vi "LabVIEW_Ansys.vi"() -> ()   [LabVIEW 2017]
uses:
  <vilib>/imath/engines/lvmath/Plug In/_Char/NIMS_CH_character datatype.ctl
  <vilib>/Utility/file.llb/Read Delimited Spreadsheet (string).vi
  <vilib>/imath/engines/lvmath2/RunTimeEngine/Managers/WorkSpace/UID Generator.vi
  <vilib>/imath/engines/lvmath2/RunTimeEngine/ArithmeticOperatorToken/NIMS_ArithmeticOperator_times.vi
  <instcachedir>/0/NIMS_ArithmeticOperator_times_9BECD6C28351466A83A029AF2762CD58.lvgen/NIMS_ArithmeticOperator_times_9BECD6C28351466A83A029AF2762CD58_000.vi
  <vilib>/imath/engines/lvmath2/RunTimeEngine/ArithmeticOperatorToken/NIMS_ArithmeticOperator_plus.vi
  <instcachedir>/0/NIMS_ArithmeticOperator_plus_9255C7DA94A9479C92F91DC2DA9A664F.lvgen/NIMS_ArithmeticOperator_plus_9255C7DA94A9479C92F91DC2DA9A664F_004.vi
  <vilib>/imath/engines/lvmath2/RunTimeEngine/RunTimeType/NIMS_RunTimeType_From StrictType (excl LVString).vi
  <instcachedir>/0/NIMS_RunTimeType_From StrictType (excl LVString)_1019F277F0A747EDBCA0F6C52CA54500.lvgen/NIMS_RunTimeType_From StrictType (excl LVString)_1019F277F0A747EDBCA0F6C52CA54500_000.vi
  <vilib>/imath/engines/lvmath2/RunTimeEngine/ErrorHandling/NIMS_Create Error From Enums.vi
  <vilib>/imath/engines/lvmath2/RunTimeEngine/LocalVariableDefStatement/MC_LocalVariableDefStatement_Display.vi
  <vilib>/imath/engines/lvmath2/RunTimeEngine/BuiltInFunctions/plot/NIMS_plot(RM, RM, Str).vi
  <vilib>/imathl/engines/lvmath/Functions/Error Handling/Create Error.vi
  <vilib>/imath/engines/lvmath/Plug In/_Char/NIMS_CH_Character RV to String.vi
  <vilib>/imath/engines/lvmath2/RunTimeEngine/BuiltInFunctions/title/NIMS_title.vi
  <vilib>/imath/engines/lvmath2/RunTimeEngine/BuiltInFunctions/xlabel/NIMS_xlabel.vi
  <vilib>/imath/engines/lvmath2/RunTimeEngine/BuiltInFunctions/ylabel/NIMS_ylabel.vi
  <vilib>/imath/engines/lvmath2/RunTimeEngine/Managers/SymbolTable/Clear UID.vi
  <vilib>/imath/engines/lvmath2/RunTimeEngine/ErrorHandling/NIMS_Finalize Error.vi
  <vilib>/imath/engines/lvmath2/RunTimeEngine/Managers/SymbolTable/NIMS_WorkSpace.lvlib
panel:
  in  "定子瞬态":bool
  out "new picture":picture caption="图片展示"
  in  "?":bool
  in  "表面幅仿真-Z方向":bool
  in  "表面幅仿真-Y方向":bool
  in  "关闭图片":bool
  in  "阻抗特性曲线":bool
  in  "计算步数":u32(slide) scale=0.0..100.0
  in  "表面幅仿真-X方向":bool
  in  "16":bool
  in  "波数":dbl
  in  "15":bool
  in  "台阶高":dbl
  in  "14":bool
  in  "压电片外圈直径":dbl
  in  "13":bool
  in  "压电片内圈直径":dbl
  in  "12":bool
  in  "压电片厚":dbl
  in  "11":bool
  in  "轴厚度":dbl
  in  "10":bool
  in  "轴外圈直径":dbl
  in  "9":bool
  in  "轴内圈直径":dbl
  in  "8":bool
  in  "定子齿外圈直径":dbl
  in  "7":bool
  in  "定子齿内圈直径":dbl
  in  "6":bool
  in  "齿槽宽":dbl
  in  "5":bool
  in  "齿厚":dbl
  in  "4":bool
  in  "内侧斜齿高":dbl
  in  "3":bool
  in  "外侧斜齿高":dbl
  in  "2":bool
  in  "平均齿高":dbl
  in  "1":bool
  in  "齿数":dbl
  in  "数值":dbl
  in  "加载图片":bool
  in  "一键删除":bool
  in  "开始ANSYS计算":bool
  in  "存":bool
  in  "前一张":bool
  in  "后一张":bool
  # "电机仿真参数"
  # "计算"
  # "结果"
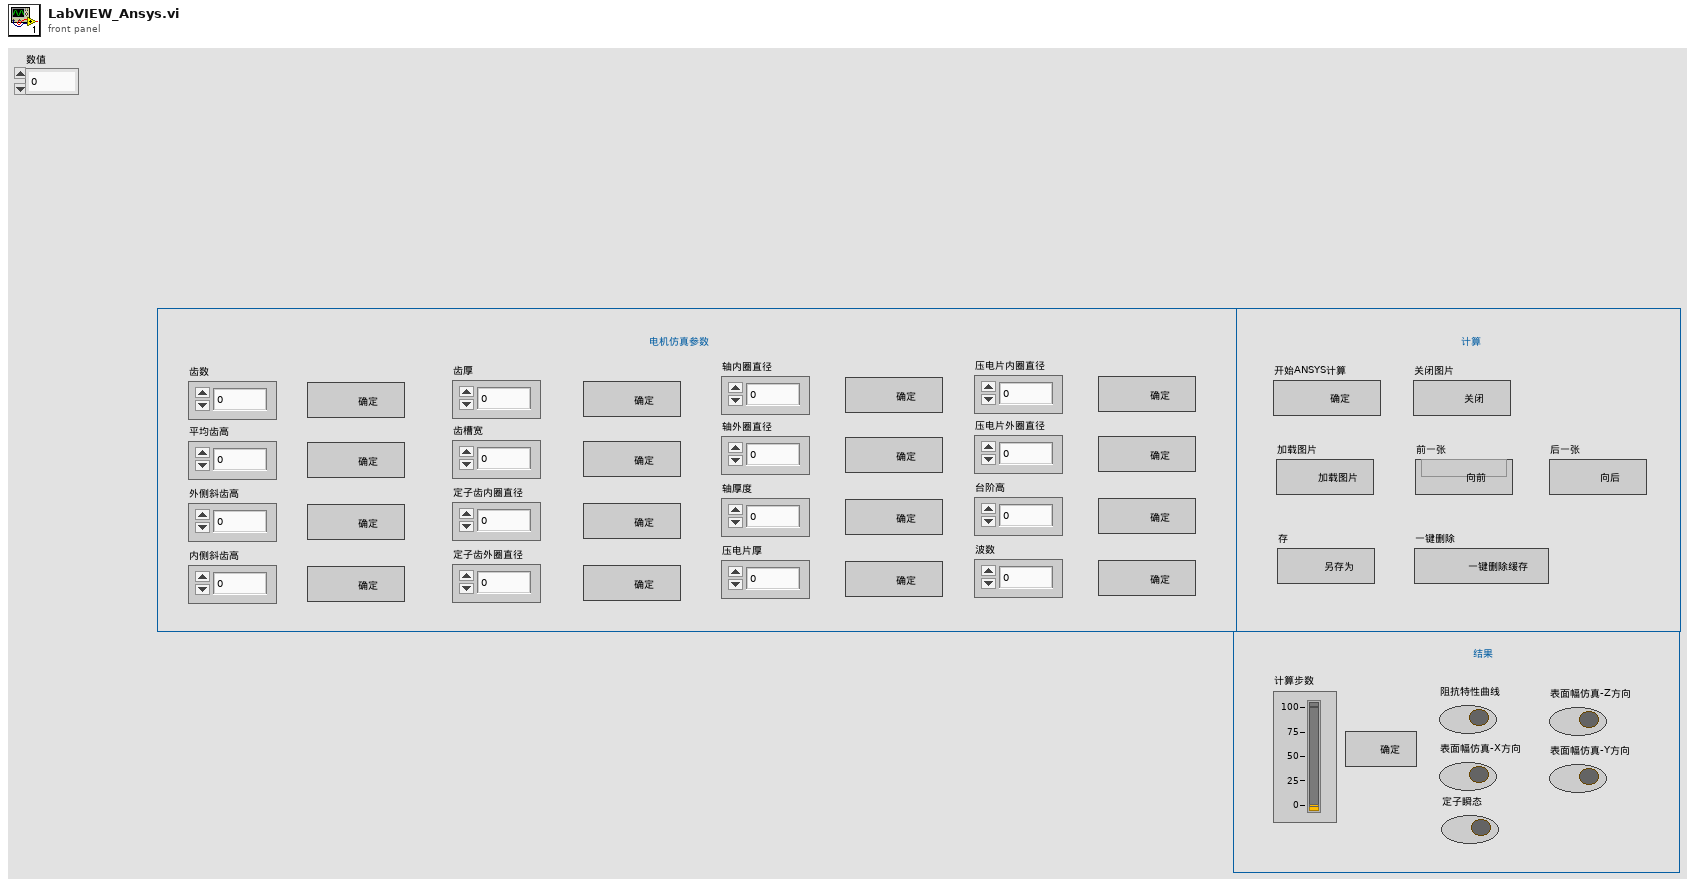
[diagram p1: front panel]
types:
  T1 = enum16{"open", "replace", "create", "open or create", "replace or create", "replace or create with confirmation"}
  T2 = typedef "NIMS_CH_character datatype.ctl" = cluster{"Numeric":u8}
  T3 = typedef "imagedata.ctl" = cluster{"image type":i32, "image depth":i32, "image":u8[], "mask":u8[], "colors":u32[], "Rectangle":cluster{"left":i16, "top":i16, "right":i16, "bottom":i16}}
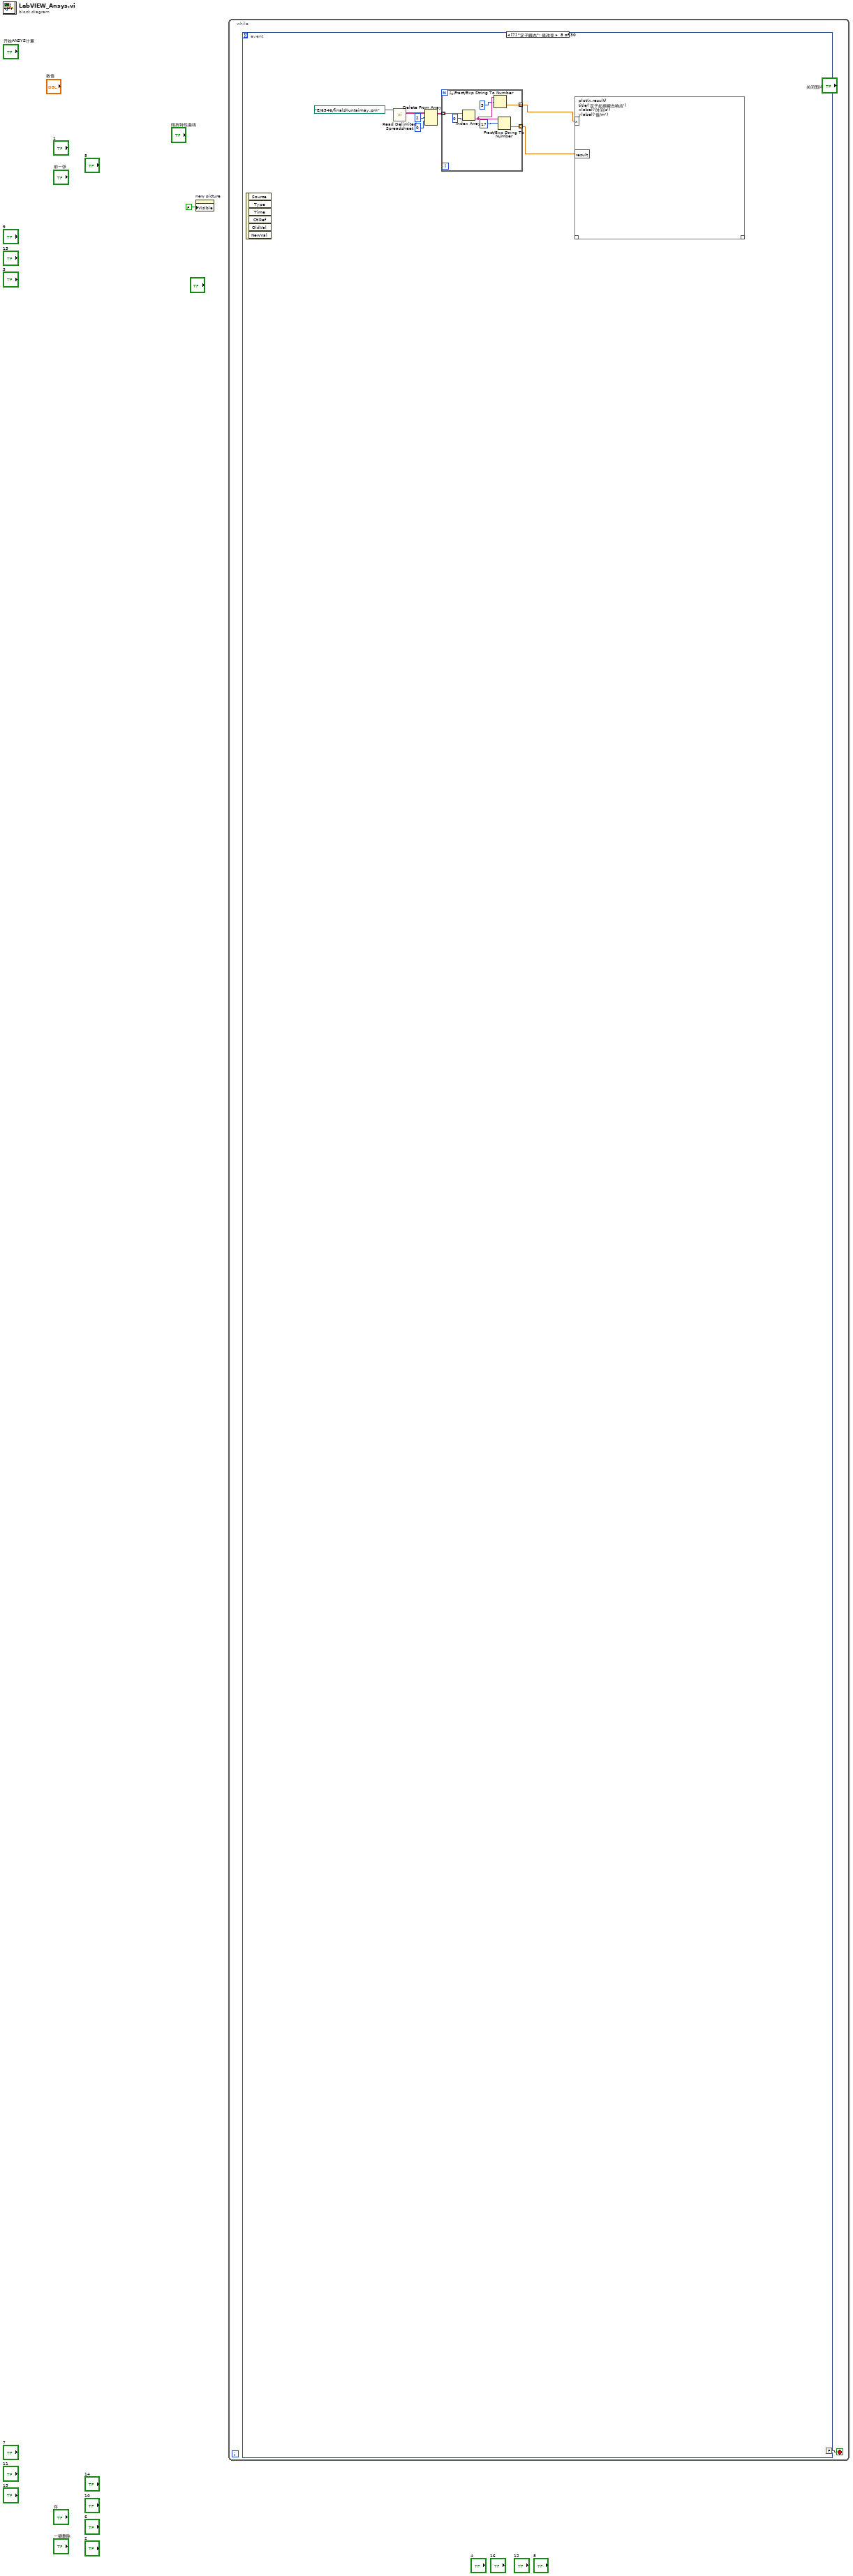
[diagram p0: block diagram]
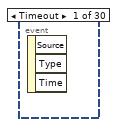
[diagram p2: hidden frame]
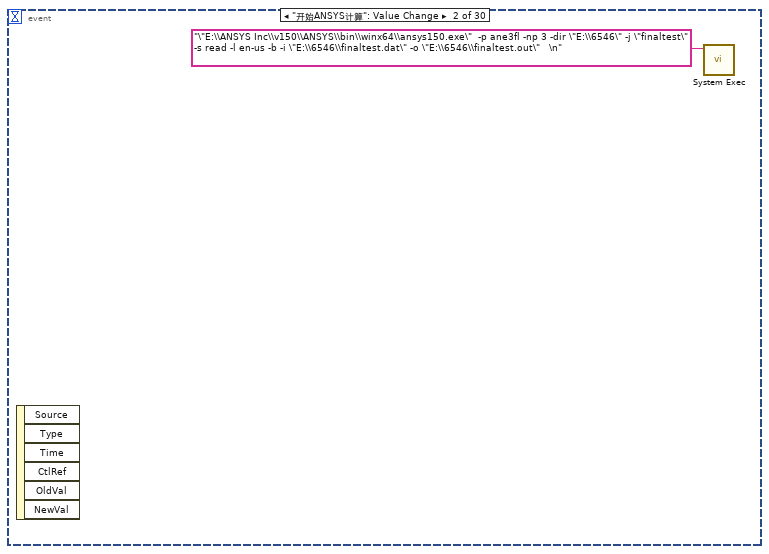
[diagram p3: hidden frame]
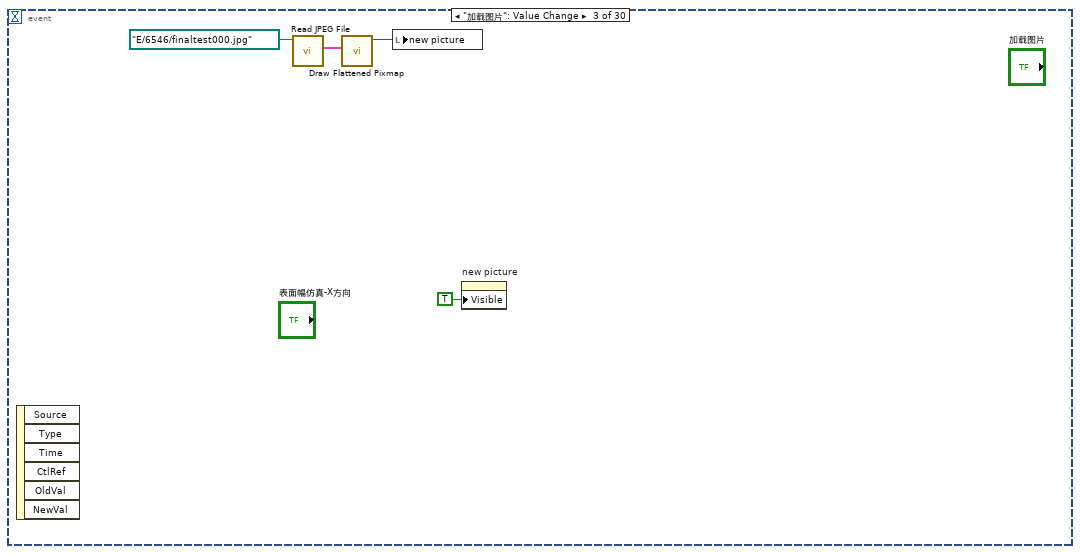
[diagram p4: hidden frame]
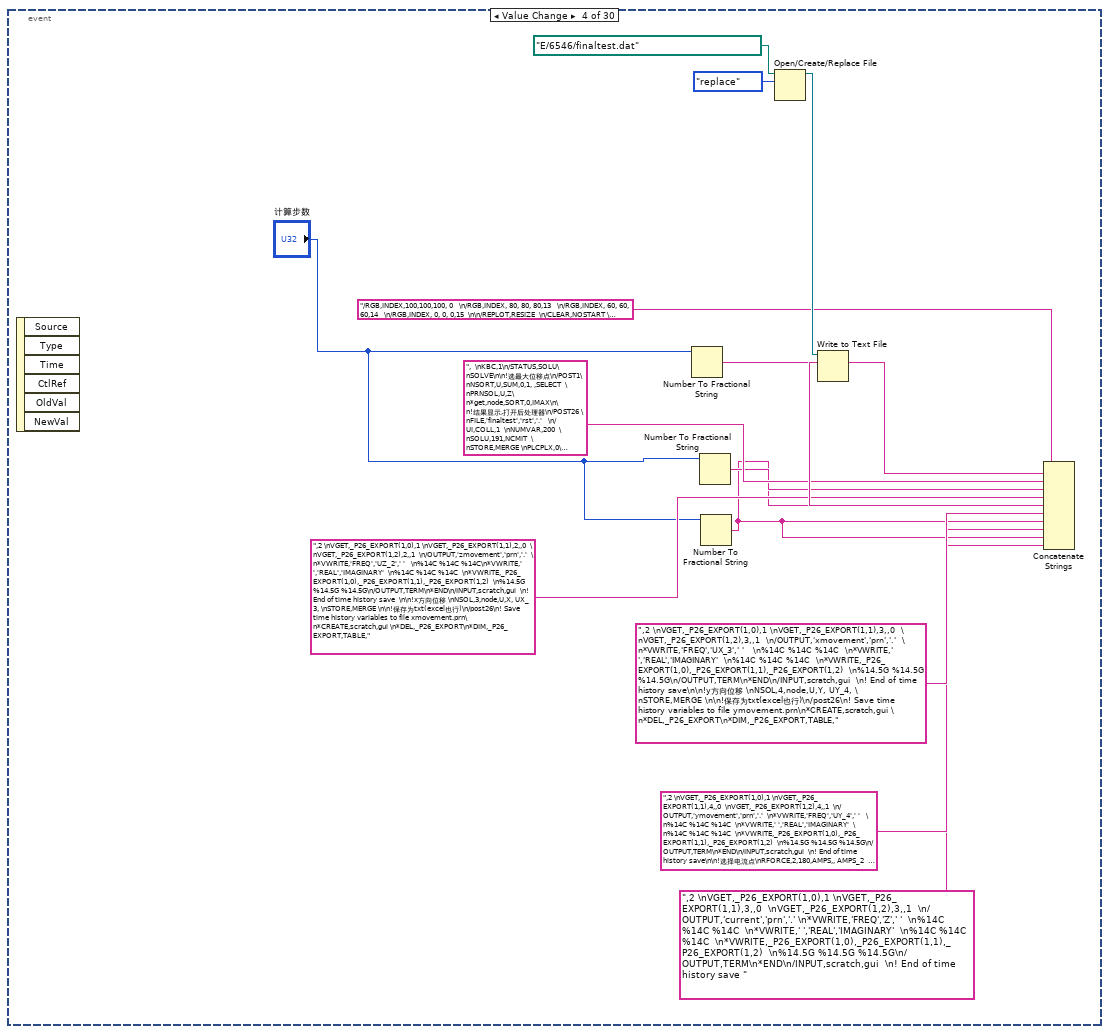
[diagram p5: hidden frame]
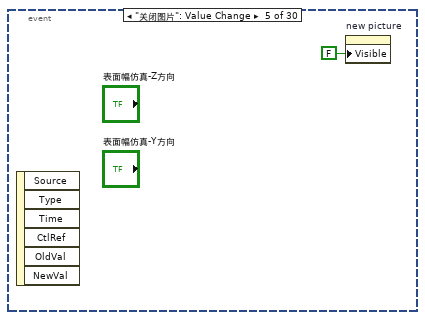
[diagram p6: hidden frame]
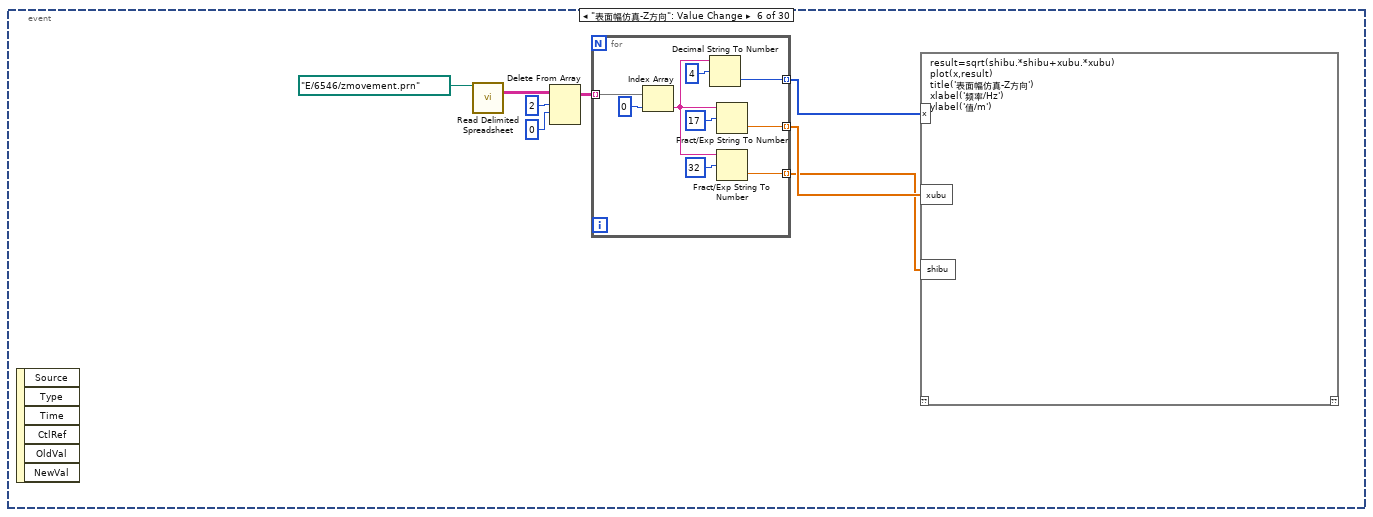
[diagram p7: hidden frame]
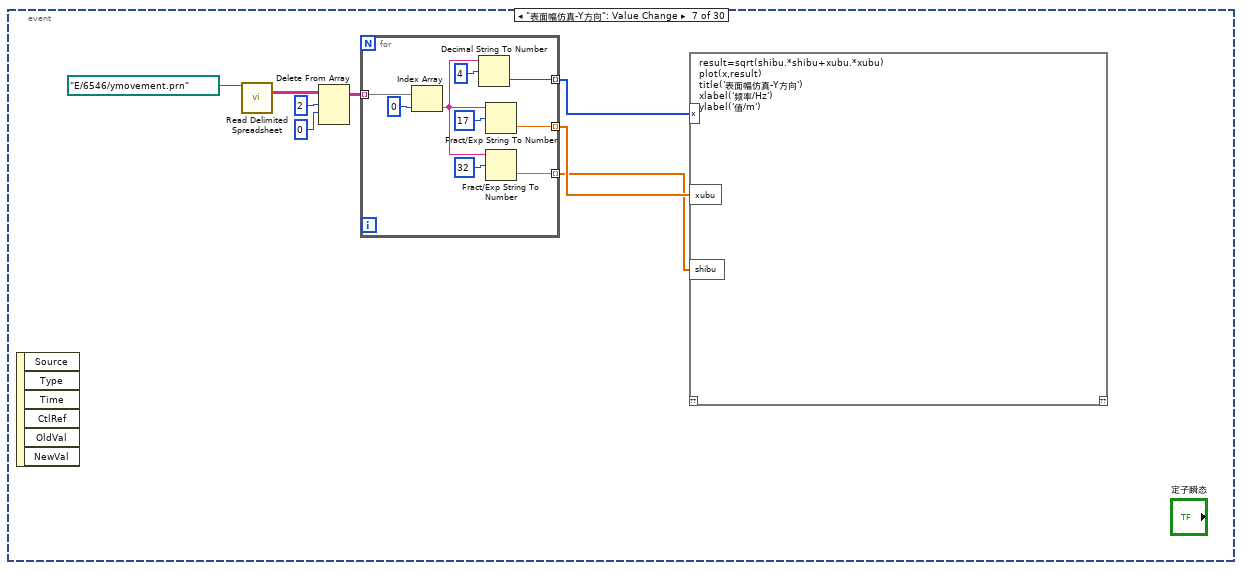
[diagram p8: hidden frame]
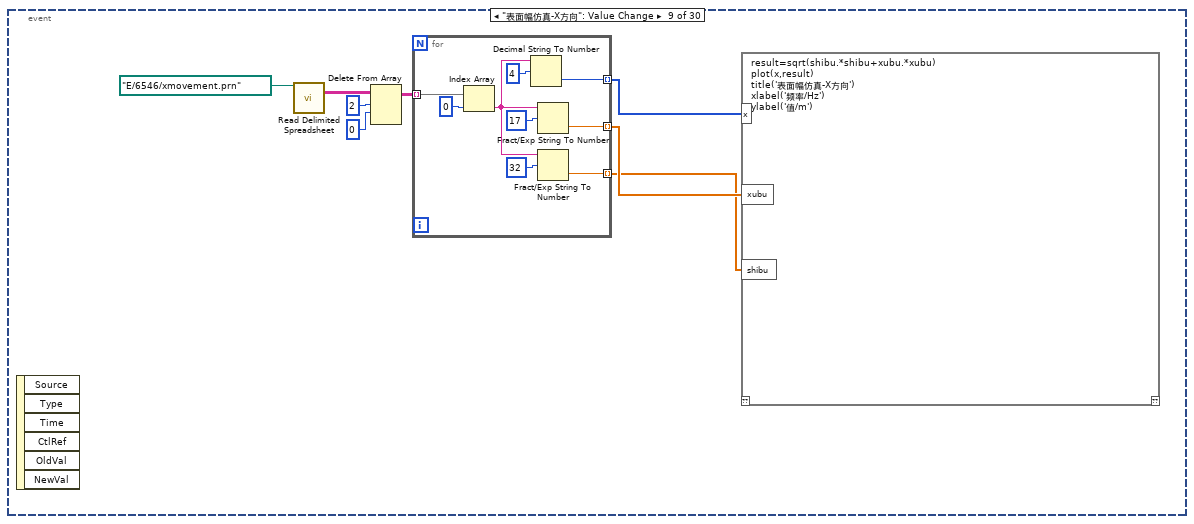
[diagram p9: hidden frame]
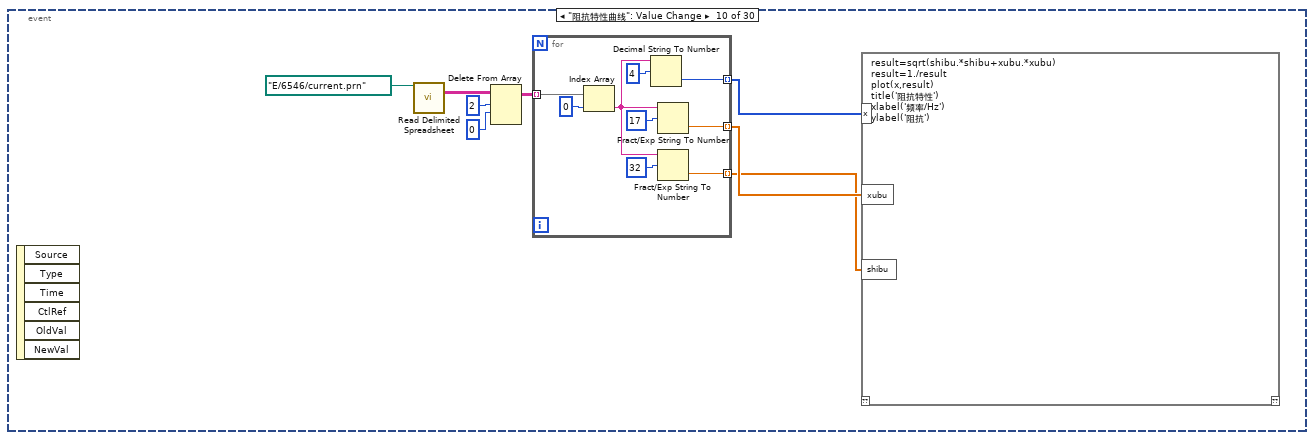
[diagram p10: hidden frame]
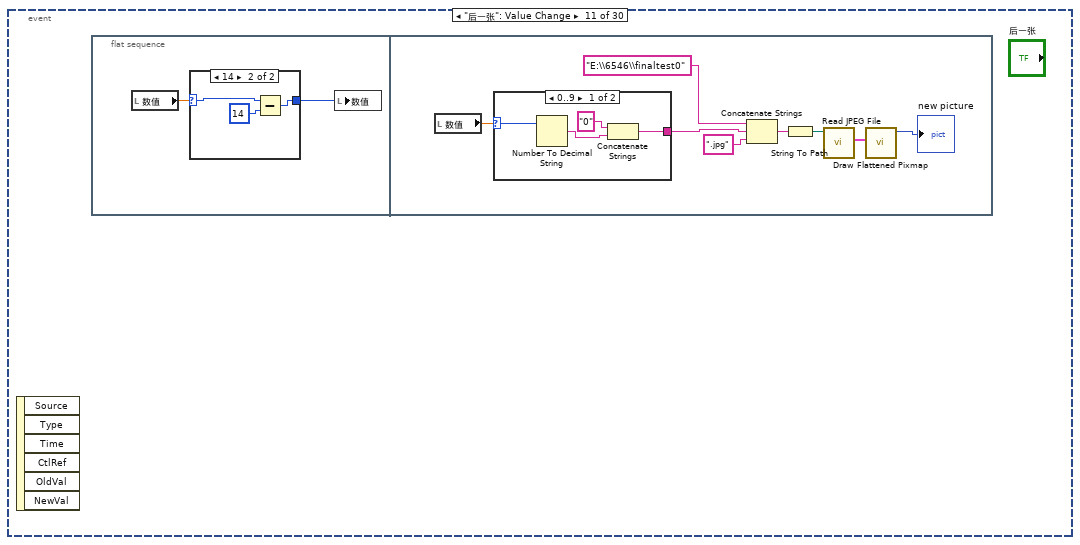
[diagram p11: hidden frame]
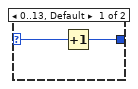
[diagram p12: hidden frame]
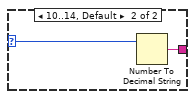
[diagram p13: hidden frame]
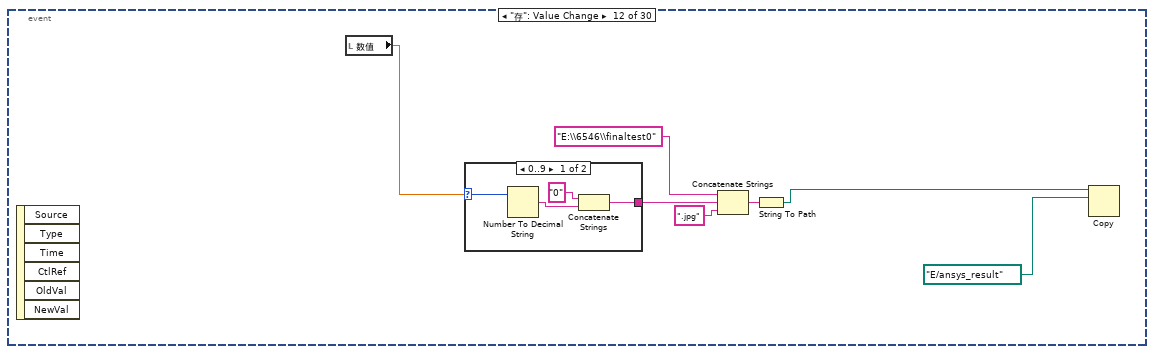
[diagram p14: hidden frame]
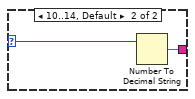
[diagram p15: hidden frame]
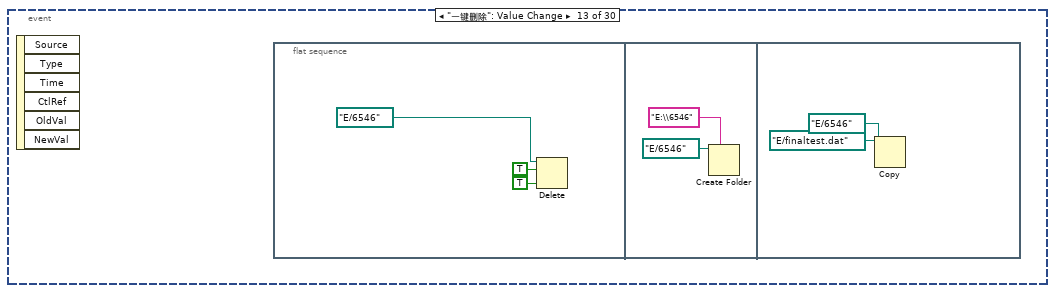
[diagram p16: hidden frame]
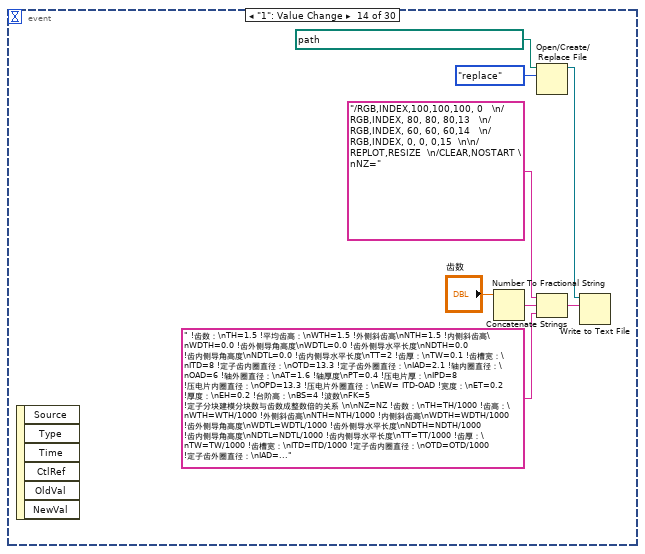
[diagram p17: hidden frame]
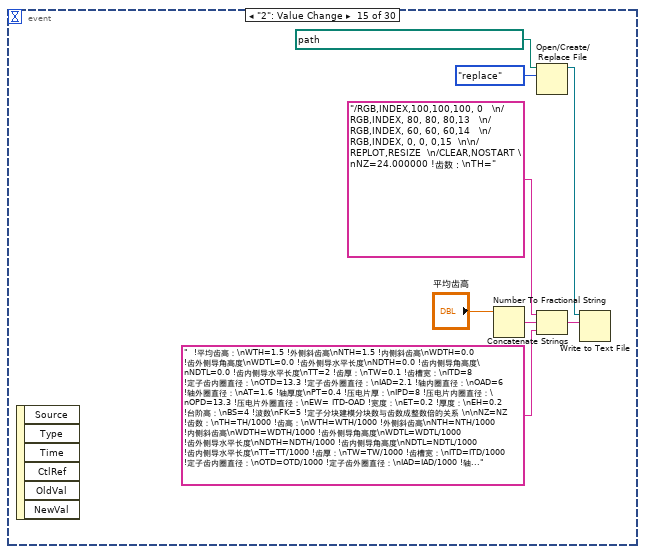
[diagram p18: hidden frame]
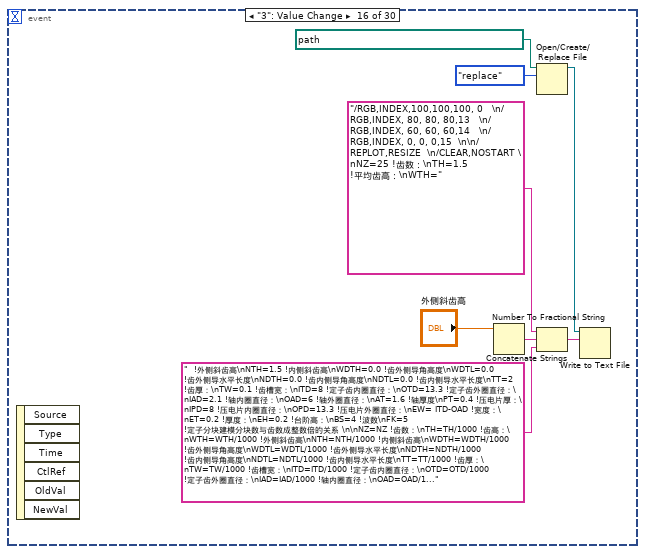
[diagram p19: hidden frame]
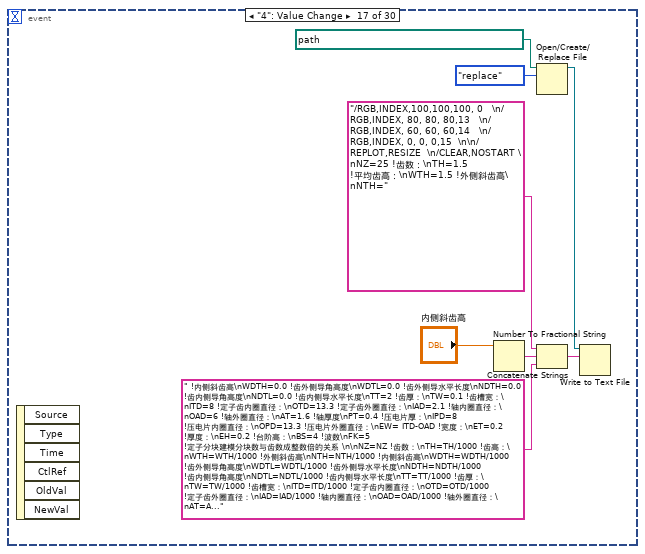
[diagram p20: hidden frame]
diagram:
  n1 = property on="new picture" class="Pict"("Visible"=FALSE ("可见")) -> ()  [unwired: 2 in, 2 out]
  n2 = while {
    stop <- FALSE stop-if-true
    n3 = event shown="[7] \"定子瞬态\": 值改变" {
      selector: _ -> [_ _ _ _ _ _ _ _ _ _ _ _ _ _ _ _ _ _ _ _ _ _ _ _ _ _ _ _ _ _]
      dyn-events: _ -> [_ _ _ _ _ _ _ _ _ _ _ _ _ _ _ _ _ _ _ _ _ _ _ _ _ _ _ _ _ _]
      timeout: _ -> [_ _ _ _ _ _ _ _ _ _ _ _ _ _ _ _ _ _ _ _ _ _ _ _ _ _ _ _ _ _]
      event Timeout {
        n4 = event-data() -> ()  [unwired: 1 in, 3 out]
      }
      event "开始ANSYS计算": Value Change {
        n5 = event-data() -> ()  [unwired: 1 in, 6 out]
        n6 = call <vilib>:"System Exec.vi"("command line"="\"E:\\ANSYS Inc\\v150\\ANSYS\\bin\\winx64\\ansys150.exe\"  -p ane3fl -np 3 -dir \"E:\\6546\" -j \"finaltest\" -s read -l en-us -b -i \"E:\\6546\\finaltest.dat\" -o \"E:\\6546\\finaltest.out\"   \n") -> ()  [unwired: 7 in, 4 out]
      }
      event "加载图片": Value Change {
        n7 = event-data() -> ()  [unwired: 1 in, 6 out]
        n8 = call <vilib>:"Read JPEG File.vi"("path to JPEG file"=path "E:/6546/finaltest000.jpg") -> ("image data"=w7:T3)  [unwired: 8 in, 2 out]
        n9 = call <vilib>:"Draw Flattened Pixmap.vi"("image data"=w7) -> ("new picture"=w5:picture)  [unwired: 8 in]
        n10 = local write "new picture"(w5) -> ()
        n11 = property on="new picture" class="Pict"("Visible"=TRUE ("可见")) -> ()  [unwired: 2 in, 2 out]
      }
      event Value Change {
        n12 = event-data() -> ()  [unwired: 1 in, 6 out]
        n13 = Number To Fractional String(number="计算步数") -> (F-format string=w17:string)  [unwired: 3 in]
        n14 = Number To Fractional String(number="计算步数") -> (F-format string=w14:string)  [unwired: 3 in]
        n15 = Number To Fractional String(number="计算步数") -> (F-format string=w9:string)  [unwired: 3 in]
        n16 = Open/Create/Replace File(file path (use dialog)=path "E:/6546/finaltest.dat" ("文件路径（使用对话框）"), operation (0:open)=T1."replace" ("操作(0:open)")) -> (refnum out=w21:refnum<file>)  [unwired: 4 in, 2 out]
        n17 = Concatenate Strings("/RGB,INDEX,100,100,100, 0   \n/RGB,INDEX, 80, 80, 80,13   \n/RGB,INDEX, 60, 60, 60,14   \n/RGB,INDEX, 0, 0, 0,15  \n\n/REPLOT,RESIZE  \n/CLEAR,NOSTART \nNZ=25 !齿数：\nTH=1.5 !平均齿高：\nWTH=1.5 !外侧斜齿高\nNTH=1.5 !内侧斜齿高\nWDTH=0.0 !齿外侧导角高度\nWDTL=0.0 !齿外侧导水平长度\nNDTH=0.0 !齿内侧导角高度\nNDTL=0.0 !齿内侧导水平长度\nTT=2 !齿厚：\nTW=0.1 !齿槽宽：\nITD=8 !定子齿内圈直径：\nOTD=13.3 !定子齿外圈直径：\nIAD=2.1 !轴内圈直径：\nOAD=6 !轴外圈直径：\nAT=1.6 !轴厚度\nPT=0.4 !压电片厚：\nIPD=8 !压电片内圈直径：\nOPD=13.3 !压电片外圈直径：\nEW= ITD-OAD !宽度：\nET=0.2 !厚度：\nEH=0.2 !台阶高：\nBS=4 !波数\nFK=5 !定子分块建模分块数与齿数成整数倍的关系 \n\nNZ=NZ !齿数：\nTH=TH/1000 !齿高：\nWTH=WTH/1000 !外侧斜齿高\nNTH=NTH/1000 !内侧斜齿高\nWDTH=WDTH/1000 !齿外侧导角高度\nWDTL=WDTL/1000 !齿外侧导水平长度\nNDTH=NDTH/1000 !齿内侧导角高度\nNDTL=NDTL/1000 !齿内侧导水平长度\nTT=TT/1000 !齿厚：\nTW=TW/1000 !齿槽宽：\nITD=ITD/1000 !定子齿内圈直径：\nOTD=OTD/1000 !定子齿外圈直径：\nIAD=IAD/1000 !轴内圈直径：\nOAD=OAD/1000 !轴外圈直径：\nAT=AT/1000 !轴厚度\nPT=PT/1000 !压电片厚：\nIPD=IPD/1000 !压电片内圈直径：\nOPD=OPD/1000 !压电片外圈直径：\nEW= EW/1000 !宽度：\nET=ET/1000 !厚度：\nEH=EH/1000 !台阶高：\n\n/PREP7 \n!定义单元和材料属性\nET,1,SOLID185   \nMPTEMP,,,,,,,,  \nMPTEMP,1,0  \nMPDATA,DENS,1,,8290\nMPTEMP,,,,,,,,  \nMPTEMP,1,0  \nMPDATA,EX,1,,1.06E+011   \nMPDATA,PRXY,1,,0.35 \n\nET,2,SOLID5 \nMPTEMP,,,,,,,,  \nMPTEMP,1,0     \nMPDATA,DENS,2,,7750   \nMPTEMP,,,,,,,,  \nMPTEMP,1,0  \nMPDATA,PERX,2,,919E-009\nMPDATA,PERY,2,,919E-009   \nMPDATA,PERZ,2,,826E-009\nTB,PIEZ,2,,,0   \nTBMODIF,1,1,0   \nTBMODIF,1,2,0   \nTBMODIF,1,3,-5.35   \nTBMODIF,2,1,0   \nTBMODIF,2,2,0   \nTBMODIF,2,3,-5.35   \nTBMODIF,3,1,0   \nTBMODIF,3,2,0   \nTBMODIF,3,3,15.78   \nTBMODIF,4,1,0   \nTBMODIF,4,2,0   \nTBMODIF,4,3,0   \nTBMODIF,5,1,0   \nTBMODIF,5,2,12.3\nTBMODIF,5,3,0   \nTBMODIF,6,1,12.3\nTBMODIF,6,2,0   \nTBMODIF,6,3,0   \nTB,ANEL,2,1,21,0\nTBTEMP,0\nTBDATA,,1.2035E+011,7.52E+010,7.51E+010,0,0,0   \nTBDATA,,1.204E+011,7.51E+010,0,0,0,1.109E+011   \nTBDATA,,0,0,0,2.26E+010,0,0 \nTBDATA,,2.12E+010,0,2.11E+010,,,\n\n!超声波电机模型建立\nK,1,OAD/2,,,\nK,2,ITD/2,,,\nK,3,ITD/2,-EH,,!最上面\nK,4,OTD/2,-EH,,\nK,5,OTD/2,-EH+TT-TH,,\nK,6,ITD/2,-EH+TT-TH,,\nK,7,ITD/2,ET,,\nK,8,OAD/2,ET,,\nK,11,ITD/2,-EH-PT,,!最下面\nK,12,OTD/2,-EH-PT,,\nK,13,OTD/2,-EH+TT,,\nK,14,ITD/2,-EH+TT,,\nK,15,IAD/2,ET,,\nK,16,IAD/2,0,,\nK,17,IAD/2,-AT+ET,,\nK,18,OAD/2,-AT+ET,,\n\nK,100,0,0,0,\nK,101,0,0.003,0,\n\nLSTR,1,2\nLSTR,2,3\nLSTR,3,4\nLSTR,4,5\nLSTR,5,6\nLSTR,6,7\nLSTR,7,8\nLSTR,8,1\nLSTR,3,11\nLSTR,11,12\nLSTR,12,4\nLSTR,5,13\nLSTR,13,14\nLSTR,14,6\nLSTR,2,7\nLSTR,8,15\nLSTR,15,16\nLSTR,1,16\nLSTR,16,17\nLSTR,17,18\nLSTR,1,18\n\nAL,1,15,7,8\nAL,15,2,3,4,5,6,\nAL,9,10,11,3\nAL,5,12,13,14\nAL,8,16,17,18\nAL,18,19,20,21\n\nVROTAT,1,2,3,4, , ,100,101 ,360/FK, , !!!!!\nVROTAT,5,6, , , , ,100,101 ,360/FK, , !!!!!\nBLC4,0,TT-EH,OTD,-TH,TW !建立长方体\nVGEN, ,7, , , , ,-TW/2, , ,1!复制创建体  \nVOVLAP,4,7 !布尔操作\nVDELE,10, , ,1!删除体\nVSYMM,Z,8, , , ,0,0 !体镜像 \n\n!建立齿槽\nCSYS,5  \nWPSTYLE,,,,,,,,0\nVGEN,NZ/FK+1,4, , , ,360/NZ, , ,0  \nVGEN,NZ/FK+1,8, , , ,360/NZ, , ,0  \nVOVLAP,ALL\n*DO,I,1,NZ/FK+1\nCSYS,0\nVSEL,S,LOC,Y,TT-EH-TH/1.5,1\nCSYS,5\nVSEL,R,LOC,Y,(I-1)*360/NZ-TW/2/3.1415/ITD*360,TW/2/3.1415/ITD*360+(I-1)*360/NZ!选择体\nVDELE,ALL, , ,1\nALLSEL,ALL \n*ENDDO\n\n!旋转成体\nEPLOT \nCSYS,5 \nVGEN,FK,ALL, , , ,360/FK, , ,0 \n\n!Glue体\nVGLUE,ALL\n\n!添加材料属性\nALLSEL,ALL\nCSYS,0\nVSEL,S,LOC,Y,0,TT-EH\nVATT,       1, ,   1,       0   \nCSYS,5\nVSEL,S,LOC,X,0,OAD/2\nVATT,       1, ,   1,       0 \n\nALLSEL,ALL\nCSYS,0\nVSEL,R,LOC,Y,-EH-PT,-EH\nVATT,       2, ,  2,       0  \nALLSEL,ALL\n\n!网格体\nCSYS,0\nVSEL,R,LOC,Y,-EH-PT,-EH\nVSWEEP,ALL\n\nCSYS,0\nALLSEL,ALL \nVSEL,S,MAT,,1\nSMRT,6  \nSMRT,5  \nSMRT,4  \nMSHAPE,1,3d\nMSHKEY,0\nVMESH,ALL\n\nALLSEL,ALL\n\n!模态分析 \n/SOL  \nANTYPE,2\nMODOPT,LANB,22  \nEQSLV,SPAR  \nMXPAND,0, , ,0  \nLUMPM,0 \nPSTRES,0\nMODOPT,LANB,22,0,80000, ,OFF\n\nCSYS,5\nASEL,S,LOC,X,-IAD/2,IAD/2   \nDA,ALL,ALL,\nALLSEL,ALL\n\n!OUTPR,BASIC,ALL,  \n!OUTRES,ALL,ALL,\n \n/STATUS,SOLU\nSOLVE   \nFINISH\nCSYS,0\nALLSEL,ALL\n\n/POST1  \nSET,FIRST   \n/EFACET,1   \nPLNSOL, U,SUM, 2,1.0 !无轮廓2变0\n/post1\n*do,i,8,22\nset,1,i\n/VIEW,1,1,2,3   \n/ANG,1  \n/REP,FAST  \n/show,jpeg,,\nplnsol,u,sum,0,1.0\n/show,close\n*enddo\nFINISH\n\n!振幅仿真\n/SOL\nANTYPE,3\nHROPT,FULL  \nHROUT,ON\nLUMPM,0 \nEQSLV, ,0,  \nPSTRES,0\n\n!阻尼特性\nALPHAD,0,   \nBETAD,0,\nDMPSTR,0.005,   \n\n!压电耦合\n*do,i,1,(BS-1)\nALLSEL,ALL\ncsys,5\nnsel,S,LOC,X,ITD/2,OTD/2\ncsys,0\nnsel,R,loc,y,-eh-eq-pt\ncsys,5\nangle=360/BS\nnsel,r,loc,y,(i-1)*angle/2,i*angle/2\nb=1/2*(1-(-1)**i)*1\nc=1/2*(1-(-1)**(i+1))*1\nD,All,VOLT,b,c\n*enddo\n\nALLSEL,ALL\ncsys,5\nnsel,S,LOC,X,ITD/2,OTD/2\ncsys,0\nnsel,R,loc,y,-eh-eq-pt\ncsys,5\nangle=360/BS\nnsel,r,loc,y,(BS-1)*angle/2,((BS-1)*angle/2+3*angle/8)\nD,All,VOLT,(1/2*(1-(-1)**BS)*1),(1/2*(1-(-1)**(BS+1))*1)\n\nALLSEL,ALL\ncsys,5\nnsel,S,LOC,X,ITD/2,OTD/2\ncsys,0\nnsel,R,loc,y,-eh-eq-pt\ncsys,5\nangle=360/BS\nnsel,r,loc,y,((BS-1)*angle/2+3*angle/8),((BS-1)*angle/2+3*angle/4)\nD,All,VOLT,(1/2*(1-(-1)**(BS+1))*1),(1/2*(1-(-1)**(BS+2))*1)\n\n*do,i,1,(BS-1)\nALLSEL,ALL\ncsys,5\nnsel,S,LOC,X,ITD/2,OTD/2\ncsys,0\nnsel,R,loc,y,-eh-eq-pt\ncsys,5\nangle=360/BS\nnsel,r,loc,y,((BS-1)*angle/2+3*angle/4+(i-1)*angle/2),((BS-1)*angle/2+3*angle/4+(i)*angle/2)\ne=1/2*(1-(-1)**(BS+1+i))*1\nf=1/2*(1-(-1)**(BS+2+i))*1\nD,All,VOLT,e,f\n*enddo\n\nALLSEL,ALL\ncsys,5\nnsel,S,LOC,X,ITD/2,OTD/2\ncsys,0\nnsel,r,loc,y,-eh-eq\nD,All,VOLT,0,0\nALLSEL,ALL \n\nHARFRQ,26000,76000, \nNSUBST," ("字符串"), w17, ",  \nKBC,1\n/STATUS,SOLU\nSOLVE\n\n!选最大位移点\n/POST1\nNSORT,U,SUM,0,1, ,SELECT  \nPRNSOL,U,Z\n*get,node,SORT,0,IMAX\n\n!结果显示,打开后处理器\n/POST26 \nFILE,'finaltest','rst','.'   \n/UI,COLL,1  \nNUMVAR,200  \nSOLU,191,NCMIT  \nSTORE,MERGE \nPLCPLX,0\nPRCPLX,1\nFILLDATA,191,,,,1,1 \nREALVAR,191,191 \n\n!z方向位移 \nNSOL,2,node,U,Z, UZ_2, \nSTORE,MERGE \n\n!保存为txt(excel也行)\n/post26\n! Save time history variables to file zmovement.prn\n*CREATE,scratch,gui \n*DEL,_P26_EXPORT\n*DIM,_P26_EXPORT,TABLE," ("字符串"), w14, ",2 \nVGET,_P26_EXPORT(1,0),1 \nVGET,_P26_EXPORT(1,1),2,,0  \nVGET,_P26_EXPORT(1,2),2,,1  \n/OUTPUT,'zmovement','prn','.'  \n*VWRITE,'FREQ','UZ_2',' '   \n%14C %14C %14C\n*VWRITE,' ','REAL','IMAGINARY'  \n%14C %14C %14C  \n*VWRITE,_P26_EXPORT(1,0),_P26_EXPORT(1,1),_P26_EXPORT(1,2)  \n%14.5G %14.5G %14.5G\n/OUTPUT,TERM\n*END\n/INPUT,scratch,gui  \n! End of time history save  \n\n!x方向位移 \nNSOL,3,node,U,X, UX_3, \nSTORE,MERGE \n\n!保存为txt(excel也行)\n/post26\n! Save time history variables to file xmovement.prn\n*CREATE,scratch,gui \n*DEL,_P26_EXPORT\n*DIM,_P26_EXPORT,TABLE," ("字符串"), w9, ",2 \nVGET,_P26_EXPORT(1,0),1 \nVGET,_P26_EXPORT(1,1),3,,0  \nVGET,_P26_EXPORT(1,2),3,,1  \n/OUTPUT,'xmovement','prn','.'  \n*VWRITE,'FREQ','UX_3',' '   \n%14C %14C %14C  \n*VWRITE,' ','REAL','IMAGINARY'  \n%14C %14C %14C  \n*VWRITE,_P26_EXPORT(1,0),_P26_EXPORT(1,1),_P26_EXPORT(1,2)  \n%14.5G %14.5G %14.5G\n/OUTPUT,TERM\n*END\n/INPUT,scratch,gui  \n! End of time history save\n\n!y方向位移 \nNSOL,4,node,U,Y, UY_4, \nSTORE,MERGE \n\n!保存为txt(excel也行)\n/post26\n! Save time history variables to file ymovement.prn\n*CREATE,scratch,gui \n*DEL,_P26_EXPORT\n*DIM,_P26_EXPORT,TABLE," ("字符串"), w9, ",2 \nVGET,_P26_EXPORT(1,0),1 \nVGET,_P26_EXPORT(1,1),4,,0  \nVGET,_P26_EXPORT(1,2),4,,1  \n/OUTPUT,'ymovement','prn','.'  \n*VWRITE,'FREQ','UY_4',' '   \n%14C %14C %14C  \n*VWRITE,' ','REAL','IMAGINARY'  \n%14C %14C %14C  \n*VWRITE,_P26_EXPORT(1,0),_P26_EXPORT(1,1),_P26_EXPORT(1,2)  \n%14.5G %14.5G %14.5G\n/OUTPUT,TERM\n*END\n/INPUT,scratch,gui  \n! End of time history save\n\n!选择电流点\nRFORCE,2,180,AMPS,, AMPS_2  \nSTORE,MERGE \nFILLDATA,192,,,,0,0 \nFILLDATA,193,,,,1,0 \nFILLDATA,194,,,,-1,0\nFILLDATA,195,,,,1,1 \nVARNAME,195,NSET\n! Name: Z   \n! ID:  3\n! Function: 1/{AMPS_2}  \nFILLDATA,199,,,,1,0 \nREALVAR,199,199 \nQUOT,3,199,2,,Z \nSTORE,MERGE \n\n!保存为txt(excel也行)\n/post26\n! Save time history variables to file current.prn   \n*CREATE,scratch,gui \n*DEL,_P26_EXPORT\n*DIM,_P26_EXPORT,TABLE," ("字符串"), w9, ",2 \nVGET,_P26_EXPORT(1,0),1 \nVGET,_P26_EXPORT(1,1),3,,0  \nVGET,_P26_EXPORT(1,2),3,,1  \n/OUTPUT,'current','prn','.' \n*VWRITE,'FREQ','Z',' '  \n%14C %14C %14C  \n*VWRITE,' ','REAL','IMAGINARY'  \n%14C %14C %14C  \n*VWRITE,_P26_EXPORT(1,0),_P26_EXPORT(1,1),_P26_EXPORT(1,2)  \n%14.5G %14.5G %14.5G\n/OUTPUT,TERM\n*END\n/INPUT,scratch,gui  \n! End of time history save " ("字符串")) -> (w20:string)
        n18 = Write to Text File(file (use dialog)=w21, text=w20) -> ()  [unwired: 2 in, 3 out]
      }
      event "关闭图片": Value Change {
        n19 = event-data() -> ()  [unwired: 1 in, 6 out]
        n20 = property on="new picture" class="Pict"("Visible"=FALSE ("可见")) -> ()  [unwired: 2 in, 2 out]
      }
      event "表面幅仿真-Z方向": Value Change {
        n21 = event-data() -> ()  [unwired: 1 in, 6 out]
        n22 = call-poly <vilib>:"Read Delimited Spreadsheet.vi"("file path (dialog if empty)"=path "E:/6546/zmovement.prn") -> ("all rows"=w27:string[][])  [unwired: 9 in, 5 out]
        n23 = Delete From Array(array=w27, length=2 ("长度"), index (row)=0 ("索引 (行)")) -> (array with subset deleted=w26:string[][])  [unwired: 1 in, 1 out]
        n24 = for {
          tunnel: w26 -> [w175] mode=indexing
          tunnel: [w178] -> w24 mode=indexing
          tunnel: [w177] -> w23 mode=indexing
          tunnel: [w176] -> w25 mode=indexing
          n25 = Index Array(array=w175, index=0 ("索引")) -> (element=w173:string)
          n26 = Decimal String To Number(string=w173, offset=4 ("偏移量")) -> (number=w176:i32)  [unwired: 1 in, 1 out]
          n27 = Fract/Exp String To Number(string=w173, offset=17 ("偏移量")) -> (number=w178:dbl)  [unwired: 2 in, 1 out]
          n28 = Fract/Exp String To Number(string=w173, offset=32 ("偏移量")) -> (number=w177:dbl)  [unwired: 2 in, 1 out]
        }
        n29 = mathscript code="result=sqrt(shibu.*shibu+xubu.*xubu)\nplot(x,result)\ntitle('表面幅仿真-Z方向')\nxlabel('频率/Hz')\nylabel('值/m')"("x"=w25, "xubu"=w24, "shibu"=w23) -> ()  [unwired: 1 in, 1 out]
      }
      event "表面幅仿真-Y方向": Value Change {
        n30 = event-data() -> ()  [unwired: 1 in, 6 out]
        n31 = call-poly <vilib>:"Read Delimited Spreadsheet.vi"("file path (dialog if empty)"=path "E:/6546/ymovement.prn") -> ("all rows"=w186:string[][])  [unwired: 9 in, 5 out]
        n32 = Delete From Array(array=w186, length=2 ("长度"), index (row)=0 ("索引 (行)")) -> (array with subset deleted=w185:string[][])  [unwired: 1 in, 1 out]
        n33 = for {
          tunnel: w185 -> [w334] mode=indexing
          tunnel: [w337] -> w183 mode=indexing
          tunnel: [w336] -> w182 mode=indexing
          tunnel: [w335] -> w184 mode=indexing
          n34 = Index Array(array=w334, index=0 ("索引")) -> (element=w332:string)
          n35 = Decimal String To Number(string=w332, offset=4 ("偏移量")) -> (number=w335:i32)  [unwired: 1 in, 1 out]
          n36 = Fract/Exp String To Number(string=w332, offset=17 ("偏移量")) -> (number=w337:dbl)  [unwired: 2 in, 1 out]
          n37 = Fract/Exp String To Number(string=w332, offset=32 ("偏移量")) -> (number=w336:dbl)  [unwired: 2 in, 1 out]
        }
        n38 = mathscript code="result=sqrt(shibu.*shibu+xubu.*xubu)\nplot(x,result)\ntitle('表面幅仿真-Y方向')\nxlabel('频率/Hz')\nylabel('值/m')"("x"=w184, "xubu"=w183, "shibu"=w182) -> ()  [unwired: 1 in, 1 out]
      }
      event "定子瞬态": Value Change {
        n39 = event-data() -> ()  [unwired: 1 in, 6 out]
        n40 = call-poly <vilib>:"Read Delimited Spreadsheet.vi"("file path (dialog if empty)"=path "E:/6546/finalshuntaimay.prn") -> ("all rows"=w344:string[][])  [unwired: 9 in, 5 out]
        n41 = Delete From Array(array=w344, length=2 ("长度"), index (row)=0 ("索引 (行)")) -> (array with subset deleted=w343:string[][])  [unwired: 1 in, 1 out]
        n42 = for {
          tunnel: w343 -> [w453] mode=indexing
          tunnel: [w454] -> w342 mode=indexing
          tunnel: [w449] -> w341 mode=indexing
          n43 = Index Array(array=w453, index=0 ("索引")) -> (element=w451:string)
          n44 = Fract/Exp String To Number(string=w451, offset=3 ("偏移量")) -> (number=w449:dbl)  [unwired: 2 in, 1 out]
          n45 = Fract/Exp String To Number(string=w451, offset=17 ("偏移量")) -> (number=w454:dbl)  [unwired: 2 in, 1 out]
        }
        n46 = mathscript code="plot(x,result)\ntitle('定子起振瞬态响应')\nxlabel('时间/s')\nylabel('值/m')"("x"=w341, "result"=w342) -> ()  [unwired: 1 in, 1 out]
      }
      event "表面幅仿真-X方向": Value Change {
        n47 = event-data() -> ()  [unwired: 1 in, 6 out]
        n48 = call-poly <vilib>:"Read Delimited Spreadsheet.vi"("file path (dialog if empty)"=path "E:/6546/xmovement.prn") -> ("all rows"=w460:string[][])  [unwired: 9 in, 5 out]
        n49 = Delete From Array(array=w460, length=2 ("长度"), index (row)=0 ("索引 (行)")) -> (array with subset deleted=w459:string[][])  [unwired: 1 in, 1 out]
        n50 = for {
          tunnel: w459 -> [w608] mode=indexing
          tunnel: [w611] -> w457 mode=indexing
          tunnel: [w610] -> w456 mode=indexing
          tunnel: [w609] -> w458 mode=indexing
          n51 = Index Array(array=w608, index=0 ("索引")) -> (element=w606:string)
          n52 = Decimal String To Number(string=w606, offset=4 ("偏移量")) -> (number=w609:i32)  [unwired: 1 in, 1 out]
          n53 = Fract/Exp String To Number(string=w606, offset=17 ("偏移量")) -> (number=w611:dbl)  [unwired: 2 in, 1 out]
          n54 = Fract/Exp String To Number(string=w606, offset=32 ("偏移量")) -> (number=w610:dbl)  [unwired: 2 in, 1 out]
        }
        n55 = mathscript code="result=sqrt(shibu.*shibu+xubu.*xubu)\nplot(x,result)\ntitle('表面幅仿真-X方向')\nxlabel('频率/Hz')\nylabel('值/m')"("x"=w458, "xubu"=w457, "shibu"=w456) -> ()  [unwired: 1 in, 1 out]
      }
      event "阻抗特性曲线": Value Change {
        n56 = event-data() -> ()  [unwired: 1 in, 6 out]
        n57 = call-poly <vilib>:"Read Delimited Spreadsheet.vi"("file path (dialog if empty)"=path "E:/6546/current.prn") -> ("all rows"=w619:string[][])  [unwired: 9 in, 5 out]
        n58 = Delete From Array(array=w619, length=2 ("长度"), index (row)=0 ("索引 (行)")) -> (array with subset deleted=w618:string[][])  [unwired: 1 in, 1 out]
        n59 = for {
          tunnel: w618 -> [w781] mode=indexing
          tunnel: [w784] -> w616 mode=indexing
          tunnel: [w783] -> w615 mode=indexing
          tunnel: [w782] -> w617 mode=indexing
          n60 = Index Array(array=w781, index=0 ("索引")) -> (element=w779:string)
          n61 = Decimal String To Number(string=w779, offset=4 ("偏移量")) -> (number=w782:i32)  [unwired: 1 in, 1 out]
          n62 = Fract/Exp String To Number(string=w779, offset=17 ("偏移量")) -> (number=w784:dbl)  [unwired: 2 in, 1 out]
          n63 = Fract/Exp String To Number(string=w779, offset=32 ("偏移量")) -> (number=w783:dbl)  [unwired: 2 in, 1 out]
        }
        n64 = mathscript code="result=sqrt(shibu.*shibu+xubu.*xubu)\nresult=1./result\nplot(x,result)\ntitle('阻抗特性')\nxlabel('频率/Hz')\nylabel('阻抗')"("x"=w617, "xubu"=w616, "shibu"=w615) -> ()  [unwired: 1 in, 1 out]
      }
      event "后一张": Value Change {
        n65 = event-data() -> ()  [unwired: 1 in, 6 out]
        n66 = flat-sequence {
          frame #0 {
            n67 = local read "数值"() -> (w789:dbl)
            n68 = case shown="14" w789 {
              selector: w789 -> [w791 w794]
              tunnel: [w790 w792] -> w788
              frame 0..13, Default {
                n69 = Increment(x=w791) -> (x+1=w790:i32)
              }
              frame 14 {
                n70 = Subtract(x=w794, y=14) -> (x-y=w792:i32)
              }
            }
            n71 = local write "数值"(w788) -> ()
          }
          frame #1 {
            n72 = local read "数值"() -> (w800:dbl)
            n73 = case shown="0..9" w800 {
              selector: w800 -> [w804 w808]
              tunnel: [w805 w807] -> w802
              frame 0..9 {
                n74 = Number To Decimal String(number=w804) -> (decimal integer string=w803:string)  [unwired: 1 in]
                n75 = Concatenate Strings("0" ("字符串"), w803) -> (w805:string)
              }
              frame 10..14, Default {
                n76 = Number To Decimal String(number=w808) -> (decimal integer string=w807:string)  [unwired: 1 in]
              }
            }
            n77 = Concatenate Strings("E:\\6546\\finaltest0", w802, ".jpg" ("字符串")) -> (w797:string)
            n78 = String To Path(string=w797) -> (path=w796:path)
            n79 = call <vilib>:"Read JPEG File.vi"("path to JPEG file"=w796) -> ("image data"=w798:T3)  [unwired: 8 in, 2 out]
            n80 = call <vilib>:"Draw Flattened Pixmap.vi"("image data"=w798) -> ("new picture"=→"new picture":picture)  [unwired: 8 in]
          }
        }
      }
      event "存": Value Change {
        n81 = event-data() -> ()  [unwired: 1 in, 6 out]
        n82 = local read "数值"() -> (w811:dbl)
        n83 = case shown="0..9" w811 {
          selector: w811 -> [w817 w821]
          tunnel: [w818 w820] -> w815
          frame 0..9 {
            n84 = Number To Decimal String(number=w817) -> (decimal integer string=w816:string)  [unwired: 1 in]
            n85 = Concatenate Strings("0" ("字符串"), w816) -> (w818:string)
          }
          frame 10..14, Default {
            n86 = Number To Decimal String(number=w821) -> (decimal integer string=w820:string)  [unwired: 1 in]
          }
        }
        n87 = Concatenate Strings("E:\\6546\\finaltest0", w815, ".jpg" ("字符串")) -> (w813:string)
        n88 = String To Path(string=w813) -> (path=w810:path)
        n89 = Copy(10:path "E:/ansys_result" ("目标路径（使用对话框）"), 11:w810) -> ()  [unwired: 3 in, 3 out]
      }
      event "一键删除": Value Change {
        n90 = event-data() -> ()  [unwired: 1 in, 6 out]
        n91 = flat-sequence {
          frame #0 {
            n92 = Delete(path (use dialog)=path "E:/6546" ("路径（使用对话框）"), entire hierarchy (F)=TRUE ("整个层次结构(F)"), confirm (F)=TRUE ("确认(F)")) -> ()  [unwired: 2 in, 3 out]
          }
          frame #1 {
            n93 = Create Folder(prompt (Create Folder)="E:\\6546" ("对话框窗口（创建文件夹）"), path (use dialog)=path "E:/6546" ("路径（使用对话框）")) -> ()  [unwired: 1 in, 3 out]
          }
          frame #2 {
            n94 = Copy(10:path "E:/6546" ("目标路径（使用对话框）"), 11:path "E:/finaltest.dat" ("源路径")) -> ()  [unwired: 3 in, 3 out]
          }
        }
      }
      event "1": Value Change {
        n95 = event-data() -> ()  [unwired: 1 in, 6 out]
        n96 = Number To Fractional String(number="齿数") -> (F-format string=w830:string)  [unwired: 3 in]
        n97 = Open/Create/Replace File(file path (use dialog)=path "H:/新/finaltest.dat" ("文件路径（使用对话框）"), operation (0:open)=T1."replace" ("操作(0:open)")) -> (refnum out=w836:refnum<file>)  [unwired: 4 in, 2 out]
        n98 = Concatenate Strings("/RGB,INDEX,100,100,100, 0   \n/RGB,INDEX, 80, 80, 80,13   \n/RGB,INDEX, 60, 60, 60,14   \n/RGB,INDEX, 0, 0, 0,15  \n\n/REPLOT,RESIZE  \n/CLEAR,NOSTART \nNZ=" ("字符串"), w830, " !齿数：\nTH=1.5 !平均齿高：\nWTH=1.5 !外侧斜齿高\nNTH=1.5 !内侧斜齿高\nWDTH=0.0 !齿外侧导角高度\nWDTL=0.0 !齿外侧导水平长度\nNDTH=0.0 !齿内侧导角高度\nNDTL=0.0 !齿内侧导水平长度\nTT=2 !齿厚：\nTW=0.1 !齿槽宽：\nITD=8 !定子齿内圈直径：\nOTD=13.3 !定子齿外圈直径：\nIAD=2.1 !轴内圈直径：\nOAD=6 !轴外圈直径：\nAT=1.6 !轴厚度\nPT=0.4 !压电片厚：\nIPD=8 !压电片内圈直径：\nOPD=13.3 !压电片外圈直径：\nEW= ITD-OAD !宽度：\nET=0.2 !厚度：\nEH=0.2 !台阶高：\nBS=4 !波数\nFK=5 !定子分块建模分块数与齿数成整数倍的关系 \n\nNZ=NZ !齿数：\nTH=TH/1000 !齿高：\nWTH=WTH/1000 !外侧斜齿高\nNTH=NTH/1000 !内侧斜齿高\nWDTH=WDTH/1000 !齿外侧导角高度\nWDTL=WDTL/1000 !齿外侧导水平长度\nNDTH=NDTH/1000 !齿内侧导角高度\nNDTL=NDTL/1000 !齿内侧导水平长度\nTT=TT/1000 !齿厚：\nTW=TW/1000 !齿槽宽：\nITD=ITD/1000 !定子齿内圈直径：\nOTD=OTD/1000 !定子齿外圈直径：\nIAD=IAD/1000 !轴内圈直径：\nOAD=OAD/1000 !轴外圈直径：\nAT=AT/1000 !轴厚度\nPT=PT/1000 !压电片厚：\nIPD=IPD/1000 !压电片内圈直径：\nOPD=OPD/1000 !压电片外圈直径：\nEW= EW/1000 !宽度：\nET=ET/1000 !厚度：\nEH=EH/1000 !台阶高：\n\n/PREP7 \n!定义单元和材料属性\nET,1,SOLID185   \nMPTEMP,,,,,,,,  \nMPTEMP,1,0  \nMPDATA,DENS,1,,8290\nMPTEMP,,,,,,,,  \nMPTEMP,1,0  \nMPDATA,EX,1,,1.06E+011   \nMPDATA,PRXY,1,,0.35 \n\nET,2,SOLID5 \nMPTEMP,,,,,,,,  \nMPTEMP,1,0     \nMPDATA,DENS,2,,7750   \nMPTEMP,,,,,,,,  \nMPTEMP,1,0  \nMPDATA,PERX,2,,919E-009\nMPDATA,PERY,2,,919E-009   \nMPDATA,PERZ,2,,826E-009\nTB,PIEZ,2,,,0   \nTBMODIF,1,1,0   \nTBMODIF,1,2,0   \nTBMODIF,1,3,-5.35   \nTBMODIF,2,1,0   \nTBMODIF,2,2,0   \nTBMODIF,2,3,-5.35   \nTBMODIF,3,1,0   \nTBMODIF,3,2,0   \nTBMODIF,3,3,15.78   \nTBMODIF,4,1,0   \nTBMODIF,4,2,0   \nTBMODIF,4,3,0   \nTBMODIF,5,1,0   \nTBMODIF,5,2,12.3\nTBMODIF,5,3,0   \nTBMODIF,6,1,12.3\nTBMODIF,6,2,0   \nTBMODIF,6,3,0   \nTB,ANEL,2,1,21,0\nTBTEMP,0\nTBDATA,,1.2035E+011,7.52E+010,7.51E+010,0,0,0   \nTBDATA,,1.204E+011,7.51E+010,0,0,0,1.109E+011   \nTBDATA,,0,0,0,2.26E+010,0,0 \nTBDATA,,2.12E+010,0,2.11E+010,,,\n\n!超声波电机模型建立\nK,1,OAD/2,,,\nK,2,ITD/2,,,\nK,3,ITD/2,-EH,,!最上面\nK,4,OTD/2,-EH,,\nK,5,OTD/2,-EH+TT-TH,,\nK,6,ITD/2,-EH+TT-TH,,\nK,7,ITD/2,ET,,\nK,8,OAD/2,ET,,\nK,11,ITD/2,-EH-PT,,!最下面\nK,12,OTD/2,-EH-PT,,\nK,13,OTD/2,-EH+TT,,\nK,14,ITD/2,-EH+TT,,\nK,15,IAD/2,ET,,\nK,16,IAD/2,0,,\nK,17,IAD/2,-AT+ET,,\nK,18,OAD/2,-AT+ET,,\n\nK,100,0,0,0,\nK,101,0,0.003,0,\n\nLSTR,1,2\nLSTR,2,3\nLSTR,3,4\nLSTR,4,5\nLSTR,5,6\nLSTR,6,7\nLSTR,7,8\nLSTR,8,1\nLSTR,3,11\nLSTR,11,12\nLSTR,12,4\nLSTR,5,13\nLSTR,13,14\nLSTR,14,6\nLSTR,2,7\nLSTR,8,15\nLSTR,15,16\nLSTR,1,16\nLSTR,16,17\nLSTR,17,18\nLSTR,1,18\n\nAL,1,15,7,8\nAL,15,2,3,4,5,6,\nAL,9,10,11,3\nAL,5,12,13,14\nAL,8,16,17,18\nAL,18,19,20,21\n\nVROTAT,1,2,3,4, , ,100,101 ,360/FK, , !!!!!\nVROTAT,5,6, , , , ,100,101 ,360/FK, , !!!!!\nBLC4,0,TT-EH,OTD,-TH,TW !建立长方体\nVGEN, ,7, , , , ,-TW/2, , ,1!复制创建体  \nVOVLAP,4,7 !布尔操作\nVDELE,10, , ,1!删除体\nVSYMM,Z,8, , , ,0,0 !体镜像 \n\n!建立齿槽\nCSYS,5  \nWPSTYLE,,,,,,,,0\nVGEN,NZ/FK+1,4, , , ,360/NZ, , ,0  \nVGEN,NZ/FK+1,8, , , ,360/NZ, , ,0  \nVOVLAP,ALL\n*DO,I,1,NZ/FK+1\nCSYS,0\nVSEL,S,LOC,Y,TT-EH-TH/1.5,1\nCSYS,5\nVSEL,R,LOC,Y,(I-1)*360/NZ-TW/2/3.1415/ITD*360,TW/2/3.1415/ITD*360+(I-1)*360/NZ!选择体\nVDELE,ALL, , ,1\nALLSEL,ALL \n*ENDDO\n\n!旋转成体\nEPLOT \nCSYS,5 \nVGEN,FK,ALL, , , ,360/FK, , ,0 \n\n!Glue体\nVGLUE,ALL\n\n!添加材料属性\nALLSEL,ALL\nCSYS,0\nVSEL,S,LOC,Y,0,TT-EH\nVATT,       1, ,   1,       0   \nCSYS,5\nVSEL,S,LOC,X,0,OAD/2\nVATT,       1, ,   1,       0 \n\nALLSEL,ALL\nCSYS,0\nVSEL,R,LOC,Y,-EH-PT,-EH\nVATT,       2, ,  2,       0  \nALLSEL,ALL\n\n!网格体\nCSYS,0\nVSEL,R,LOC,Y,-EH-PT,-EH\nVSWEEP,ALL\n\nCSYS,0\nALLSEL,ALL \nVSEL,S,MAT,,1\nSMRT,6  \nSMRT,5  \nSMRT,4  \nMSHAPE,1,3d\nMSHKEY,0\nVMESH,ALL\n\nALLSEL,ALL\n\n!模态分析 \n/SOL  \nANTYPE,2\nMODOPT,LANB,22  \nEQSLV,SPAR  \nMXPAND,0, , ,0  \nLUMPM,0 \nPSTRES,0\nMODOPT,LANB,22,0,80000, ,OFF\n\nCSYS,5\nASEL,S,LOC,X,-IAD/2,IAD/2   \nDA,ALL,ALL,\nALLSEL,ALL\n\n!OUTPR,BASIC,ALL,  \n!OUTRES,ALL,ALL,\n \n/STATUS,SOLU\nSOLVE   \nFINISH\nCSYS,0\nALLSEL,ALL\n\n/POST1  \nSET,FIRST   \n/EFACET,1   \nPLNSOL, U,SUM, 2,1.0 !无轮廓2变0\n/post1\n*do,i,8,22\nset,1,i\n/VIEW,1,1,2,3   \n/ANG,1  \n/REP,FAST  \n/show,jpeg,,\nplnsol,u,sum,0,1.0\n/show,close\n*enddo\nFINISH\n\n!振幅仿真\n/SOL\nANTYPE,3\nHROPT,FULL  \nHROUT,ON\nLUMPM,0 \nEQSLV, ,0,  \nPSTRES,0\n\n!阻尼特性\nALPHAD,0,   \nBETAD,0,\nDMPSTR,0.005,   \n\n!压电耦合\n*do,i,1,(BS-1)\nALLSEL,ALL\ncsys,5\nnsel,S,LOC,X,ITD/2,OTD/2\ncsys,0\nnsel,R,loc,y,-eh-eq-pt\ncsys,5\nangle=360/BS\nnsel,r,loc,y,(i-1)*angle/2,i*angle/2\nb=1/2*(1-(-1)**i)*1\nc=1/2*(1-(-1)**(i+1))*1\nD,All,VOLT,b,c\n*enddo\n\nALLSEL,ALL\ncsys,5\nnsel,S,LOC,X,ITD/2,OTD/2\ncsys,0\nnsel,R,loc,y,-eh-eq-pt\ncsys,5\nangle=360/BS\nnsel,r,loc,y,(BS-1)*angle/2,((BS-1)*angle/2+3*angle/8)\nD,All,VOLT,(1/2*(1-(-1)**BS)*1),(1/2*(1-(-1)**(BS+1))*1)\n\nALLSEL,ALL\ncsys,5\nnsel,S,LOC,X,ITD/2,OTD/2\ncsys,0\nnsel,R,loc,y,-eh-eq-pt\ncsys,5\nangle=360/BS\nnsel,r,loc,y,((BS-1)*angle/2+3*angle/8),((BS-1)*angle/2+3*angle/4)\nD,All,VOLT,(1/2*(1-(-1)**(BS+1))*1),(1/2*(1-(-1)**(BS+2))*1)\n\n*do,i,1,(BS-1)\nALLSEL,ALL\ncsys,5\nnsel,S,LOC,X,ITD/2,OTD/2\ncsys,0\nnsel,R,loc,y,-eh-eq-pt\ncsys,5\nangle=360/BS\nnsel,r,loc,y,((BS-1)*angle/2+3*angle/4+(i-1)*angle/2),((BS-1)*angle/2+3*angle/4+(i)*angle/2)\ne=1/2*(1-(-1)**(BS+1+i))*1\nf=1/2*(1-(-1)**(BS+2+i))*1\nD,All,VOLT,e,f\n*enddo\n\nALLSEL,ALL\ncsys,5\nnsel,S,LOC,X,ITD/2,OTD/2\ncsys,0\nnsel,r,loc,y,-eh-eq\nD,All,VOLT,0,0\nALLSEL,ALL \n\nHARFRQ,26000,76000, \nNSUBST,5,  \nKBC,1\n/STATUS,SOLU\nSOLVE\n\n!选最大位移点\n/POST1\nNSORT,U,SUM,0,1, ,SELECT  \nPRNSOL,U,Z\n*get,node,SORT,0,IMAX\n\n!结果显示,打开后处理器\n/POST26 \nFILE,'finaltest','rst','.'   \n/UI,COLL,1  \nNUMVAR,200  \nSOLU,191,NCMIT  \nSTORE,MERGE \nPLCPLX,0\nPRCPLX,1\nFILLDATA,191,,,,1,1 \nREALVAR,191,191 \n\n!z方向位移 \nNSOL,2,node,U,Z, UZ_2, \nSTORE,MERGE \n\n!保存为txt(excel也行)\n/post26\n! Save time history variables to file zmovement.prn\n*CREATE,scratch,gui \n*DEL,_P26_EXPORT\n*DIM,_P26_EXPORT,TABLE,5,2 \nVGET,_P26_EXPORT(1,0),1 \nVGET,_P26_EXPORT(1,1),2,,0  \nVGET,_P26_EXPORT(1,2),2,,1  \n/OUTPUT,'zmovement','prn','.'  \n*VWRITE,'FREQ','UZ_2',' '   \n%14C %14C %14C\n*VWRITE,' ','REAL','IMAGINARY'  \n%14C %14C %14C  \n*VWRITE,_P26_EXPORT(1,0),_P26_EXPORT(1,1),_P26_EXPORT(1,2)  \n%14.5G %14.5G %14.5G\n/OUTPUT,TERM\n*END\n/INPUT,scratch,gui  \n! End of time history save  \n\n!x方向位移 \nNSOL,3,node,U,X, UX_3, \nSTORE,MERGE \n\n!保存为txt(excel也行)\n/post26\n! Save time history variables to file xmovement.prn\n*CREATE,scratch,gui \n*DEL,_P26_EXPORT\n*DIM,_P26_EXPORT,TABLE,5,2 \nVGET,_P26_EXPORT(1,0),1 \nVGET,_P26_EXPORT(1,1),3,,0  \nVGET,_P26_EXPORT(1,2),3,,1  \n/OUTPUT,'xmovement','prn','.'  \n*VWRITE,'FREQ','UX_3',' '   \n%14C %14C %14C  \n*VWRITE,' ','REAL','IMAGINARY'  \n%14C %14C %14C  \n*VWRITE,_P26_EXPORT(1,0),_P26_EXPORT(1,1),_P26_EXPORT(1,2)  \n%14.5G %14.5G %14.5G\n/OUTPUT,TERM\n*END\n/INPUT,scratch,gui  \n! End of time history save\n\n!y方向位移 \nNSOL,4,node,U,Y, UY_4, \nSTORE,MERGE \n\n!保存为txt(excel也行)\n/post26\n! Save time history variables to file ymovement.prn\n*CREATE,scratch,gui \n*DEL,_P26_EXPORT\n*DIM,_P26_EXPORT,TABLE,5,2 \nVGET,_P26_EXPORT(1,0),1 \nVGET,_P26_EXPORT(1,1),4,,0  \nVGET,_P26_EXPORT(1,2),4,,1  \n/OUTPUT,'ymovement','prn','.'  \n*VWRITE,'FREQ','UY_4',' '   \n%14C %14C %14C  \n*VWRITE,' ','REAL','IMAGINARY'  \n%14C %14C %14C  \n*VWRITE,_P26_EXPORT(1,0),_P26_EXPORT(1,1),_P26_EXPORT(1,2)  \n%14.5G %14.5G %14.5G\n/OUTPUT,TERM\n*END\n/INPUT,scratch,gui  \n! End of time history save\n\n!选择电流点\nRFORCE,2,180,AMPS,, AMPS_2  \nSTORE,MERGE \nFILLDATA,192,,,,0,0 \nFILLDATA,193,,,,1,0 \nFILLDATA,194,,,,-1,0\nFILLDATA,195,,,,1,1 \nVARNAME,195,NSET\n! Name: Z   \n! ID:  3\n! Function: 1/{AMPS_2}  \nFILLDATA,199,,,,1,0 \nREALVAR,199,199 \nQUOT,3,199,2,,Z \nSTORE,MERGE \n\n!保存为txt(excel也行)\n/post26\n! Save time history variables to file current.prn   \n*CREATE,scratch,gui \n*DEL,_P26_EXPORT\n*DIM,_P26_EXPORT,TABLE,5,2 \nVGET,_P26_EXPORT(1,0),1 \nVGET,_P26_EXPORT(1,1),3,,0  \nVGET,_P26_EXPORT(1,2),3,,1  \n/OUTPUT,'current','prn','.' \n*VWRITE,'FREQ','Z',' '  \n%14C %14C %14C  \n*VWRITE,' ','REAL','IMAGINARY'  \n%14C %14C %14C  \n*VWRITE,_P26_EXPORT(1,0),_P26_EXPORT(1,1),_P26_EXPORT(1,2)  \n%14.5G %14.5G %14.5G\n/OUTPUT,TERM\n*END\n/INPUT,scratch,gui  \n! End of time history save " ("字符串")) -> (w835:string)
        n99 = Write to Text File(file (use dialog)=w836, text=w835) -> ()  [unwired: 2 in, 3 out]
      }
      event "2": Value Change {
        n100 = event-data() -> ()  [unwired: 1 in, 6 out]
        n101 = Number To Fractional String(number="平均齿高") -> (F-format string=w839:string)  [unwired: 3 in]
        n102 = Open/Create/Replace File(file path (use dialog)=path "H:/新/finaltest.dat" ("文件路径（使用对话框）"), operation (0:open)=T1."replace" ("操作(0:open)")) -> (refnum out=w844:refnum<file>)  [unwired: 4 in, 2 out]
        n103 = Concatenate Strings("/RGB,INDEX,100,100,100, 0   \n/RGB,INDEX, 80, 80, 80,13   \n/RGB,INDEX, 60, 60, 60,14   \n/RGB,INDEX, 0, 0, 0,15  \n\n/REPLOT,RESIZE  \n/CLEAR,NOSTART \nNZ=24.000000 !齿数：\nTH=" ("字符串"), w839, "  !平均齿高：\nWTH=1.5 !外侧斜齿高\nNTH=1.5 !内侧斜齿高\nWDTH=0.0 !齿外侧导角高度\nWDTL=0.0 !齿外侧导水平长度\nNDTH=0.0 !齿内侧导角高度\nNDTL=0.0 !齿内侧导水平长度\nTT=2 !齿厚：\nTW=0.1 !齿槽宽：\nITD=8 !定子齿内圈直径：\nOTD=13.3 !定子齿外圈直径：\nIAD=2.1 !轴内圈直径：\nOAD=6 !轴外圈直径：\nAT=1.6 !轴厚度\nPT=0.4 !压电片厚：\nIPD=8 !压电片内圈直径：\nOPD=13.3 !压电片外圈直径：\nEW= ITD-OAD !宽度：\nET=0.2 !厚度：\nEH=0.2 !台阶高：\nBS=4 !波数\nFK=5 !定子分块建模分块数与齿数成整数倍的关系 \n\nNZ=NZ !齿数：\nTH=TH/1000 !齿高：\nWTH=WTH/1000 !外侧斜齿高\nNTH=NTH/1000 !内侧斜齿高\nWDTH=WDTH/1000 !齿外侧导角高度\nWDTL=WDTL/1000 !齿外侧导水平长度\nNDTH=NDTH/1000 !齿内侧导角高度\nNDTL=NDTL/1000 !齿内侧导水平长度\nTT=TT/1000 !齿厚：\nTW=TW/1000 !齿槽宽：\nITD=ITD/1000 !定子齿内圈直径：\nOTD=OTD/1000 !定子齿外圈直径：\nIAD=IAD/1000 !轴内圈直径：\nOAD=OAD/1000 !轴外圈直径：\nAT=AT/1000 !轴厚度\nPT=PT/1000 !压电片厚：\nIPD=IPD/1000 !压电片内圈直径：\nOPD=OPD/1000 !压电片外圈直径：\nEW= EW/1000 !宽度：\nET=ET/1000 !厚度：\nEH=EH/1000 !台阶高：\n\n/PREP7 \n!定义单元和材料属性\nET,1,SOLID185   \nMPTEMP,,,,,,,,  \nMPTEMP,1,0  \nMPDATA,DENS,1,,8290\nMPTEMP,,,,,,,,  \nMPTEMP,1,0  \nMPDATA,EX,1,,1.06E+011   \nMPDATA,PRXY,1,,0.35 \n\nET,2,SOLID5 \nMPTEMP,,,,,,,,  \nMPTEMP,1,0     \nMPDATA,DENS,2,,7750   \nMPTEMP,,,,,,,,  \nMPTEMP,1,0  \nMPDATA,PERX,2,,919E-009\nMPDATA,PERY,2,,919E-009   \nMPDATA,PERZ,2,,826E-009\nTB,PIEZ,2,,,0   \nTBMODIF,1,1,0   \nTBMODIF,1,2,0   \nTBMODIF,1,3,-5.35   \nTBMODIF,2,1,0   \nTBMODIF,2,2,0   \nTBMODIF,2,3,-5.35   \nTBMODIF,3,1,0   \nTBMODIF,3,2,0   \nTBMODIF,3,3,15.78   \nTBMODIF,4,1,0   \nTBMODIF,4,2,0   \nTBMODIF,4,3,0   \nTBMODIF,5,1,0   \nTBMODIF,5,2,12.3\nTBMODIF,5,3,0   \nTBMODIF,6,1,12.3\nTBMODIF,6,2,0   \nTBMODIF,6,3,0   \nTB,ANEL,2,1,21,0\nTBTEMP,0\nTBDATA,,1.2035E+011,7.52E+010,7.51E+010,0,0,0   \nTBDATA,,1.204E+011,7.51E+010,0,0,0,1.109E+011   \nTBDATA,,0,0,0,2.26E+010,0,0 \nTBDATA,,2.12E+010,0,2.11E+010,,,\n\n!超声波电机模型建立\nK,1,OAD/2,,,\nK,2,ITD/2,,,\nK,3,ITD/2,-EH,,!最上面\nK,4,OTD/2,-EH,,\nK,5,OTD/2,-EH+TT-TH,,\nK,6,ITD/2,-EH+TT-TH,,\nK,7,ITD/2,ET,,\nK,8,OAD/2,ET,,\nK,11,ITD/2,-EH-PT,,!最下面\nK,12,OTD/2,-EH-PT,,\nK,13,OTD/2,-EH+TT,,\nK,14,ITD/2,-EH+TT,,\nK,15,IAD/2,ET,,\nK,16,IAD/2,0,,\nK,17,IAD/2,-AT+ET,,\nK,18,OAD/2,-AT+ET,,\n\nK,100,0,0,0,\nK,101,0,0.003,0,\n\nLSTR,1,2\nLSTR,2,3\nLSTR,3,4\nLSTR,4,5\nLSTR,5,6\nLSTR,6,7\nLSTR,7,8\nLSTR,8,1\nLSTR,3,11\nLSTR,11,12\nLSTR,12,4\nLSTR,5,13\nLSTR,13,14\nLSTR,14,6\nLSTR,2,7\nLSTR,8,15\nLSTR,15,16\nLSTR,1,16\nLSTR,16,17\nLSTR,17,18\nLSTR,1,18\n\nAL,1,15,7,8\nAL,15,2,3,4,5,6,\nAL,9,10,11,3\nAL,5,12,13,14\nAL,8,16,17,18\nAL,18,19,20,21\n\nVROTAT,1,2,3,4, , ,100,101 ,360/FK, , !!!!!\nVROTAT,5,6, , , , ,100,101 ,360/FK, , !!!!!\nBLC4,0,TT-EH,OTD,-TH,TW !建立长方体\nVGEN, ,7, , , , ,-TW/2, , ,1!复制创建体  \nVOVLAP,4,7 !布尔操作\nVDELE,10, , ,1!删除体\nVSYMM,Z,8, , , ,0,0 !体镜像 \n\n!建立齿槽\nCSYS,5  \nWPSTYLE,,,,,,,,0\nVGEN,NZ/FK+1,4, , , ,360/NZ, , ,0  \nVGEN,NZ/FK+1,8, , , ,360/NZ, , ,0  \nVOVLAP,ALL\n*DO,I,1,NZ/FK+1\nCSYS,0\nVSEL,S,LOC,Y,TT-EH-TH/1.5,1\nCSYS,5\nVSEL,R,LOC,Y,(I-1)*360/NZ-TW/2/3.1415/ITD*360,TW/2/3.1415/ITD*360+(I-1)*360/NZ!选择体\nVDELE,ALL, , ,1\nALLSEL,ALL \n*ENDDO\n\n!旋转成体\nEPLOT \nCSYS,5 \nVGEN,FK,ALL, , , ,360/FK, , ,0 \n\n!Glue体\nVGLUE,ALL\n\n!添加材料属性\nALLSEL,ALL\nCSYS,0\nVSEL,S,LOC,Y,0,TT-EH\nVATT,       1, ,   1,       0   \nCSYS,5\nVSEL,S,LOC,X,0,OAD/2\nVATT,       1, ,   1,       0 \n\nALLSEL,ALL\nCSYS,0\nVSEL,R,LOC,Y,-EH-PT,-EH\nVATT,       2, ,  2,       0  \nALLSEL,ALL\n\n!网格体\nCSYS,0\nVSEL,R,LOC,Y,-EH-PT,-EH\nVSWEEP,ALL\n\nCSYS,0\nALLSEL,ALL \nVSEL,S,MAT,,1\nSMRT,6  \nSMRT,5  \nSMRT,4  \nMSHAPE,1,3d\nMSHKEY,0\nVMESH,ALL\n\nALLSEL,ALL\n\n!模态分析 \n/SOL  \nANTYPE,2\nMODOPT,LANB,22  \nEQSLV,SPAR  \nMXPAND,0, , ,0  \nLUMPM,0 \nPSTRES,0\nMODOPT,LANB,22,0,80000, ,OFF\n\nCSYS,5\nASEL,S,LOC,X,-IAD/2,IAD/2   \nDA,ALL,ALL,\nALLSEL,ALL\n\n!OUTPR,BASIC,ALL,  \n!OUTRES,ALL,ALL,\n \n/STATUS,SOLU\nSOLVE   \nFINISH\nCSYS,0\nALLSEL,ALL\n\n/POST1  \nSET,FIRST   \n/EFACET,1   \nPLNSOL, U,SUM, 2,1.0 !无轮廓2变0\n/post1\n*do,i,8,22\nset,1,i\n/VIEW,1,1,2,3   \n/ANG,1  \n/REP,FAST  \n/show,jpeg,,\nplnsol,u,sum,0,1.0\n/show,close\n*enddo\nFINISH\n\n!振幅仿真\n/SOL\nANTYPE,3\nHROPT,FULL  \nHROUT,ON\nLUMPM,0 \nEQSLV, ,0,  \nPSTRES,0\n\n!阻尼特性\nALPHAD,0,   \nBETAD,0,\nDMPSTR,0.005,   \n\n!压电耦合\n*do,i,1,(BS-1)\nALLSEL,ALL\ncsys,5\nnsel,S,LOC,X,ITD/2,OTD/2\ncsys,0\nnsel,R,loc,y,-eh-eq-pt\ncsys,5\nangle=360/BS\nnsel,r,loc,y,(i-1)*angle/2,i*angle/2\nb=1/2*(1-(-1)**i)*1\nc=1/2*(1-(-1)**(i+1))*1\nD,All,VOLT,b,c\n*enddo\n\nALLSEL,ALL\ncsys,5\nnsel,S,LOC,X,ITD/2,OTD/2\ncsys,0\nnsel,R,loc,y,-eh-eq-pt\ncsys,5\nangle=360/BS\nnsel,r,loc,y,(BS-1)*angle/2,((BS-1)*angle/2+3*angle/8)\nD,All,VOLT,(1/2*(1-(-1)**BS)*1),(1/2*(1-(-1)**(BS+1))*1)\n\nALLSEL,ALL\ncsys,5\nnsel,S,LOC,X,ITD/2,OTD/2\ncsys,0\nnsel,R,loc,y,-eh-eq-pt\ncsys,5\nangle=360/BS\nnsel,r,loc,y,((BS-1)*angle/2+3*angle/8),((BS-1)*angle/2+3*angle/4)\nD,All,VOLT,(1/2*(1-(-1)**(BS+1))*1),(1/2*(1-(-1)**(BS+2))*1)\n\n*do,i,1,(BS-1)\nALLSEL,ALL\ncsys,5\nnsel,S,LOC,X,ITD/2,OTD/2\ncsys,0\nnsel,R,loc,y,-eh-eq-pt\ncsys,5\nangle=360/BS\nnsel,r,loc,y,((BS-1)*angle/2+3*angle/4+(i-1)*angle/2),((BS-1)*angle/2+3*angle/4+(i)*angle/2)\ne=1/2*(1-(-1)**(BS+1+i))*1\nf=1/2*(1-(-1)**(BS+2+i))*1\nD,All,VOLT,e,f\n*enddo\n\nALLSEL,ALL\ncsys,5\nnsel,S,LOC,X,ITD/2,OTD/2\ncsys,0\nnsel,r,loc,y,-eh-eq\nD,All,VOLT,0,0\nALLSEL,ALL \n\nHARFRQ,26000,76000, \nNSUBST,5,  \nKBC,1\n/STATUS,SOLU\nSOLVE\n\n!选最大位移点\n/POST1\nNSORT,U,SUM,0,1, ,SELECT  \nPRNSOL,U,Z\n*get,node,SORT,0,IMAX\n\n!结果显示,打开后处理器\n/POST26 \nFILE,'finaltest','rst','.'   \n/UI,COLL,1  \nNUMVAR,200  \nSOLU,191,NCMIT  \nSTORE,MERGE \nPLCPLX,0\nPRCPLX,1\nFILLDATA,191,,,,1,1 \nREALVAR,191,191 \n\n!z方向位移 \nNSOL,2,node,U,Z, UZ_2, \nSTORE,MERGE \n\n!保存为txt(excel也行)\n/post26\n! Save time history variables to file zmovement.prn\n*CREATE,scratch,gui \n*DEL,_P26_EXPORT\n*DIM,_P26_EXPORT,TABLE,5,2 \nVGET,_P26_EXPORT(1,0),1 \nVGET,_P26_EXPORT(1,1),2,,0  \nVGET,_P26_EXPORT(1,2),2,,1  \n/OUTPUT,'zmovement','prn','.'  \n*VWRITE,'FREQ','UZ_2',' '   \n%14C %14C %14C\n*VWRITE,' ','REAL','IMAGINARY'  \n%14C %14C %14C  \n*VWRITE,_P26_EXPORT(1,0),_P26_EXPORT(1,1),_P26_EXPORT(1,2)  \n%14.5G %14.5G %14.5G\n/OUTPUT,TERM\n*END\n/INPUT,scratch,gui  \n! End of time history save  \n\n!x方向位移 \nNSOL,3,node,U,X, UX_3, \nSTORE,MERGE \n\n!保存为txt(excel也行)\n/post26\n! Save time history variables to file xmovement.prn\n*CREATE,scratch,gui \n*DEL,_P26_EXPORT\n*DIM,_P26_EXPORT,TABLE,5,2 \nVGET,_P26_EXPORT(1,0),1 \nVGET,_P26_EXPORT(1,1),3,,0  \nVGET,_P26_EXPORT(1,2),3,,1  \n/OUTPUT,'xmovement','prn','.'  \n*VWRITE,'FREQ','UX_3',' '   \n%14C %14C %14C  \n*VWRITE,' ','REAL','IMAGINARY'  \n%14C %14C %14C  \n*VWRITE,_P26_EXPORT(1,0),_P26_EXPORT(1,1),_P26_EXPORT(1,2)  \n%14.5G %14.5G %14.5G\n/OUTPUT,TERM\n*END\n/INPUT,scratch,gui  \n! End of time history save\n\n!y方向位移 \nNSOL,4,node,U,Y, UY_4, \nSTORE,MERGE \n\n!保存为txt(excel也行)\n/post26\n! Save time history variables to file ymovement.prn\n*CREATE,scratch,gui \n*DEL,_P26_EXPORT\n*DIM,_P26_EXPORT,TABLE,5,2 \nVGET,_P26_EXPORT(1,0),1 \nVGET,_P26_EXPORT(1,1),4,,0  \nVGET,_P26_EXPORT(1,2),4,,1  \n/OUTPUT,'ymovement','prn','.'  \n*VWRITE,'FREQ','UY_4',' '   \n%14C %14C %14C  \n*VWRITE,' ','REAL','IMAGINARY'  \n%14C %14C %14C  \n*VWRITE,_P26_EXPORT(1,0),_P26_EXPORT(1,1),_P26_EXPORT(1,2)  \n%14.5G %14.5G %14.5G\n/OUTPUT,TERM\n*END\n/INPUT,scratch,gui  \n! End of time history save\n\n!选择电流点\nRFORCE,2,180,AMPS,, AMPS_2  \nSTORE,MERGE \nFILLDATA,192,,,,0,0 \nFILLDATA,193,,,,1,0 \nFILLDATA,194,,,,-1,0\nFILLDATA,195,,,,1,1 \nVARNAME,195,NSET\n! Name: Z   \n! ID:  3\n! Function: 1/{AMPS_2}  \nFILLDATA,199,,,,1,0 \nREALVAR,199,199 \nQUOT,3,199,2,,Z \nSTORE,MERGE \n\n!保存为txt(excel也行)\n/post26\n! Save time history variables to file current.prn   \n*CREATE,scratch,gui \n*DEL,_P26_EXPORT\n*DIM,_P26_EXPORT,TABLE,5,2 \nVGET,_P26_EXPORT(1,0),1 \nVGET,_P26_EXPORT(1,1),3,,0  \nVGET,_P26_EXPORT(1,2),3,,1  \n/OUTPUT,'current','prn','.' \n*VWRITE,'FREQ','Z',' '  \n%14C %14C %14C  \n*VWRITE,' ','REAL','IMAGINARY'  \n%14C %14C %14C  \n*VWRITE,_P26_EXPORT(1,0),_P26_EXPORT(1,1),_P26_EXPORT(1,2)  \n%14.5G %14.5G %14.5G\n/OUTPUT,TERM\n*END\n/INPUT,scratch,gui  \n! End of time history save " ("字符串")) -> (w843:string)
        n104 = Write to Text File(file (use dialog)=w844, text=w843) -> ()  [unwired: 2 in, 3 out]
      }
      event "3": Value Change {
        n105 = event-data() -> ()  [unwired: 1 in, 6 out]
        n106 = Number To Fractional String(number="外侧斜齿高") -> (F-format string=w847:string)  [unwired: 3 in]
        n107 = Open/Create/Replace File(file path (use dialog)=path "H:/新/finaltest.dat" ("文件路径（使用对话框）"), operation (0:open)=T1."replace" ("操作(0:open)")) -> (refnum out=w852:refnum<file>)  [unwired: 4 in, 2 out]
        n108 = Concatenate Strings("/RGB,INDEX,100,100,100, 0   \n/RGB,INDEX, 80, 80, 80,13   \n/RGB,INDEX, 60, 60, 60,14   \n/RGB,INDEX, 0, 0, 0,15  \n\n/REPLOT,RESIZE  \n/CLEAR,NOSTART \nNZ=25 !齿数：\nTH=1.5 !平均齿高：\nWTH=" ("字符串"), w847, "  !外侧斜齿高\nNTH=1.5 !内侧斜齿高\nWDTH=0.0 !齿外侧导角高度\nWDTL=0.0 !齿外侧导水平长度\nNDTH=0.0 !齿内侧导角高度\nNDTL=0.0 !齿内侧导水平长度\nTT=2 !齿厚：\nTW=0.1 !齿槽宽：\nITD=8 !定子齿内圈直径：\nOTD=13.3 !定子齿外圈直径：\nIAD=2.1 !轴内圈直径：\nOAD=6 !轴外圈直径：\nAT=1.6 !轴厚度\nPT=0.4 !压电片厚：\nIPD=8 !压电片内圈直径：\nOPD=13.3 !压电片外圈直径：\nEW= ITD-OAD !宽度：\nET=0.2 !厚度：\nEH=0.2 !台阶高：\nBS=4 !波数\nFK=5 !定子分块建模分块数与齿数成整数倍的关系 \n\nNZ=NZ !齿数：\nTH=TH/1000 !齿高：\nWTH=WTH/1000 !外侧斜齿高\nNTH=NTH/1000 !内侧斜齿高\nWDTH=WDTH/1000 !齿外侧导角高度\nWDTL=WDTL/1000 !齿外侧导水平长度\nNDTH=NDTH/1000 !齿内侧导角高度\nNDTL=NDTL/1000 !齿内侧导水平长度\nTT=TT/1000 !齿厚：\nTW=TW/1000 !齿槽宽：\nITD=ITD/1000 !定子齿内圈直径：\nOTD=OTD/1000 !定子齿外圈直径：\nIAD=IAD/1000 !轴内圈直径：\nOAD=OAD/1000 !轴外圈直径：\nAT=AT/1000 !轴厚度\nPT=PT/1000 !压电片厚：\nIPD=IPD/1000 !压电片内圈直径：\nOPD=OPD/1000 !压电片外圈直径：\nEW= EW/1000 !宽度：\nET=ET/1000 !厚度：\nEH=EH/1000 !台阶高：\n\n/PREP7 \n!定义单元和材料属性\nET,1,SOLID185   \nMPTEMP,,,,,,,,  \nMPTEMP,1,0  \nMPDATA,DENS,1,,8290\nMPTEMP,,,,,,,,  \nMPTEMP,1,0  \nMPDATA,EX,1,,1.06E+011   \nMPDATA,PRXY,1,,0.35 \n\nET,2,SOLID5 \nMPTEMP,,,,,,,,  \nMPTEMP,1,0     \nMPDATA,DENS,2,,7750   \nMPTEMP,,,,,,,,  \nMPTEMP,1,0  \nMPDATA,PERX,2,,919E-009\nMPDATA,PERY,2,,919E-009   \nMPDATA,PERZ,2,,826E-009\nTB,PIEZ,2,,,0   \nTBMODIF,1,1,0   \nTBMODIF,1,2,0   \nTBMODIF,1,3,-5.35   \nTBMODIF,2,1,0   \nTBMODIF,2,2,0   \nTBMODIF,2,3,-5.35   \nTBMODIF,3,1,0   \nTBMODIF,3,2,0   \nTBMODIF,3,3,15.78   \nTBMODIF,4,1,0   \nTBMODIF,4,2,0   \nTBMODIF,4,3,0   \nTBMODIF,5,1,0   \nTBMODIF,5,2,12.3\nTBMODIF,5,3,0   \nTBMODIF,6,1,12.3\nTBMODIF,6,2,0   \nTBMODIF,6,3,0   \nTB,ANEL,2,1,21,0\nTBTEMP,0\nTBDATA,,1.2035E+011,7.52E+010,7.51E+010,0,0,0   \nTBDATA,,1.204E+011,7.51E+010,0,0,0,1.109E+011   \nTBDATA,,0,0,0,2.26E+010,0,0 \nTBDATA,,2.12E+010,0,2.11E+010,,,\n\n!超声波电机模型建立\nK,1,OAD/2,,,\nK,2,ITD/2,,,\nK,3,ITD/2,-EH,,!最上面\nK,4,OTD/2,-EH,,\nK,5,OTD/2,-EH+TT-TH,,\nK,6,ITD/2,-EH+TT-TH,,\nK,7,ITD/2,ET,,\nK,8,OAD/2,ET,,\nK,11,ITD/2,-EH-PT,,!最下面\nK,12,OTD/2,-EH-PT,,\nK,13,OTD/2,-EH+TT,,\nK,14,ITD/2,-EH+TT,,\nK,15,IAD/2,ET,,\nK,16,IAD/2,0,,\nK,17,IAD/2,-AT+ET,,\nK,18,OAD/2,-AT+ET,,\n\nK,100,0,0,0,\nK,101,0,0.003,0,\n\nLSTR,1,2\nLSTR,2,3\nLSTR,3,4\nLSTR,4,5\nLSTR,5,6\nLSTR,6,7\nLSTR,7,8\nLSTR,8,1\nLSTR,3,11\nLSTR,11,12\nLSTR,12,4\nLSTR,5,13\nLSTR,13,14\nLSTR,14,6\nLSTR,2,7\nLSTR,8,15\nLSTR,15,16\nLSTR,1,16\nLSTR,16,17\nLSTR,17,18\nLSTR,1,18\n\nAL,1,15,7,8\nAL,15,2,3,4,5,6,\nAL,9,10,11,3\nAL,5,12,13,14\nAL,8,16,17,18\nAL,18,19,20,21\n\nVROTAT,1,2,3,4, , ,100,101 ,360/FK, , !!!!!\nVROTAT,5,6, , , , ,100,101 ,360/FK, , !!!!!\nBLC4,0,TT-EH,OTD,-TH,TW !建立长方体\nVGEN, ,7, , , , ,-TW/2, , ,1!复制创建体  \nVOVLAP,4,7 !布尔操作\nVDELE,10, , ,1!删除体\nVSYMM,Z,8, , , ,0,0 !体镜像 \n\n!建立齿槽\nCSYS,5  \nWPSTYLE,,,,,,,,0\nVGEN,NZ/FK+1,4, , , ,360/NZ, , ,0  \nVGEN,NZ/FK+1,8, , , ,360/NZ, , ,0  \nVOVLAP,ALL\n*DO,I,1,NZ/FK+1\nCSYS,0\nVSEL,S,LOC,Y,TT-EH-TH/1.5,1\nCSYS,5\nVSEL,R,LOC,Y,(I-1)*360/NZ-TW/2/3.1415/ITD*360,TW/2/3.1415/ITD*360+(I-1)*360/NZ!选择体\nVDELE,ALL, , ,1\nALLSEL,ALL \n*ENDDO\n\n!旋转成体\nEPLOT \nCSYS,5 \nVGEN,FK,ALL, , , ,360/FK, , ,0 \n\n!Glue体\nVGLUE,ALL\n\n!添加材料属性\nALLSEL,ALL\nCSYS,0\nVSEL,S,LOC,Y,0,TT-EH\nVATT,       1, ,   1,       0   \nCSYS,5\nVSEL,S,LOC,X,0,OAD/2\nVATT,       1, ,   1,       0 \n\nALLSEL,ALL\nCSYS,0\nVSEL,R,LOC,Y,-EH-PT,-EH\nVATT,       2, ,  2,       0  \nALLSEL,ALL\n\n!网格体\nCSYS,0\nVSEL,R,LOC,Y,-EH-PT,-EH\nVSWEEP,ALL\n\nCSYS,0\nALLSEL,ALL \nVSEL,S,MAT,,1\nSMRT,6  \nSMRT,5  \nSMRT,4  \nMSHAPE,1,3d\nMSHKEY,0\nVMESH,ALL\n\nALLSEL,ALL\n\n!模态分析 \n/SOL  \nANTYPE,2\nMODOPT,LANB,22  \nEQSLV,SPAR  \nMXPAND,0, , ,0  \nLUMPM,0 \nPSTRES,0\nMODOPT,LANB,22,0,80000, ,OFF\n\nCSYS,5\nASEL,S,LOC,X,-IAD/2,IAD/2   \nDA,ALL,ALL,\nALLSEL,ALL\n\n!OUTPR,BASIC,ALL,  \n!OUTRES,ALL,ALL,\n \n/STATUS,SOLU\nSOLVE   \nFINISH\nCSYS,0\nALLSEL,ALL\n\n/POST1  \nSET,FIRST   \n/EFACET,1   \nPLNSOL, U,SUM, 2,1.0 !无轮廓2变0\n/post1\n*do,i,8,22\nset,1,i\n/VIEW,1,1,2,3   \n/ANG,1  \n/REP,FAST  \n/show,jpeg,,\nplnsol,u,sum,0,1.0\n/show,close\n*enddo\nFINISH\n\n!振幅仿真\n/SOL\nANTYPE,3\nHROPT,FULL  \nHROUT,ON\nLUMPM,0 \nEQSLV, ,0,  \nPSTRES,0\n\n!阻尼特性\nALPHAD,0,   \nBETAD,0,\nDMPSTR,0.005,   \n\n!压电耦合\n*do,i,1,(BS-1)\nALLSEL,ALL\ncsys,5\nnsel,S,LOC,X,ITD/2,OTD/2\ncsys,0\nnsel,R,loc,y,-eh-eq-pt\ncsys,5\nangle=360/BS\nnsel,r,loc,y,(i-1)*angle/2,i*angle/2\nb=1/2*(1-(-1)**i)*1\nc=1/2*(1-(-1)**(i+1))*1\nD,All,VOLT,b,c\n*enddo\n\nALLSEL,ALL\ncsys,5\nnsel,S,LOC,X,ITD/2,OTD/2\ncsys,0\nnsel,R,loc,y,-eh-eq-pt\ncsys,5\nangle=360/BS\nnsel,r,loc,y,(BS-1)*angle/2,((BS-1)*angle/2+3*angle/8)\nD,All,VOLT,(1/2*(1-(-1)**BS)*1),(1/2*(1-(-1)**(BS+1))*1)\n\nALLSEL,ALL\ncsys,5\nnsel,S,LOC,X,ITD/2,OTD/2\ncsys,0\nnsel,R,loc,y,-eh-eq-pt\ncsys,5\nangle=360/BS\nnsel,r,loc,y,((BS-1)*angle/2+3*angle/8),((BS-1)*angle/2+3*angle/4)\nD,All,VOLT,(1/2*(1-(-1)**(BS+1))*1),(1/2*(1-(-1)**(BS+2))*1)\n\n*do,i,1,(BS-1)\nALLSEL,ALL\ncsys,5\nnsel,S,LOC,X,ITD/2,OTD/2\ncsys,0\nnsel,R,loc,y,-eh-eq-pt\ncsys,5\nangle=360/BS\nnsel,r,loc,y,((BS-1)*angle/2+3*angle/4+(i-1)*angle/2),((BS-1)*angle/2+3*angle/4+(i)*angle/2)\ne=1/2*(1-(-1)**(BS+1+i))*1\nf=1/2*(1-(-1)**(BS+2+i))*1\nD,All,VOLT,e,f\n*enddo\n\nALLSEL,ALL\ncsys,5\nnsel,S,LOC,X,ITD/2,OTD/2\ncsys,0\nnsel,r,loc,y,-eh-eq\nD,All,VOLT,0,0\nALLSEL,ALL \n\nHARFRQ,26000,76000, \nNSUBST,5,  \nKBC,1\n/STATUS,SOLU\nSOLVE\n\n!选最大位移点\n/POST1\nNSORT,U,SUM,0,1, ,SELECT  \nPRNSOL,U,Z\n*get,node,SORT,0,IMAX\n\n!结果显示,打开后处理器\n/POST26 \nFILE,'finaltest','rst','.'   \n/UI,COLL,1  \nNUMVAR,200  \nSOLU,191,NCMIT  \nSTORE,MERGE \nPLCPLX,0\nPRCPLX,1\nFILLDATA,191,,,,1,1 \nREALVAR,191,191 \n\n!z方向位移 \nNSOL,2,node,U,Z, UZ_2, \nSTORE,MERGE \n\n!保存为txt(excel也行)\n/post26\n! Save time history variables to file zmovement.prn\n*CREATE,scratch,gui \n*DEL,_P26_EXPORT\n*DIM,_P26_EXPORT,TABLE,5,2 \nVGET,_P26_EXPORT(1,0),1 \nVGET,_P26_EXPORT(1,1),2,,0  \nVGET,_P26_EXPORT(1,2),2,,1  \n/OUTPUT,'zmovement','prn','.'  \n*VWRITE,'FREQ','UZ_2',' '   \n%14C %14C %14C\n*VWRITE,' ','REAL','IMAGINARY'  \n%14C %14C %14C  \n*VWRITE,_P26_EXPORT(1,0),_P26_EXPORT(1,1),_P26_EXPORT(1,2)  \n%14.5G %14.5G %14.5G\n/OUTPUT,TERM\n*END\n/INPUT,scratch,gui  \n! End of time history save  \n\n!x方向位移 \nNSOL,3,node,U,X, UX_3, \nSTORE,MERGE \n\n!保存为txt(excel也行)\n/post26\n! Save time history variables to file xmovement.prn\n*CREATE,scratch,gui \n*DEL,_P26_EXPORT\n*DIM,_P26_EXPORT,TABLE,5,2 \nVGET,_P26_EXPORT(1,0),1 \nVGET,_P26_EXPORT(1,1),3,,0  \nVGET,_P26_EXPORT(1,2),3,,1  \n/OUTPUT,'xmovement','prn','.'  \n*VWRITE,'FREQ','UX_3',' '   \n%14C %14C %14C  \n*VWRITE,' ','REAL','IMAGINARY'  \n%14C %14C %14C  \n*VWRITE,_P26_EXPORT(1,0),_P26_EXPORT(1,1),_P26_EXPORT(1,2)  \n%14.5G %14.5G %14.5G\n/OUTPUT,TERM\n*END\n/INPUT,scratch,gui  \n! End of time history save\n\n!y方向位移 \nNSOL,4,node,U,Y, UY_4, \nSTORE,MERGE \n\n!保存为txt(excel也行)\n/post26\n! Save time history variables to file ymovement.prn\n*CREATE,scratch,gui \n*DEL,_P26_EXPORT\n*DIM,_P26_EXPORT,TABLE,5,2 \nVGET,_P26_EXPORT(1,0),1 \nVGET,_P26_EXPORT(1,1),4,,0  \nVGET,_P26_EXPORT(1,2),4,,1  \n/OUTPUT,'ymovement','prn','.'  \n*VWRITE,'FREQ','UY_4',' '   \n%14C %14C %14C  \n*VWRITE,' ','REAL','IMAGINARY'  \n%14C %14C %14C  \n*VWRITE,_P26_EXPORT(1,0),_P26_EXPORT(1,1),_P26_EXPORT(1,2)  \n%14.5G %14.5G %14.5G\n/OUTPUT,TERM\n*END\n/INPUT,scratch,gui  \n! End of time history save\n\n!选择电流点\nRFORCE,2,180,AMPS,, AMPS_2  \nSTORE,MERGE \nFILLDATA,192,,,,0,0 \nFILLDATA,193,,,,1,0 \nFILLDATA,194,,,,-1,0\nFILLDATA,195,,,,1,1 \nVARNAME,195,NSET\n! Name: Z   \n! ID:  3\n! Function: 1/{AMPS_2}  \nFILLDATA,199,,,,1,0 \nREALVAR,199,199 \nQUOT,3,199,2,,Z \nSTORE,MERGE \n\n!保存为txt(excel也行)\n/post26\n! Save time history variables to file current.prn   \n*CREATE,scratch,gui \n*DEL,_P26_EXPORT\n*DIM,_P26_EXPORT,TABLE,5,2 \nVGET,_P26_EXPORT(1,0),1 \nVGET,_P26_EXPORT(1,1),3,,0  \nVGET,_P26_EXPORT(1,2),3,,1  \n/OUTPUT,'current','prn','.' \n*VWRITE,'FREQ','Z',' '  \n%14C %14C %14C  \n*VWRITE,' ','REAL','IMAGINARY'  \n%14C %14C %14C  \n*VWRITE,_P26_EXPORT(1,0),_P26_EXPORT(1,1),_P26_EXPORT(1,2)  \n%14.5G %14.5G %14.5G\n/OUTPUT,TERM\n*END\n/INPUT,scratch,gui  \n! End of time history save " ("字符串")) -> (w851:string)
        n109 = Write to Text File(file (use dialog)=w852, text=w851) -> ()  [unwired: 2 in, 3 out]
      }
      event "4": Value Change {
        n110 = event-data() -> ()  [unwired: 1 in, 6 out]
        n111 = Number To Fractional String(number="内侧斜齿高") -> (F-format string=w855:string)  [unwired: 3 in]
        n112 = Open/Create/Replace File(file path (use dialog)=path "H:/新/finaltest.dat" ("文件路径（使用对话框）"), operation (0:open)=T1."replace" ("操作(0:open)")) -> (refnum out=w860:refnum<file>)  [unwired: 4 in, 2 out]
        n113 = Concatenate Strings("/RGB,INDEX,100,100,100, 0   \n/RGB,INDEX, 80, 80, 80,13   \n/RGB,INDEX, 60, 60, 60,14   \n/RGB,INDEX, 0, 0, 0,15  \n\n/REPLOT,RESIZE  \n/CLEAR,NOSTART \nNZ=25 !齿数：\nTH=1.5 !平均齿高：\nWTH=1.5 !外侧斜齿高\nNTH=" ("字符串"), w855, " !内侧斜齿高\nWDTH=0.0 !齿外侧导角高度\nWDTL=0.0 !齿外侧导水平长度\nNDTH=0.0 !齿内侧导角高度\nNDTL=0.0 !齿内侧导水平长度\nTT=2 !齿厚：\nTW=0.1 !齿槽宽：\nITD=8 !定子齿内圈直径：\nOTD=13.3 !定子齿外圈直径：\nIAD=2.1 !轴内圈直径：\nOAD=6 !轴外圈直径：\nAT=1.6 !轴厚度\nPT=0.4 !压电片厚：\nIPD=8 !压电片内圈直径：\nOPD=13.3 !压电片外圈直径：\nEW= ITD-OAD !宽度：\nET=0.2 !厚度：\nEH=0.2 !台阶高：\nBS=4 !波数\nFK=5 !定子分块建模分块数与齿数成整数倍的关系 \n\nNZ=NZ !齿数：\nTH=TH/1000 !齿高：\nWTH=WTH/1000 !外侧斜齿高\nNTH=NTH/1000 !内侧斜齿高\nWDTH=WDTH/1000 !齿外侧导角高度\nWDTL=WDTL/1000 !齿外侧导水平长度\nNDTH=NDTH/1000 !齿内侧导角高度\nNDTL=NDTL/1000 !齿内侧导水平长度\nTT=TT/1000 !齿厚：\nTW=TW/1000 !齿槽宽：\nITD=ITD/1000 !定子齿内圈直径：\nOTD=OTD/1000 !定子齿外圈直径：\nIAD=IAD/1000 !轴内圈直径：\nOAD=OAD/1000 !轴外圈直径：\nAT=AT/1000 !轴厚度\nPT=PT/1000 !压电片厚：\nIPD=IPD/1000 !压电片内圈直径：\nOPD=OPD/1000 !压电片外圈直径：\nEW= EW/1000 !宽度：\nET=ET/1000 !厚度：\nEH=EH/1000 !台阶高：\n\n/PREP7 \n!定义单元和材料属性\nET,1,SOLID185   \nMPTEMP,,,,,,,,  \nMPTEMP,1,0  \nMPDATA,DENS,1,,8290\nMPTEMP,,,,,,,,  \nMPTEMP,1,0  \nMPDATA,EX,1,,1.06E+011   \nMPDATA,PRXY,1,,0.35 \n\nET,2,SOLID5 \nMPTEMP,,,,,,,,  \nMPTEMP,1,0     \nMPDATA,DENS,2,,7750   \nMPTEMP,,,,,,,,  \nMPTEMP,1,0  \nMPDATA,PERX,2,,919E-009\nMPDATA,PERY,2,,919E-009   \nMPDATA,PERZ,2,,826E-009\nTB,PIEZ,2,,,0   \nTBMODIF,1,1,0   \nTBMODIF,1,2,0   \nTBMODIF,1,3,-5.35   \nTBMODIF,2,1,0   \nTBMODIF,2,2,0   \nTBMODIF,2,3,-5.35   \nTBMODIF,3,1,0   \nTBMODIF,3,2,0   \nTBMODIF,3,3,15.78   \nTBMODIF,4,1,0   \nTBMODIF,4,2,0   \nTBMODIF,4,3,0   \nTBMODIF,5,1,0   \nTBMODIF,5,2,12.3\nTBMODIF,5,3,0   \nTBMODIF,6,1,12.3\nTBMODIF,6,2,0   \nTBMODIF,6,3,0   \nTB,ANEL,2,1,21,0\nTBTEMP,0\nTBDATA,,1.2035E+011,7.52E+010,7.51E+010,0,0,0   \nTBDATA,,1.204E+011,7.51E+010,0,0,0,1.109E+011   \nTBDATA,,0,0,0,2.26E+010,0,0 \nTBDATA,,2.12E+010,0,2.11E+010,,,\n\n!超声波电机模型建立\nK,1,OAD/2,,,\nK,2,ITD/2,,,\nK,3,ITD/2,-EH,,!最上面\nK,4,OTD/2,-EH,,\nK,5,OTD/2,-EH+TT-TH,,\nK,6,ITD/2,-EH+TT-TH,,\nK,7,ITD/2,ET,,\nK,8,OAD/2,ET,,\nK,11,ITD/2,-EH-PT,,!最下面\nK,12,OTD/2,-EH-PT,,\nK,13,OTD/2,-EH+TT,,\nK,14,ITD/2,-EH+TT,,\nK,15,IAD/2,ET,,\nK,16,IAD/2,0,,\nK,17,IAD/2,-AT+ET,,\nK,18,OAD/2,-AT+ET,,\n\nK,100,0,0,0,\nK,101,0,0.003,0,\n\nLSTR,1,2\nLSTR,2,3\nLSTR,3,4\nLSTR,4,5\nLSTR,5,6\nLSTR,6,7\nLSTR,7,8\nLSTR,8,1\nLSTR,3,11\nLSTR,11,12\nLSTR,12,4\nLSTR,5,13\nLSTR,13,14\nLSTR,14,6\nLSTR,2,7\nLSTR,8,15\nLSTR,15,16\nLSTR,1,16\nLSTR,16,17\nLSTR,17,18\nLSTR,1,18\n\nAL,1,15,7,8\nAL,15,2,3,4,5,6,\nAL,9,10,11,3\nAL,5,12,13,14\nAL,8,16,17,18\nAL,18,19,20,21\n\nVROTAT,1,2,3,4, , ,100,101 ,360/FK, , !!!!!\nVROTAT,5,6, , , , ,100,101 ,360/FK, , !!!!!\nBLC4,0,TT-EH,OTD,-TH,TW !建立长方体\nVGEN, ,7, , , , ,-TW/2, , ,1!复制创建体  \nVOVLAP,4,7 !布尔操作\nVDELE,10, , ,1!删除体\nVSYMM,Z,8, , , ,0,0 !体镜像 \n\n!建立齿槽\nCSYS,5  \nWPSTYLE,,,,,,,,0\nVGEN,NZ/FK+1,4, , , ,360/NZ, , ,0  \nVGEN,NZ/FK+1,8, , , ,360/NZ, , ,0  \nVOVLAP,ALL\n*DO,I,1,NZ/FK+1\nCSYS,0\nVSEL,S,LOC,Y,TT-EH-TH/1.5,1\nCSYS,5\nVSEL,R,LOC,Y,(I-1)*360/NZ-TW/2/3.1415/ITD*360,TW/2/3.1415/ITD*360+(I-1)*360/NZ!选择体\nVDELE,ALL, , ,1\nALLSEL,ALL \n*ENDDO\n\n!旋转成体\nEPLOT \nCSYS,5 \nVGEN,FK,ALL, , , ,360/FK, , ,0 \n\n!Glue体\nVGLUE,ALL\n\n!添加材料属性\nALLSEL,ALL\nCSYS,0\nVSEL,S,LOC,Y,0,TT-EH\nVATT,       1, ,   1,       0   \nCSYS,5\nVSEL,S,LOC,X,0,OAD/2\nVATT,       1, ,   1,       0 \n\nALLSEL,ALL\nCSYS,0\nVSEL,R,LOC,Y,-EH-PT,-EH\nVATT,       2, ,  2,       0  \nALLSEL,ALL\n\n!网格体\nCSYS,0\nVSEL,R,LOC,Y,-EH-PT,-EH\nVSWEEP,ALL\n\nCSYS,0\nALLSEL,ALL \nVSEL,S,MAT,,1\nSMRT,6  \nSMRT,5  \nSMRT,4  \nMSHAPE,1,3d\nMSHKEY,0\nVMESH,ALL\n\nALLSEL,ALL\n\n!模态分析 \n/SOL  \nANTYPE,2\nMODOPT,LANB,22  \nEQSLV,SPAR  \nMXPAND,0, , ,0  \nLUMPM,0 \nPSTRES,0\nMODOPT,LANB,22,0,80000, ,OFF\n\nCSYS,5\nASEL,S,LOC,X,-IAD/2,IAD/2   \nDA,ALL,ALL,\nALLSEL,ALL\n\n!OUTPR,BASIC,ALL,  \n!OUTRES,ALL,ALL,\n \n/STATUS,SOLU\nSOLVE   \nFINISH\nCSYS,0\nALLSEL,ALL\n\n/POST1  \nSET,FIRST   \n/EFACET,1   \nPLNSOL, U,SUM, 2,1.0 !无轮廓2变0\n/post1\n*do,i,8,22\nset,1,i\n/VIEW,1,1,2,3   \n/ANG,1  \n/REP,FAST  \n/show,jpeg,,\nplnsol,u,sum,0,1.0\n/show,close\n*enddo\nFINISH\n\n!振幅仿真\n/SOL\nANTYPE,3\nHROPT,FULL  \nHROUT,ON\nLUMPM,0 \nEQSLV, ,0,  \nPSTRES,0\n\n!阻尼特性\nALPHAD,0,   \nBETAD,0,\nDMPSTR,0.005,   \n\n!压电耦合\n*do,i,1,(BS-1)\nALLSEL,ALL\ncsys,5\nnsel,S,LOC,X,ITD/2,OTD/2\ncsys,0\nnsel,R,loc,y,-eh-eq-pt\ncsys,5\nangle=360/BS\nnsel,r,loc,y,(i-1)*angle/2,i*angle/2\nb=1/2*(1-(-1)**i)*1\nc=1/2*(1-(-1)**(i+1))*1\nD,All,VOLT,b,c\n*enddo\n\nALLSEL,ALL\ncsys,5\nnsel,S,LOC,X,ITD/2,OTD/2\ncsys,0\nnsel,R,loc,y,-eh-eq-pt\ncsys,5\nangle=360/BS\nnsel,r,loc,y,(BS-1)*angle/2,((BS-1)*angle/2+3*angle/8)\nD,All,VOLT,(1/2*(1-(-1)**BS)*1),(1/2*(1-(-1)**(BS+1))*1)\n\nALLSEL,ALL\ncsys,5\nnsel,S,LOC,X,ITD/2,OTD/2\ncsys,0\nnsel,R,loc,y,-eh-eq-pt\ncsys,5\nangle=360/BS\nnsel,r,loc,y,((BS-1)*angle/2+3*angle/8),((BS-1)*angle/2+3*angle/4)\nD,All,VOLT,(1/2*(1-(-1)**(BS+1))*1),(1/2*(1-(-1)**(BS+2))*1)\n\n*do,i,1,(BS-1)\nALLSEL,ALL\ncsys,5\nnsel,S,LOC,X,ITD/2,OTD/2\ncsys,0\nnsel,R,loc,y,-eh-eq-pt\ncsys,5\nangle=360/BS\nnsel,r,loc,y,((BS-1)*angle/2+3*angle/4+(i-1)*angle/2),((BS-1)*angle/2+3*angle/4+(i)*angle/2)\ne=1/2*(1-(-1)**(BS+1+i))*1\nf=1/2*(1-(-1)**(BS+2+i))*1\nD,All,VOLT,e,f\n*enddo\n\nALLSEL,ALL\ncsys,5\nnsel,S,LOC,X,ITD/2,OTD/2\ncsys,0\nnsel,r,loc,y,-eh-eq\nD,All,VOLT,0,0\nALLSEL,ALL \n\nHARFRQ,26000,76000, \nNSUBST,5,  \nKBC,1\n/STATUS,SOLU\nSOLVE\n\n!选最大位移点\n/POST1\nNSORT,U,SUM,0,1, ,SELECT  \nPRNSOL,U,Z\n*get,node,SORT,0,IMAX\n\n!结果显示,打开后处理器\n/POST26 \nFILE,'finaltest','rst','.'   \n/UI,COLL,1  \nNUMVAR,200  \nSOLU,191,NCMIT  \nSTORE,MERGE \nPLCPLX,0\nPRCPLX,1\nFILLDATA,191,,,,1,1 \nREALVAR,191,191 \n\n!z方向位移 \nNSOL,2,node,U,Z, UZ_2, \nSTORE,MERGE \n\n!保存为txt(excel也行)\n/post26\n! Save time history variables to file zmovement.prn\n*CREATE,scratch,gui \n*DEL,_P26_EXPORT\n*DIM,_P26_EXPORT,TABLE,5,2 \nVGET,_P26_EXPORT(1,0),1 \nVGET,_P26_EXPORT(1,1),2,,0  \nVGET,_P26_EXPORT(1,2),2,,1  \n/OUTPUT,'zmovement','prn','.'  \n*VWRITE,'FREQ','UZ_2',' '   \n%14C %14C %14C\n*VWRITE,' ','REAL','IMAGINARY'  \n%14C %14C %14C  \n*VWRITE,_P26_EXPORT(1,0),_P26_EXPORT(1,1),_P26_EXPORT(1,2)  \n%14.5G %14.5G %14.5G\n/OUTPUT,TERM\n*END\n/INPUT,scratch,gui  \n! End of time history save  \n\n!x方向位移 \nNSOL,3,node,U,X, UX_3, \nSTORE,MERGE \n\n!保存为txt(excel也行)\n/post26\n! Save time history variables to file xmovement.prn\n*CREATE,scratch,gui \n*DEL,_P26_EXPORT\n*DIM,_P26_EXPORT,TABLE,5,2 \nVGET,_P26_EXPORT(1,0),1 \nVGET,_P26_EXPORT(1,1),3,,0  \nVGET,_P26_EXPORT(1,2),3,,1  \n/OUTPUT,'xmovement','prn','.'  \n*VWRITE,'FREQ','UX_3',' '   \n%14C %14C %14C  \n*VWRITE,' ','REAL','IMAGINARY'  \n%14C %14C %14C  \n*VWRITE,_P26_EXPORT(1,0),_P26_EXPORT(1,1),_P26_EXPORT(1,2)  \n%14.5G %14.5G %14.5G\n/OUTPUT,TERM\n*END\n/INPUT,scratch,gui  \n! End of time history save\n\n!y方向位移 \nNSOL,4,node,U,Y, UY_4, \nSTORE,MERGE \n\n!保存为txt(excel也行)\n/post26\n! Save time history variables to file ymovement.prn\n*CREATE,scratch,gui \n*DEL,_P26_EXPORT\n*DIM,_P26_EXPORT,TABLE,5,2 \nVGET,_P26_EXPORT(1,0),1 \nVGET,_P26_EXPORT(1,1),4,,0  \nVGET,_P26_EXPORT(1,2),4,,1  \n/OUTPUT,'ymovement','prn','.'  \n*VWRITE,'FREQ','UY_4',' '   \n%14C %14C %14C  \n*VWRITE,' ','REAL','IMAGINARY'  \n%14C %14C %14C  \n*VWRITE,_P26_EXPORT(1,0),_P26_EXPORT(1,1),_P26_EXPORT(1,2)  \n%14.5G %14.5G %14.5G\n/OUTPUT,TERM\n*END\n/INPUT,scratch,gui  \n! End of time history save\n\n!选择电流点\nRFORCE,2,180,AMPS,, AMPS_2  \nSTORE,MERGE \nFILLDATA,192,,,,0,0 \nFILLDATA,193,,,,1,0 \nFILLDATA,194,,,,-1,0\nFILLDATA,195,,,,1,1 \nVARNAME,195,NSET\n! Name: Z   \n! ID:  3\n! Function: 1/{AMPS_2}  \nFILLDATA,199,,,,1,0 \nREALVAR,199,199 \nQUOT,3,199,2,,Z \nSTORE,MERGE \n\n!保存为txt(excel也行)\n/post26\n! Save time history variables to file current.prn   \n*CREATE,scratch,gui \n*DEL,_P26_EXPORT\n*DIM,_P26_EXPORT,TABLE,5,2 \nVGET,_P26_EXPORT(1,0),1 \nVGET,_P26_EXPORT(1,1),3,,0  \nVGET,_P26_EXPORT(1,2),3,,1  \n/OUTPUT,'current','prn','.' \n*VWRITE,'FREQ','Z',' '  \n%14C %14C %14C  \n*VWRITE,' ','REAL','IMAGINARY'  \n%14C %14C %14C  \n*VWRITE,_P26_EXPORT(1,0),_P26_EXPORT(1,1),_P26_EXPORT(1,2)  \n%14.5G %14.5G %14.5G\n/OUTPUT,TERM\n*END\n/INPUT,scratch,gui  \n! End of time history save " ("字符串")) -> (w859:string)
        n114 = Write to Text File(file (use dialog)=w860, text=w859) -> ()  [unwired: 2 in, 3 out]
      }
      event "5": Value Change {
        n115 = event-data() -> ()  [unwired: 1 in, 6 out]
        n116 = Number To Fractional String(number="齿厚") -> (F-format string=w863:string)  [unwired: 3 in]
        n117 = Open/Create/Replace File(file path (use dialog)=path "H:/新/finaltest.dat" ("文件路径（使用对话框）"), operation (0:open)=T1."replace" ("操作(0:open)")) -> (refnum out=w868:refnum<file>)  [unwired: 4 in, 2 out]
        n118 = Concatenate Strings("/RGB,INDEX,100,100,100, 0   \n/RGB,INDEX, 80, 80, 80,13   \n/RGB,INDEX, 60, 60, 60,14   \n/RGB,INDEX, 0, 0, 0,15  \n\n/REPLOT,RESIZE  \n/CLEAR,NOSTART \nNZ=25 !齿数：\nTH=1.5 !平均齿高：\nWTH=1.5 !外侧斜齿高\nNTH=1.5 !内侧斜齿高\nWDTH=0.0 !齿外侧导角高度\nWDTL=0.0 !齿外侧导水平长度\nNDTH=0.0 !齿内侧导角高度\nNDTL=0.0 !齿内侧导水平长度\nTT=" ("字符串"), w863, " !齿厚：\nTW=0.1 !齿槽宽：\nITD=8 !定子齿内圈直径：\nOTD=13.3 !定子齿外圈直径：\nIAD=2.1 !轴内圈直径：\nOAD=6 !轴外圈直径：\nAT=1.6 !轴厚度\nPT=0.4 !压电片厚：\nIPD=8 !压电片内圈直径：\nOPD=13.3 !压电片外圈直径：\nEW= ITD-OAD !宽度：\nET=0.2 !厚度：\nEH=0.2 !台阶高：\nBS=4 !波数\nFK=5 !定子分块建模分块数与齿数成整数倍的关系 \n\nNZ=NZ !齿数：\nTH=TH/1000 !齿高：\nWTH=WTH/1000 !外侧斜齿高\nNTH=NTH/1000 !内侧斜齿高\nWDTH=WDTH/1000 !齿外侧导角高度\nWDTL=WDTL/1000 !齿外侧导水平长度\nNDTH=NDTH/1000 !齿内侧导角高度\nNDTL=NDTL/1000 !齿内侧导水平长度\nTT=TT/1000 !齿厚：\nTW=TW/1000 !齿槽宽：\nITD=ITD/1000 !定子齿内圈直径：\nOTD=OTD/1000 !定子齿外圈直径：\nIAD=IAD/1000 !轴内圈直径：\nOAD=OAD/1000 !轴外圈直径：\nAT=AT/1000 !轴厚度\nPT=PT/1000 !压电片厚：\nIPD=IPD/1000 !压电片内圈直径：\nOPD=OPD/1000 !压电片外圈直径：\nEW= EW/1000 !宽度：\nET=ET/1000 !厚度：\nEH=EH/1000 !台阶高：\n\n/PREP7 \n!定义单元和材料属性\nET,1,SOLID185   \nMPTEMP,,,,,,,,  \nMPTEMP,1,0  \nMPDATA,DENS,1,,8290\nMPTEMP,,,,,,,,  \nMPTEMP,1,0  \nMPDATA,EX,1,,1.06E+011   \nMPDATA,PRXY,1,,0.35 \n\nET,2,SOLID5 \nMPTEMP,,,,,,,,  \nMPTEMP,1,0     \nMPDATA,DENS,2,,7750   \nMPTEMP,,,,,,,,  \nMPTEMP,1,0  \nMPDATA,PERX,2,,919E-009\nMPDATA,PERY,2,,919E-009   \nMPDATA,PERZ,2,,826E-009\nTB,PIEZ,2,,,0   \nTBMODIF,1,1,0   \nTBMODIF,1,2,0   \nTBMODIF,1,3,-5.35   \nTBMODIF,2,1,0   \nTBMODIF,2,2,0   \nTBMODIF,2,3,-5.35   \nTBMODIF,3,1,0   \nTBMODIF,3,2,0   \nTBMODIF,3,3,15.78   \nTBMODIF,4,1,0   \nTBMODIF,4,2,0   \nTBMODIF,4,3,0   \nTBMODIF,5,1,0   \nTBMODIF,5,2,12.3\nTBMODIF,5,3,0   \nTBMODIF,6,1,12.3\nTBMODIF,6,2,0   \nTBMODIF,6,3,0   \nTB,ANEL,2,1,21,0\nTBTEMP,0\nTBDATA,,1.2035E+011,7.52E+010,7.51E+010,0,0,0   \nTBDATA,,1.204E+011,7.51E+010,0,0,0,1.109E+011   \nTBDATA,,0,0,0,2.26E+010,0,0 \nTBDATA,,2.12E+010,0,2.11E+010,,,\n\n!超声波电机模型建立\nK,1,OAD/2,,,\nK,2,ITD/2,,,\nK,3,ITD/2,-EH,,!最上面\nK,4,OTD/2,-EH,,\nK,5,OTD/2,-EH+TT-TH,,\nK,6,ITD/2,-EH+TT-TH,,\nK,7,ITD/2,ET,,\nK,8,OAD/2,ET,,\nK,11,ITD/2,-EH-PT,,!最下面\nK,12,OTD/2,-EH-PT,,\nK,13,OTD/2,-EH+TT,,\nK,14,ITD/2,-EH+TT,,\nK,15,IAD/2,ET,,\nK,16,IAD/2,0,,\nK,17,IAD/2,-AT+ET,,\nK,18,OAD/2,-AT+ET,,\n\nK,100,0,0,0,\nK,101,0,0.003,0,\n\nLSTR,1,2\nLSTR,2,3\nLSTR,3,4\nLSTR,4,5\nLSTR,5,6\nLSTR,6,7\nLSTR,7,8\nLSTR,8,1\nLSTR,3,11\nLSTR,11,12\nLSTR,12,4\nLSTR,5,13\nLSTR,13,14\nLSTR,14,6\nLSTR,2,7\nLSTR,8,15\nLSTR,15,16\nLSTR,1,16\nLSTR,16,17\nLSTR,17,18\nLSTR,1,18\n\nAL,1,15,7,8\nAL,15,2,3,4,5,6,\nAL,9,10,11,3\nAL,5,12,13,14\nAL,8,16,17,18\nAL,18,19,20,21\n\nVROTAT,1,2,3,4, , ,100,101 ,360/FK, , !!!!!\nVROTAT,5,6, , , , ,100,101 ,360/FK, , !!!!!\nBLC4,0,TT-EH,OTD,-TH,TW !建立长方体\nVGEN, ,7, , , , ,-TW/2, , ,1!复制创建体  \nVOVLAP,4,7 !布尔操作\nVDELE,10, , ,1!删除体\nVSYMM,Z,8, , , ,0,0 !体镜像 \n\n!建立齿槽\nCSYS,5  \nWPSTYLE,,,,,,,,0\nVGEN,NZ/FK+1,4, , , ,360/NZ, , ,0  \nVGEN,NZ/FK+1,8, , , ,360/NZ, , ,0  \nVOVLAP,ALL\n*DO,I,1,NZ/FK+1\nCSYS,0\nVSEL,S,LOC,Y,TT-EH-TH/1.5,1\nCSYS,5\nVSEL,R,LOC,Y,(I-1)*360/NZ-TW/2/3.1415/ITD*360,TW/2/3.1415/ITD*360+(I-1)*360/NZ!选择体\nVDELE,ALL, , ,1\nALLSEL,ALL \n*ENDDO\n\n!旋转成体\nEPLOT \nCSYS,5 \nVGEN,FK,ALL, , , ,360/FK, , ,0 \n\n!Glue体\nVGLUE,ALL\n\n!添加材料属性\nALLSEL,ALL\nCSYS,0\nVSEL,S,LOC,Y,0,TT-EH\nVATT,       1, ,   1,       0   \nCSYS,5\nVSEL,S,LOC,X,0,OAD/2\nVATT,       1, ,   1,       0 \n\nALLSEL,ALL\nCSYS,0\nVSEL,R,LOC,Y,-EH-PT,-EH\nVATT,       2, ,  2,       0  \nALLSEL,ALL\n\n!网格体\nCSYS,0\nVSEL,R,LOC,Y,-EH-PT,-EH\nVSWEEP,ALL\n\nCSYS,0\nALLSEL,ALL \nVSEL,S,MAT,,1\nSMRT,6  \nSMRT,5  \nSMRT,4  \nMSHAPE,1,3d\nMSHKEY,0\nVMESH,ALL\n\nALLSEL,ALL\n\n!模态分析 \n/SOL  \nANTYPE,2\nMODOPT,LANB,22  \nEQSLV,SPAR  \nMXPAND,0, , ,0  \nLUMPM,0 \nPSTRES,0\nMODOPT,LANB,22,0,80000, ,OFF\n\nCSYS,5\nASEL,S,LOC,X,-IAD/2,IAD/2   \nDA,ALL,ALL,\nALLSEL,ALL\n\n!OUTPR,BASIC,ALL,  \n!OUTRES,ALL,ALL,\n \n/STATUS,SOLU\nSOLVE   \nFINISH\nCSYS,0\nALLSEL,ALL\n\n/POST1  \nSET,FIRST   \n/EFACET,1   \nPLNSOL, U,SUM, 2,1.0 !无轮廓2变0\n/post1\n*do,i,8,22\nset,1,i\n/VIEW,1,1,2,3   \n/ANG,1  \n/REP,FAST  \n/show,jpeg,,\nplnsol,u,sum,0,1.0\n/show,close\n*enddo\nFINISH\n\n!振幅仿真\n/SOL\nANTYPE,3\nHROPT,FULL  \nHROUT,ON\nLUMPM,0 \nEQSLV, ,0,  \nPSTRES,0\n\n!阻尼特性\nALPHAD,0,   \nBETAD,0,\nDMPSTR,0.005,   \n\n!压电耦合\n*do,i,1,(BS-1)\nALLSEL,ALL\ncsys,5\nnsel,S,LOC,X,ITD/2,OTD/2\ncsys,0\nnsel,R,loc,y,-eh-eq-pt\ncsys,5\nangle=360/BS\nnsel,r,loc,y,(i-1)*angle/2,i*angle/2\nb=1/2*(1-(-1)**i)*1\nc=1/2*(1-(-1)**(i+1))*1\nD,All,VOLT,b,c\n*enddo\n\nALLSEL,ALL\ncsys,5\nnsel,S,LOC,X,ITD/2,OTD/2\ncsys,0\nnsel,R,loc,y,-eh-eq-pt\ncsys,5\nangle=360/BS\nnsel,r,loc,y,(BS-1)*angle/2,((BS-1)*angle/2+3*angle/8)\nD,All,VOLT,(1/2*(1-(-1)**BS)*1),(1/2*(1-(-1)**(BS+1))*1)\n\nALLSEL,ALL\ncsys,5\nnsel,S,LOC,X,ITD/2,OTD/2\ncsys,0\nnsel,R,loc,y,-eh-eq-pt\ncsys,5\nangle=360/BS\nnsel,r,loc,y,((BS-1)*angle/2+3*angle/8),((BS-1)*angle/2+3*angle/4)\nD,All,VOLT,(1/2*(1-(-1)**(BS+1))*1),(1/2*(1-(-1)**(BS+2))*1)\n\n*do,i,1,(BS-1)\nALLSEL,ALL\ncsys,5\nnsel,S,LOC,X,ITD/2,OTD/2\ncsys,0\nnsel,R,loc,y,-eh-eq-pt\ncsys,5\nangle=360/BS\nnsel,r,loc,y,((BS-1)*angle/2+3*angle/4+(i-1)*angle/2),((BS-1)*angle/2+3*angle/4+(i)*angle/2)\ne=1/2*(1-(-1)**(BS+1+i))*1\nf=1/2*(1-(-1)**(BS+2+i))*1\nD,All,VOLT,e,f\n*enddo\n\nALLSEL,ALL\ncsys,5\nnsel,S,LOC,X,ITD/2,OTD/2\ncsys,0\nnsel,r,loc,y,-eh-eq\nD,All,VOLT,0,0\nALLSEL,ALL \n\nHARFRQ,26000,76000, \nNSUBST,5,  \nKBC,1\n/STATUS,SOLU\nSOLVE\n\n!选最大位移点\n/POST1\nNSORT,U,SUM,0,1, ,SELECT  \nPRNSOL,U,Z\n*get,node,SORT,0,IMAX\n\n!结果显示,打开后处理器\n/POST26 \nFILE,'finaltest','rst','.'   \n/UI,COLL,1  \nNUMVAR,200  \nSOLU,191,NCMIT  \nSTORE,MERGE \nPLCPLX,0\nPRCPLX,1\nFILLDATA,191,,,,1,1 \nREALVAR,191,191 \n\n!z方向位移 \nNSOL,2,node,U,Z, UZ_2, \nSTORE,MERGE \n\n!保存为txt(excel也行)\n/post26\n! Save time history variables to file zmovement.prn\n*CREATE,scratch,gui \n*DEL,_P26_EXPORT\n*DIM,_P26_EXPORT,TABLE,5,2 \nVGET,_P26_EXPORT(1,0),1 \nVGET,_P26_EXPORT(1,1),2,,0  \nVGET,_P26_EXPORT(1,2),2,,1  \n/OUTPUT,'zmovement','prn','.'  \n*VWRITE,'FREQ','UZ_2',' '   \n%14C %14C %14C\n*VWRITE,' ','REAL','IMAGINARY'  \n%14C %14C %14C  \n*VWRITE,_P26_EXPORT(1,0),_P26_EXPORT(1,1),_P26_EXPORT(1,2)  \n%14.5G %14.5G %14.5G\n/OUTPUT,TERM\n*END\n/INPUT,scratch,gui  \n! End of time history save  \n\n!x方向位移 \nNSOL,3,node,U,X, UX_3, \nSTORE,MERGE \n\n!保存为txt(excel也行)\n/post26\n! Save time history variables to file xmovement.prn\n*CREATE,scratch,gui \n*DEL,_P26_EXPORT\n*DIM,_P26_EXPORT,TABLE,5,2 \nVGET,_P26_EXPORT(1,0),1 \nVGET,_P26_EXPORT(1,1),3,,0  \nVGET,_P26_EXPORT(1,2),3,,1  \n/OUTPUT,'xmovement','prn','.'  \n*VWRITE,'FREQ','UX_3',' '   \n%14C %14C %14C  \n*VWRITE,' ','REAL','IMAGINARY'  \n%14C %14C %14C  \n*VWRITE,_P26_EXPORT(1,0),_P26_EXPORT(1,1),_P26_EXPORT(1,2)  \n%14.5G %14.5G %14.5G\n/OUTPUT,TERM\n*END\n/INPUT,scratch,gui  \n! End of time history save\n\n!y方向位移 \nNSOL,4,node,U,Y, UY_4, \nSTORE,MERGE \n\n!保存为txt(excel也行)\n/post26\n! Save time history variables to file ymovement.prn\n*CREATE,scratch,gui \n*DEL,_P26_EXPORT\n*DIM,_P26_EXPORT,TABLE,5,2 \nVGET,_P26_EXPORT(1,0),1 \nVGET,_P26_EXPORT(1,1),4,,0  \nVGET,_P26_EXPORT(1,2),4,,1  \n/OUTPUT,'ymovement','prn','.'  \n*VWRITE,'FREQ','UY_4',' '   \n%14C %14C %14C  \n*VWRITE,' ','REAL','IMAGINARY'  \n%14C %14C %14C  \n*VWRITE,_P26_EXPORT(1,0),_P26_EXPORT(1,1),_P26_EXPORT(1,2)  \n%14.5G %14.5G %14.5G\n/OUTPUT,TERM\n*END\n/INPUT,scratch,gui  \n! End of time history save\n\n!选择电流点\nRFORCE,2,180,AMPS,, AMPS_2  \nSTORE,MERGE \nFILLDATA,192,,,,0,0 \nFILLDATA,193,,,,1,0 \nFILLDATA,194,,,,-1,0\nFILLDATA,195,,,,1,1 \nVARNAME,195,NSET\n! Name: Z   \n! ID:  3\n! Function: 1/{AMPS_2}  \nFILLDATA,199,,,,1,0 \nREALVAR,199,199 \nQUOT,3,199,2,,Z \nSTORE,MERGE \n\n!保存为txt(excel也行)\n/post26\n! Save time history variables to file current.prn   \n*CREATE,scratch,gui \n*DEL,_P26_EXPORT\n*DIM,_P26_EXPORT,TABLE,5,2 \nVGET,_P26_EXPORT(1,0),1 \nVGET,_P26_EXPORT(1,1),3,,0  \nVGET,_P26_EXPORT(1,2),3,,1  \n/OUTPUT,'current','prn','.' \n*VWRITE,'FREQ','Z',' '  \n%14C %14C %14C  \n*VWRITE,' ','REAL','IMAGINARY'  \n%14C %14C %14C  \n*VWRITE,_P26_EXPORT(1,0),_P26_EXPORT(1,1),_P26_EXPORT(1,2)  \n%14.5G %14.5G %14.5G\n/OUTPUT,TERM\n*END\n/INPUT,scratch,gui  \n! End of time history save " ("字符串")) -> (w867:string)
        n119 = Write to Text File(file (use dialog)=w868, text=w867) -> ()  [unwired: 2 in, 3 out]
      }
      event "6": Value Change {
        n120 = event-data() -> ()  [unwired: 1 in, 6 out]
        n121 = Number To Fractional String(number="齿槽宽") -> (F-format string=w871:string)  [unwired: 3 in]
        n122 = Open/Create/Replace File(file path (use dialog)=path "H:/新/finaltest.dat" ("文件路径（使用对话框）"), operation (0:open)=T1."replace" ("操作(0:open)")) -> (refnum out=w876:refnum<file>)  [unwired: 4 in, 2 out]
        n123 = Concatenate Strings("/RGB,INDEX,100,100,100, 0   \n/RGB,INDEX, 80, 80, 80,13   \n/RGB,INDEX, 60, 60, 60,14   \n/RGB,INDEX, 0, 0, 0,15  \n\n/REPLOT,RESIZE  \n/CLEAR,NOSTART \nNZ=25 !齿数：\nTH=1.5 !平均齿高：\nWTH=1.5 !外侧斜齿高\nNTH=1.5 !内侧斜齿高\nWDTH=0.0 !齿外侧导角高度\nWDTL=0.0 !齿外侧导水平长度\nNDTH=0.0 !齿内侧导角高度\nNDTL=0.0 !齿内侧导水平长度\nTT=2 !齿厚：\nTW=" ("字符串"), w871, " !齿槽宽：\nITD=8 !定子齿内圈直径：\nOTD=13.3 !定子齿外圈直径：\nIAD=2.1 !轴内圈直径：\nOAD=6 !轴外圈直径：\nAT=1.6 !轴厚度\nPT=0.4 !压电片厚：\nIPD=8 !压电片内圈直径：\nOPD=13.3 !压电片外圈直径：\nEW= ITD-OAD !宽度：\nET=0.2 !厚度：\nEH=0.2 !台阶高：\nBS=4 !波数\nFK=5 !定子分块建模分块数与齿数成整数倍的关系 \n\nNZ=NZ !齿数：\nTH=TH/1000 !齿高：\nWTH=WTH/1000 !外侧斜齿高\nNTH=NTH/1000 !内侧斜齿高\nWDTH=WDTH/1000 !齿外侧导角高度\nWDTL=WDTL/1000 !齿外侧导水平长度\nNDTH=NDTH/1000 !齿内侧导角高度\nNDTL=NDTL/1000 !齿内侧导水平长度\nTT=TT/1000 !齿厚：\nTW=TW/1000 !齿槽宽：\nITD=ITD/1000 !定子齿内圈直径：\nOTD=OTD/1000 !定子齿外圈直径：\nIAD=IAD/1000 !轴内圈直径：\nOAD=OAD/1000 !轴外圈直径：\nAT=AT/1000 !轴厚度\nPT=PT/1000 !压电片厚：\nIPD=IPD/1000 !压电片内圈直径：\nOPD=OPD/1000 !压电片外圈直径：\nEW= EW/1000 !宽度：\nET=ET/1000 !厚度：\nEH=EH/1000 !台阶高：\n\n/PREP7 \n!定义单元和材料属性\nET,1,SOLID185   \nMPTEMP,,,,,,,,  \nMPTEMP,1,0  \nMPDATA,DENS,1,,8290\nMPTEMP,,,,,,,,  \nMPTEMP,1,0  \nMPDATA,EX,1,,1.06E+011   \nMPDATA,PRXY,1,,0.35 \n\nET,2,SOLID5 \nMPTEMP,,,,,,,,  \nMPTEMP,1,0     \nMPDATA,DENS,2,,7750   \nMPTEMP,,,,,,,,  \nMPTEMP,1,0  \nMPDATA,PERX,2,,919E-009\nMPDATA,PERY,2,,919E-009   \nMPDATA,PERZ,2,,826E-009\nTB,PIEZ,2,,,0   \nTBMODIF,1,1,0   \nTBMODIF,1,2,0   \nTBMODIF,1,3,-5.35   \nTBMODIF,2,1,0   \nTBMODIF,2,2,0   \nTBMODIF,2,3,-5.35   \nTBMODIF,3,1,0   \nTBMODIF,3,2,0   \nTBMODIF,3,3,15.78   \nTBMODIF,4,1,0   \nTBMODIF,4,2,0   \nTBMODIF,4,3,0   \nTBMODIF,5,1,0   \nTBMODIF,5,2,12.3\nTBMODIF,5,3,0   \nTBMODIF,6,1,12.3\nTBMODIF,6,2,0   \nTBMODIF,6,3,0   \nTB,ANEL,2,1,21,0\nTBTEMP,0\nTBDATA,,1.2035E+011,7.52E+010,7.51E+010,0,0,0   \nTBDATA,,1.204E+011,7.51E+010,0,0,0,1.109E+011   \nTBDATA,,0,0,0,2.26E+010,0,0 \nTBDATA,,2.12E+010,0,2.11E+010,,,\n\n!超声波电机模型建立\nK,1,OAD/2,,,\nK,2,ITD/2,,,\nK,3,ITD/2,-EH,,!最上面\nK,4,OTD/2,-EH,,\nK,5,OTD/2,-EH+TT-TH,,\nK,6,ITD/2,-EH+TT-TH,,\nK,7,ITD/2,ET,,\nK,8,OAD/2,ET,,\nK,11,ITD/2,-EH-PT,,!最下面\nK,12,OTD/2,-EH-PT,,\nK,13,OTD/2,-EH+TT,,\nK,14,ITD/2,-EH+TT,,\nK,15,IAD/2,ET,,\nK,16,IAD/2,0,,\nK,17,IAD/2,-AT+ET,,\nK,18,OAD/2,-AT+ET,,\n\nK,100,0,0,0,\nK,101,0,0.003,0,\n\nLSTR,1,2\nLSTR,2,3\nLSTR,3,4\nLSTR,4,5\nLSTR,5,6\nLSTR,6,7\nLSTR,7,8\nLSTR,8,1\nLSTR,3,11\nLSTR,11,12\nLSTR,12,4\nLSTR,5,13\nLSTR,13,14\nLSTR,14,6\nLSTR,2,7\nLSTR,8,15\nLSTR,15,16\nLSTR,1,16\nLSTR,16,17\nLSTR,17,18\nLSTR,1,18\n\nAL,1,15,7,8\nAL,15,2,3,4,5,6,\nAL,9,10,11,3\nAL,5,12,13,14\nAL,8,16,17,18\nAL,18,19,20,21\n\nVROTAT,1,2,3,4, , ,100,101 ,360/FK, , !!!!!\nVROTAT,5,6, , , , ,100,101 ,360/FK, , !!!!!\nBLC4,0,TT-EH,OTD,-TH,TW !建立长方体\nVGEN, ,7, , , , ,-TW/2, , ,1!复制创建体  \nVOVLAP,4,7 !布尔操作\nVDELE,10, , ,1!删除体\nVSYMM,Z,8, , , ,0,0 !体镜像 \n\n!建立齿槽\nCSYS,5  \nWPSTYLE,,,,,,,,0\nVGEN,NZ/FK+1,4, , , ,360/NZ, , ,0  \nVGEN,NZ/FK+1,8, , , ,360/NZ, , ,0  \nVOVLAP,ALL\n*DO,I,1,NZ/FK+1\nCSYS,0\nVSEL,S,LOC,Y,TT-EH-TH/1.5,1\nCSYS,5\nVSEL,R,LOC,Y,(I-1)*360/NZ-TW/2/3.1415/ITD*360,TW/2/3.1415/ITD*360+(I-1)*360/NZ!选择体\nVDELE,ALL, , ,1\nALLSEL,ALL \n*ENDDO\n\n!旋转成体\nEPLOT \nCSYS,5 \nVGEN,FK,ALL, , , ,360/FK, , ,0 \n\n!Glue体\nVGLUE,ALL\n\n!添加材料属性\nALLSEL,ALL\nCSYS,0\nVSEL,S,LOC,Y,0,TT-EH\nVATT,       1, ,   1,       0   \nCSYS,5\nVSEL,S,LOC,X,0,OAD/2\nVATT,       1, ,   1,       0 \n\nALLSEL,ALL\nCSYS,0\nVSEL,R,LOC,Y,-EH-PT,-EH\nVATT,       2, ,  2,       0  \nALLSEL,ALL\n\n!网格体\nCSYS,0\nVSEL,R,LOC,Y,-EH-PT,-EH\nVSWEEP,ALL\n\nCSYS,0\nALLSEL,ALL \nVSEL,S,MAT,,1\nSMRT,6  \nSMRT,5  \nSMRT,4  \nMSHAPE,1,3d\nMSHKEY,0\nVMESH,ALL\n\nALLSEL,ALL\n\n!模态分析 \n/SOL  \nANTYPE,2\nMODOPT,LANB,22  \nEQSLV,SPAR  \nMXPAND,0, , ,0  \nLUMPM,0 \nPSTRES,0\nMODOPT,LANB,22,0,80000, ,OFF\n\nCSYS,5\nASEL,S,LOC,X,-IAD/2,IAD/2   \nDA,ALL,ALL,\nALLSEL,ALL\n\n!OUTPR,BASIC,ALL,  \n!OUTRES,ALL,ALL,\n \n/STATUS,SOLU\nSOLVE   \nFINISH\nCSYS,0\nALLSEL,ALL\n\n/POST1  \nSET,FIRST   \n/EFACET,1   \nPLNSOL, U,SUM, 2,1.0 !无轮廓2变0\n/post1\n*do,i,8,22\nset,1,i\n/VIEW,1,1,2,3   \n/ANG,1  \n/REP,FAST  \n/show,jpeg,,\nplnsol,u,sum,0,1.0\n/show,close\n*enddo\nFINISH\n\n!振幅仿真\n/SOL\nANTYPE,3\nHROPT,FULL  \nHROUT,ON\nLUMPM,0 \nEQSLV, ,0,  \nPSTRES,0\n\n!阻尼特性\nALPHAD,0,   \nBETAD,0,\nDMPSTR,0.005,   \n\n!压电耦合\n*do,i,1,(BS-1)\nALLSEL,ALL\ncsys,5\nnsel,S,LOC,X,ITD/2,OTD/2\ncsys,0\nnsel,R,loc,y,-eh-eq-pt\ncsys,5\nangle=360/BS\nnsel,r,loc,y,(i-1)*angle/2,i*angle/2\nb=1/2*(1-(-1)**i)*1\nc=1/2*(1-(-1)**(i+1))*1\nD,All,VOLT,b,c\n*enddo\n\nALLSEL,ALL\ncsys,5\nnsel,S,LOC,X,ITD/2,OTD/2\ncsys,0\nnsel,R,loc,y,-eh-eq-pt\ncsys,5\nangle=360/BS\nnsel,r,loc,y,(BS-1)*angle/2,((BS-1)*angle/2+3*angle/8)\nD,All,VOLT,(1/2*(1-(-1)**BS)*1),(1/2*(1-(-1)**(BS+1))*1)\n\nALLSEL,ALL\ncsys,5\nnsel,S,LOC,X,ITD/2,OTD/2\ncsys,0\nnsel,R,loc,y,-eh-eq-pt\ncsys,5\nangle=360/BS\nnsel,r,loc,y,((BS-1)*angle/2+3*angle/8),((BS-1)*angle/2+3*angle/4)\nD,All,VOLT,(1/2*(1-(-1)**(BS+1))*1),(1/2*(1-(-1)**(BS+2))*1)\n\n*do,i,1,(BS-1)\nALLSEL,ALL\ncsys,5\nnsel,S,LOC,X,ITD/2,OTD/2\ncsys,0\nnsel,R,loc,y,-eh-eq-pt\ncsys,5\nangle=360/BS\nnsel,r,loc,y,((BS-1)*angle/2+3*angle/4+(i-1)*angle/2),((BS-1)*angle/2+3*angle/4+(i)*angle/2)\ne=1/2*(1-(-1)**(BS+1+i))*1\nf=1/2*(1-(-1)**(BS+2+i))*1\nD,All,VOLT,e,f\n*enddo\n\nALLSEL,ALL\ncsys,5\nnsel,S,LOC,X,ITD/2,OTD/2\ncsys,0\nnsel,r,loc,y,-eh-eq\nD,All,VOLT,0,0\nALLSEL,ALL \n\nHARFRQ,26000,76000, \nNSUBST,5,  \nKBC,1\n/STATUS,SOLU\nSOLVE\n\n!选最大位移点\n/POST1\nNSORT,U,SUM,0,1, ,SELECT  \nPRNSOL,U,Z\n*get,node,SORT,0,IMAX\n\n!结果显示,打开后处理器\n/POST26 \nFILE,'finaltest','rst','.'   \n/UI,COLL,1  \nNUMVAR,200  \nSOLU,191,NCMIT  \nSTORE,MERGE \nPLCPLX,0\nPRCPLX,1\nFILLDATA,191,,,,1,1 \nREALVAR,191,191 \n\n!z方向位移 \nNSOL,2,node,U,Z, UZ_2, \nSTORE,MERGE \n\n!保存为txt(excel也行)\n/post26\n! Save time history variables to file zmovement.prn\n*CREATE,scratch,gui \n*DEL,_P26_EXPORT\n*DIM,_P26_EXPORT,TABLE,5,2 \nVGET,_P26_EXPORT(1,0),1 \nVGET,_P26_EXPORT(1,1),2,,0  \nVGET,_P26_EXPORT(1,2),2,,1  \n/OUTPUT,'zmovement','prn','.'  \n*VWRITE,'FREQ','UZ_2',' '   \n%14C %14C %14C\n*VWRITE,' ','REAL','IMAGINARY'  \n%14C %14C %14C  \n*VWRITE,_P26_EXPORT(1,0),_P26_EXPORT(1,1),_P26_EXPORT(1,2)  \n%14.5G %14.5G %14.5G\n/OUTPUT,TERM\n*END\n/INPUT,scratch,gui  \n! End of time history save  \n\n!x方向位移 \nNSOL,3,node,U,X, UX_3, \nSTORE,MERGE \n\n!保存为txt(excel也行)\n/post26\n! Save time history variables to file xmovement.prn\n*CREATE,scratch,gui \n*DEL,_P26_EXPORT\n*DIM,_P26_EXPORT,TABLE,5,2 \nVGET,_P26_EXPORT(1,0),1 \nVGET,_P26_EXPORT(1,1),3,,0  \nVGET,_P26_EXPORT(1,2),3,,1  \n/OUTPUT,'xmovement','prn','.'  \n*VWRITE,'FREQ','UX_3',' '   \n%14C %14C %14C  \n*VWRITE,' ','REAL','IMAGINARY'  \n%14C %14C %14C  \n*VWRITE,_P26_EXPORT(1,0),_P26_EXPORT(1,1),_P26_EXPORT(1,2)  \n%14.5G %14.5G %14.5G\n/OUTPUT,TERM\n*END\n/INPUT,scratch,gui  \n! End of time history save\n\n!y方向位移 \nNSOL,4,node,U,Y, UY_4, \nSTORE,MERGE \n\n!保存为txt(excel也行)\n/post26\n! Save time history variables to file ymovement.prn\n*CREATE,scratch,gui \n*DEL,_P26_EXPORT\n*DIM,_P26_EXPORT,TABLE,5,2 \nVGET,_P26_EXPORT(1,0),1 \nVGET,_P26_EXPORT(1,1),4,,0  \nVGET,_P26_EXPORT(1,2),4,,1  \n/OUTPUT,'ymovement','prn','.'  \n*VWRITE,'FREQ','UY_4',' '   \n%14C %14C %14C  \n*VWRITE,' ','REAL','IMAGINARY'  \n%14C %14C %14C  \n*VWRITE,_P26_EXPORT(1,0),_P26_EXPORT(1,1),_P26_EXPORT(1,2)  \n%14.5G %14.5G %14.5G\n/OUTPUT,TERM\n*END\n/INPUT,scratch,gui  \n! End of time history save\n\n!选择电流点\nRFORCE,2,180,AMPS,, AMPS_2  \nSTORE,MERGE \nFILLDATA,192,,,,0,0 \nFILLDATA,193,,,,1,0 \nFILLDATA,194,,,,-1,0\nFILLDATA,195,,,,1,1 \nVARNAME,195,NSET\n! Name: Z   \n! ID:  3\n! Function: 1/{AMPS_2}  \nFILLDATA,199,,,,1,0 \nREALVAR,199,199 \nQUOT,3,199,2,,Z \nSTORE,MERGE \n\n!保存为txt(excel也行)\n/post26\n! Save time history variables to file current.prn   \n*CREATE,scratch,gui \n*DEL,_P26_EXPORT\n*DIM,_P26_EXPORT,TABLE,5,2 \nVGET,_P26_EXPORT(1,0),1 \nVGET,_P26_EXPORT(1,1),3,,0  \nVGET,_P26_EXPORT(1,2),3,,1  \n/OUTPUT,'current','prn','.' \n*VWRITE,'FREQ','Z',' '  \n%14C %14C %14C  \n*VWRITE,' ','REAL','IMAGINARY'  \n%14C %14C %14C  \n*VWRITE,_P26_EXPORT(1,0),_P26_EXPORT(1,1),_P26_EXPORT(1,2)  \n%14.5G %14.5G %14.5G\n/OUTPUT,TERM\n*END\n/INPUT,scratch,gui  \n! End of time history save " ("字符串")) -> (w875:string)
        n124 = Write to Text File(file (use dialog)=w876, text=w875) -> ()  [unwired: 2 in, 3 out]
      }
      event "7": Value Change {
        n125 = event-data() -> ()  [unwired: 1 in, 6 out]
        n126 = Number To Fractional String(number="定子齿内圈直径") -> (F-format string=w879:string)  [unwired: 3 in]
        n127 = Open/Create/Replace File(file path (use dialog)=path "H:/新/finaltest.dat" ("文件路径（使用对话框）"), operation (0:open)=T1."replace" ("操作(0:open)")) -> (refnum out=w884:refnum<file>)  [unwired: 4 in, 2 out]
        n128 = Concatenate Strings("/RGB,INDEX,100,100,100, 0   \n/RGB,INDEX, 80, 80, 80,13   \n/RGB,INDEX, 60, 60, 60,14   \n/RGB,INDEX, 0, 0, 0,15  \n\n/REPLOT,RESIZE  \n/CLEAR,NOSTART \nNZ=25 !齿数：\nTH=1.5 !平均齿高：\nWTH=1.5 !外侧斜齿高\nNTH=1.5 !内侧斜齿高\nWDTH=0.0 !齿外侧导角高度\nWDTL=0.0 !齿外侧导水平长度\nNDTH=0.0 !齿内侧导角高度\nNDTL=0.0 !齿内侧导水平长度\nTT=2 !齿厚：\nTW=0.1 !齿槽宽：\nITD=" ("字符串"), w879, " !定子齿内圈直径：\nOTD=13.3 !定子齿外圈直径：\nIAD=2.1 !轴内圈直径：\nOAD=6 !轴外圈直径：\nAT=1.6 !轴厚度\nPT=0.4 !压电片厚：\nIPD=8 !压电片内圈直径：\nOPD=13.3 !压电片外圈直径：\nEW= ITD-OAD !宽度：\nET=0.2 !厚度：\nEH=0.2 !台阶高：\nBS=4 !波数\nFK=5 !定子分块建模分块数与齿数成整数倍的关系 \n\nNZ=NZ !齿数：\nTH=TH/1000 !齿高：\nWTH=WTH/1000 !外侧斜齿高\nNTH=NTH/1000 !内侧斜齿高\nWDTH=WDTH/1000 !齿外侧导角高度\nWDTL=WDTL/1000 !齿外侧导水平长度\nNDTH=NDTH/1000 !齿内侧导角高度\nNDTL=NDTL/1000 !齿内侧导水平长度\nTT=TT/1000 !齿厚：\nTW=TW/1000 !齿槽宽：\nITD=ITD/1000 !定子齿内圈直径：\nOTD=OTD/1000 !定子齿外圈直径：\nIAD=IAD/1000 !轴内圈直径：\nOAD=OAD/1000 !轴外圈直径：\nAT=AT/1000 !轴厚度\nPT=PT/1000 !压电片厚：\nIPD=IPD/1000 !压电片内圈直径：\nOPD=OPD/1000 !压电片外圈直径：\nEW= EW/1000 !宽度：\nET=ET/1000 !厚度：\nEH=EH/1000 !台阶高：\n\n/PREP7 \n!定义单元和材料属性\nET,1,SOLID185   \nMPTEMP,,,,,,,,  \nMPTEMP,1,0  \nMPDATA,DENS,1,,8290\nMPTEMP,,,,,,,,  \nMPTEMP,1,0  \nMPDATA,EX,1,,1.06E+011   \nMPDATA,PRXY,1,,0.35 \n\nET,2,SOLID5 \nMPTEMP,,,,,,,,  \nMPTEMP,1,0     \nMPDATA,DENS,2,,7750   \nMPTEMP,,,,,,,,  \nMPTEMP,1,0  \nMPDATA,PERX,2,,919E-009\nMPDATA,PERY,2,,919E-009   \nMPDATA,PERZ,2,,826E-009\nTB,PIEZ,2,,,0   \nTBMODIF,1,1,0   \nTBMODIF,1,2,0   \nTBMODIF,1,3,-5.35   \nTBMODIF,2,1,0   \nTBMODIF,2,2,0   \nTBMODIF,2,3,-5.35   \nTBMODIF,3,1,0   \nTBMODIF,3,2,0   \nTBMODIF,3,3,15.78   \nTBMODIF,4,1,0   \nTBMODIF,4,2,0   \nTBMODIF,4,3,0   \nTBMODIF,5,1,0   \nTBMODIF,5,2,12.3\nTBMODIF,5,3,0   \nTBMODIF,6,1,12.3\nTBMODIF,6,2,0   \nTBMODIF,6,3,0   \nTB,ANEL,2,1,21,0\nTBTEMP,0\nTBDATA,,1.2035E+011,7.52E+010,7.51E+010,0,0,0   \nTBDATA,,1.204E+011,7.51E+010,0,0,0,1.109E+011   \nTBDATA,,0,0,0,2.26E+010,0,0 \nTBDATA,,2.12E+010,0,2.11E+010,,,\n\n!超声波电机模型建立\nK,1,OAD/2,,,\nK,2,ITD/2,,,\nK,3,ITD/2,-EH,,!最上面\nK,4,OTD/2,-EH,,\nK,5,OTD/2,-EH+TT-TH,,\nK,6,ITD/2,-EH+TT-TH,,\nK,7,ITD/2,ET,,\nK,8,OAD/2,ET,,\nK,11,ITD/2,-EH-PT,,!最下面\nK,12,OTD/2,-EH-PT,,\nK,13,OTD/2,-EH+TT,,\nK,14,ITD/2,-EH+TT,,\nK,15,IAD/2,ET,,\nK,16,IAD/2,0,,\nK,17,IAD/2,-AT+ET,,\nK,18,OAD/2,-AT+ET,,\n\nK,100,0,0,0,\nK,101,0,0.003,0,\n\nLSTR,1,2\nLSTR,2,3\nLSTR,3,4\nLSTR,4,5\nLSTR,5,6\nLSTR,6,7\nLSTR,7,8\nLSTR,8,1\nLSTR,3,11\nLSTR,11,12\nLSTR,12,4\nLSTR,5,13\nLSTR,13,14\nLSTR,14,6\nLSTR,2,7\nLSTR,8,15\nLSTR,15,16\nLSTR,1,16\nLSTR,16,17\nLSTR,17,18\nLSTR,1,18\n\nAL,1,15,7,8\nAL,15,2,3,4,5,6,\nAL,9,10,11,3\nAL,5,12,13,14\nAL,8,16,17,18\nAL,18,19,20,21\n\nVROTAT,1,2,3,4, , ,100,101 ,360/FK, , !!!!!\nVROTAT,5,6, , , , ,100,101 ,360/FK, , !!!!!\nBLC4,0,TT-EH,OTD,-TH,TW !建立长方体\nVGEN, ,7, , , , ,-TW/2, , ,1!复制创建体  \nVOVLAP,4,7 !布尔操作\nVDELE,10, , ,1!删除体\nVSYMM,Z,8, , , ,0,0 !体镜像 \n\n!建立齿槽\nCSYS,5  \nWPSTYLE,,,,,,,,0\nVGEN,NZ/FK+1,4, , , ,360/NZ, , ,0  \nVGEN,NZ/FK+1,8, , , ,360/NZ, , ,0  \nVOVLAP,ALL\n*DO,I,1,NZ/FK+1\nCSYS,0\nVSEL,S,LOC,Y,TT-EH-TH/1.5,1\nCSYS,5\nVSEL,R,LOC,Y,(I-1)*360/NZ-TW/2/3.1415/ITD*360,TW/2/3.1415/ITD*360+(I-1)*360/NZ!选择体\nVDELE,ALL, , ,1\nALLSEL,ALL \n*ENDDO\n\n!旋转成体\nEPLOT \nCSYS,5 \nVGEN,FK,ALL, , , ,360/FK, , ,0 \n\n!Glue体\nVGLUE,ALL\n\n!添加材料属性\nALLSEL,ALL\nCSYS,0\nVSEL,S,LOC,Y,0,TT-EH\nVATT,       1, ,   1,       0   \nCSYS,5\nVSEL,S,LOC,X,0,OAD/2\nVATT,       1, ,   1,       0 \n\nALLSEL,ALL\nCSYS,0\nVSEL,R,LOC,Y,-EH-PT,-EH\nVATT,       2, ,  2,       0  \nALLSEL,ALL\n\n!网格体\nCSYS,0\nVSEL,R,LOC,Y,-EH-PT,-EH\nVSWEEP,ALL\n\nCSYS,0\nALLSEL,ALL \nVSEL,S,MAT,,1\nSMRT,6  \nSMRT,5  \nSMRT,4  \nMSHAPE,1,3d\nMSHKEY,0\nVMESH,ALL\n\nALLSEL,ALL\n\n!模态分析 \n/SOL  \nANTYPE,2\nMODOPT,LANB,22  \nEQSLV,SPAR  \nMXPAND,0, , ,0  \nLUMPM,0 \nPSTRES,0\nMODOPT,LANB,22,0,80000, ,OFF\n\nCSYS,5\nASEL,S,LOC,X,-IAD/2,IAD/2   \nDA,ALL,ALL,\nALLSEL,ALL\n\n!OUTPR,BASIC,ALL,  \n!OUTRES,ALL,ALL,\n \n/STATUS,SOLU\nSOLVE   \nFINISH\nCSYS,0\nALLSEL,ALL\n\n/POST1  \nSET,FIRST   \n/EFACET,1   \nPLNSOL, U,SUM, 2,1.0 !无轮廓2变0\n/post1\n*do,i,8,22\nset,1,i\n/VIEW,1,1,2,3   \n/ANG,1  \n/REP,FAST  \n/show,jpeg,,\nplnsol,u,sum,0,1.0\n/show,close\n*enddo\nFINISH\n\n!振幅仿真\n/SOL\nANTYPE,3\nHROPT,FULL  \nHROUT,ON\nLUMPM,0 \nEQSLV, ,0,  \nPSTRES,0\n\n!阻尼特性\nALPHAD,0,   \nBETAD,0,\nDMPSTR,0.005,   \n\n!压电耦合\n*do,i,1,(BS-1)\nALLSEL,ALL\ncsys,5\nnsel,S,LOC,X,ITD/2,OTD/2\ncsys,0\nnsel,R,loc,y,-eh-eq-pt\ncsys,5\nangle=360/BS\nnsel,r,loc,y,(i-1)*angle/2,i*angle/2\nb=1/2*(1-(-1)**i)*1\nc=1/2*(1-(-1)**(i+1))*1\nD,All,VOLT,b,c\n*enddo\n\nALLSEL,ALL\ncsys,5\nnsel,S,LOC,X,ITD/2,OTD/2\ncsys,0\nnsel,R,loc,y,-eh-eq-pt\ncsys,5\nangle=360/BS\nnsel,r,loc,y,(BS-1)*angle/2,((BS-1)*angle/2+3*angle/8)\nD,All,VOLT,(1/2*(1-(-1)**BS)*1),(1/2*(1-(-1)**(BS+1))*1)\n\nALLSEL,ALL\ncsys,5\nnsel,S,LOC,X,ITD/2,OTD/2\ncsys,0\nnsel,R,loc,y,-eh-eq-pt\ncsys,5\nangle=360/BS\nnsel,r,loc,y,((BS-1)*angle/2+3*angle/8),((BS-1)*angle/2+3*angle/4)\nD,All,VOLT,(1/2*(1-(-1)**(BS+1))*1),(1/2*(1-(-1)**(BS+2))*1)\n\n*do,i,1,(BS-1)\nALLSEL,ALL\ncsys,5\nnsel,S,LOC,X,ITD/2,OTD/2\ncsys,0\nnsel,R,loc,y,-eh-eq-pt\ncsys,5\nangle=360/BS\nnsel,r,loc,y,((BS-1)*angle/2+3*angle/4+(i-1)*angle/2),((BS-1)*angle/2+3*angle/4+(i)*angle/2)\ne=1/2*(1-(-1)**(BS+1+i))*1\nf=1/2*(1-(-1)**(BS+2+i))*1\nD,All,VOLT,e,f\n*enddo\n\nALLSEL,ALL\ncsys,5\nnsel,S,LOC,X,ITD/2,OTD/2\ncsys,0\nnsel,r,loc,y,-eh-eq\nD,All,VOLT,0,0\nALLSEL,ALL \n\nHARFRQ,26000,76000, \nNSUBST,5,  \nKBC,1\n/STATUS,SOLU\nSOLVE\n\n!选最大位移点\n/POST1\nNSORT,U,SUM,0,1, ,SELECT  \nPRNSOL,U,Z\n*get,node,SORT,0,IMAX\n\n!结果显示,打开后处理器\n/POST26 \nFILE,'finaltest','rst','.'   \n/UI,COLL,1  \nNUMVAR,200  \nSOLU,191,NCMIT  \nSTORE,MERGE \nPLCPLX,0\nPRCPLX,1\nFILLDATA,191,,,,1,1 \nREALVAR,191,191 \n\n!z方向位移 \nNSOL,2,node,U,Z, UZ_2, \nSTORE,MERGE \n\n!保存为txt(excel也行)\n/post26\n! Save time history variables to file zmovement.prn\n*CREATE,scratch,gui \n*DEL,_P26_EXPORT\n*DIM,_P26_EXPORT,TABLE,5,2 \nVGET,_P26_EXPORT(1,0),1 \nVGET,_P26_EXPORT(1,1),2,,0  \nVGET,_P26_EXPORT(1,2),2,,1  \n/OUTPUT,'zmovement','prn','.'  \n*VWRITE,'FREQ','UZ_2',' '   \n%14C %14C %14C\n*VWRITE,' ','REAL','IMAGINARY'  \n%14C %14C %14C  \n*VWRITE,_P26_EXPORT(1,0),_P26_EXPORT(1,1),_P26_EXPORT(1,2)  \n%14.5G %14.5G %14.5G\n/OUTPUT,TERM\n*END\n/INPUT,scratch,gui  \n! End of time history save  \n\n!x方向位移 \nNSOL,3,node,U,X, UX_3, \nSTORE,MERGE \n\n!保存为txt(excel也行)\n/post26\n! Save time history variables to file xmovement.prn\n*CREATE,scratch,gui \n*DEL,_P26_EXPORT\n*DIM,_P26_EXPORT,TABLE,5,2 \nVGET,_P26_EXPORT(1,0),1 \nVGET,_P26_EXPORT(1,1),3,,0  \nVGET,_P26_EXPORT(1,2),3,,1  \n/OUTPUT,'xmovement','prn','.'  \n*VWRITE,'FREQ','UX_3',' '   \n%14C %14C %14C  \n*VWRITE,' ','REAL','IMAGINARY'  \n%14C %14C %14C  \n*VWRITE,_P26_EXPORT(1,0),_P26_EXPORT(1,1),_P26_EXPORT(1,2)  \n%14.5G %14.5G %14.5G\n/OUTPUT,TERM\n*END\n/INPUT,scratch,gui  \n! End of time history save\n\n!y方向位移 \nNSOL,4,node,U,Y, UY_4, \nSTORE,MERGE \n\n!保存为txt(excel也行)\n/post26\n! Save time history variables to file ymovement.prn\n*CREATE,scratch,gui \n*DEL,_P26_EXPORT\n*DIM,_P26_EXPORT,TABLE,5,2 \nVGET,_P26_EXPORT(1,0),1 \nVGET,_P26_EXPORT(1,1),4,,0  \nVGET,_P26_EXPORT(1,2),4,,1  \n/OUTPUT,'ymovement','prn','.'  \n*VWRITE,'FREQ','UY_4',' '   \n%14C %14C %14C  \n*VWRITE,' ','REAL','IMAGINARY'  \n%14C %14C %14C  \n*VWRITE,_P26_EXPORT(1,0),_P26_EXPORT(1,1),_P26_EXPORT(1,2)  \n%14.5G %14.5G %14.5G\n/OUTPUT,TERM\n*END\n/INPUT,scratch,gui  \n! End of time history save\n\n!选择电流点\nRFORCE,2,180,AMPS,, AMPS_2  \nSTORE,MERGE \nFILLDATA,192,,,,0,0 \nFILLDATA,193,,,,1,0 \nFILLDATA,194,,,,-1,0\nFILLDATA,195,,,,1,1 \nVARNAME,195,NSET\n! Name: Z   \n! ID:  3\n! Function: 1/{AMPS_2}  \nFILLDATA,199,,,,1,0 \nREALVAR,199,199 \nQUOT,3,199,2,,Z \nSTORE,MERGE \n\n!保存为txt(excel也行)\n/post26\n! Save time history variables to file current.prn   \n*CREATE,scratch,gui \n*DEL,_P26_EXPORT\n*DIM,_P26_EXPORT,TABLE,5,2 \nVGET,_P26_EXPORT(1,0),1 \nVGET,_P26_EXPORT(1,1),3,,0  \nVGET,_P26_EXPORT(1,2),3,,1  \n/OUTPUT,'current','prn','.' \n*VWRITE,'FREQ','Z',' '  \n%14C %14C %14C  \n*VWRITE,' ','REAL','IMAGINARY'  \n%14C %14C %14C  \n*VWRITE,_P26_EXPORT(1,0),_P26_EXPORT(1,1),_P26_EXPORT(1,2)  \n%14.5G %14.5G %14.5G\n/OUTPUT,TERM\n*END\n/INPUT,scratch,gui  \n! End of time history save " ("字符串")) -> (w883:string)
        n129 = Write to Text File(file (use dialog)=w884, text=w883) -> ()  [unwired: 2 in, 3 out]
      }
      event "8": Value Change {
        n130 = event-data() -> ()  [unwired: 1 in, 6 out]
        n131 = Number To Fractional String(number="定子齿外圈直径") -> (F-format string=w887:string)  [unwired: 3 in]
        n132 = Open/Create/Replace File(file path (use dialog)=path "H:/新/finaltest.dat" ("文件路径（使用对话框）"), operation (0:open)=T1."replace" ("操作(0:open)")) -> (refnum out=w892:refnum<file>)  [unwired: 4 in, 2 out]
        n133 = Concatenate Strings("/RGB,INDEX,100,100,100, 0   \n/RGB,INDEX, 80, 80, 80,13   \n/RGB,INDEX, 60, 60, 60,14   \n/RGB,INDEX, 0, 0, 0,15  \n\n/REPLOT,RESIZE  \n/CLEAR,NOSTART \nNZ=25 !齿数：\nTH=1.5 !平均齿高：\nWTH=1.5 !外侧斜齿高\nNTH=1.5 !内侧斜齿高\nWDTH=0.0 !齿外侧导角高度\nWDTL=0.0 !齿外侧导水平长度\nNDTH=0.0 !齿内侧导角高度\nNDTL=0.0 !齿内侧导水平长度\nTT=2 !齿厚：\nTW=0.1 !齿槽宽：\nITD=8 !定子齿内圈直径：\nOTD=" ("字符串"), w887, " !定子齿外圈直径：\nIAD=2.1 !轴内圈直径：\nOAD=6 !轴外圈直径：\nAT=1.6 !轴厚度\nPT=0.4 !压电片厚：\nIPD=8 !压电片内圈直径：\nOPD=13.3 !压电片外圈直径：\nEW= ITD-OAD !宽度：\nET=0.2 !厚度：\nEH=0.2 !台阶高：\nBS=4 !波数\nFK=5 !定子分块建模分块数与齿数成整数倍的关系 \n\nNZ=NZ !齿数：\nTH=TH/1000 !齿高：\nWTH=WTH/1000 !外侧斜齿高\nNTH=NTH/1000 !内侧斜齿高\nWDTH=WDTH/1000 !齿外侧导角高度\nWDTL=WDTL/1000 !齿外侧导水平长度\nNDTH=NDTH/1000 !齿内侧导角高度\nNDTL=NDTL/1000 !齿内侧导水平长度\nTT=TT/1000 !齿厚：\nTW=TW/1000 !齿槽宽：\nITD=ITD/1000 !定子齿内圈直径：\nOTD=OTD/1000 !定子齿外圈直径：\nIAD=IAD/1000 !轴内圈直径：\nOAD=OAD/1000 !轴外圈直径：\nAT=AT/1000 !轴厚度\nPT=PT/1000 !压电片厚：\nIPD=IPD/1000 !压电片内圈直径：\nOPD=OPD/1000 !压电片外圈直径：\nEW= EW/1000 !宽度：\nET=ET/1000 !厚度：\nEH=EH/1000 !台阶高：\n\n/PREP7 \n!定义单元和材料属性\nET,1,SOLID185   \nMPTEMP,,,,,,,,  \nMPTEMP,1,0  \nMPDATA,DENS,1,,8290\nMPTEMP,,,,,,,,  \nMPTEMP,1,0  \nMPDATA,EX,1,,1.06E+011   \nMPDATA,PRXY,1,,0.35 \n\nET,2,SOLID5 \nMPTEMP,,,,,,,,  \nMPTEMP,1,0     \nMPDATA,DENS,2,,7750   \nMPTEMP,,,,,,,,  \nMPTEMP,1,0  \nMPDATA,PERX,2,,919E-009\nMPDATA,PERY,2,,919E-009   \nMPDATA,PERZ,2,,826E-009\nTB,PIEZ,2,,,0   \nTBMODIF,1,1,0   \nTBMODIF,1,2,0   \nTBMODIF,1,3,-5.35   \nTBMODIF,2,1,0   \nTBMODIF,2,2,0   \nTBMODIF,2,3,-5.35   \nTBMODIF,3,1,0   \nTBMODIF,3,2,0   \nTBMODIF,3,3,15.78   \nTBMODIF,4,1,0   \nTBMODIF,4,2,0   \nTBMODIF,4,3,0   \nTBMODIF,5,1,0   \nTBMODIF,5,2,12.3\nTBMODIF,5,3,0   \nTBMODIF,6,1,12.3\nTBMODIF,6,2,0   \nTBMODIF,6,3,0   \nTB,ANEL,2,1,21,0\nTBTEMP,0\nTBDATA,,1.2035E+011,7.52E+010,7.51E+010,0,0,0   \nTBDATA,,1.204E+011,7.51E+010,0,0,0,1.109E+011   \nTBDATA,,0,0,0,2.26E+010,0,0 \nTBDATA,,2.12E+010,0,2.11E+010,,,\n\n!超声波电机模型建立\nK,1,OAD/2,,,\nK,2,ITD/2,,,\nK,3,ITD/2,-EH,,!最上面\nK,4,OTD/2,-EH,,\nK,5,OTD/2,-EH+TT-TH,,\nK,6,ITD/2,-EH+TT-TH,,\nK,7,ITD/2,ET,,\nK,8,OAD/2,ET,,\nK,11,ITD/2,-EH-PT,,!最下面\nK,12,OTD/2,-EH-PT,,\nK,13,OTD/2,-EH+TT,,\nK,14,ITD/2,-EH+TT,,\nK,15,IAD/2,ET,,\nK,16,IAD/2,0,,\nK,17,IAD/2,-AT+ET,,\nK,18,OAD/2,-AT+ET,,\n\nK,100,0,0,0,\nK,101,0,0.003,0,\n\nLSTR,1,2\nLSTR,2,3\nLSTR,3,4\nLSTR,4,5\nLSTR,5,6\nLSTR,6,7\nLSTR,7,8\nLSTR,8,1\nLSTR,3,11\nLSTR,11,12\nLSTR,12,4\nLSTR,5,13\nLSTR,13,14\nLSTR,14,6\nLSTR,2,7\nLSTR,8,15\nLSTR,15,16\nLSTR,1,16\nLSTR,16,17\nLSTR,17,18\nLSTR,1,18\n\nAL,1,15,7,8\nAL,15,2,3,4,5,6,\nAL,9,10,11,3\nAL,5,12,13,14\nAL,8,16,17,18\nAL,18,19,20,21\n\nVROTAT,1,2,3,4, , ,100,101 ,360/FK, , !!!!!\nVROTAT,5,6, , , , ,100,101 ,360/FK, , !!!!!\nBLC4,0,TT-EH,OTD,-TH,TW !建立长方体\nVGEN, ,7, , , , ,-TW/2, , ,1!复制创建体  \nVOVLAP,4,7 !布尔操作\nVDELE,10, , ,1!删除体\nVSYMM,Z,8, , , ,0,0 !体镜像 \n\n!建立齿槽\nCSYS,5  \nWPSTYLE,,,,,,,,0\nVGEN,NZ/FK+1,4, , , ,360/NZ, , ,0  \nVGEN,NZ/FK+1,8, , , ,360/NZ, , ,0  \nVOVLAP,ALL\n*DO,I,1,NZ/FK+1\nCSYS,0\nVSEL,S,LOC,Y,TT-EH-TH/1.5,1\nCSYS,5\nVSEL,R,LOC,Y,(I-1)*360/NZ-TW/2/3.1415/ITD*360,TW/2/3.1415/ITD*360+(I-1)*360/NZ!选择体\nVDELE,ALL, , ,1\nALLSEL,ALL \n*ENDDO\n\n!旋转成体\nEPLOT \nCSYS,5 \nVGEN,FK,ALL, , , ,360/FK, , ,0 \n\n!Glue体\nVGLUE,ALL\n\n!添加材料属性\nALLSEL,ALL\nCSYS,0\nVSEL,S,LOC,Y,0,TT-EH\nVATT,       1, ,   1,       0   \nCSYS,5\nVSEL,S,LOC,X,0,OAD/2\nVATT,       1, ,   1,       0 \n\nALLSEL,ALL\nCSYS,0\nVSEL,R,LOC,Y,-EH-PT,-EH\nVATT,       2, ,  2,       0  \nALLSEL,ALL\n\n!网格体\nCSYS,0\nVSEL,R,LOC,Y,-EH-PT,-EH\nVSWEEP,ALL\n\nCSYS,0\nALLSEL,ALL \nVSEL,S,MAT,,1\nSMRT,6  \nSMRT,5  \nSMRT,4  \nMSHAPE,1,3d\nMSHKEY,0\nVMESH,ALL\n\nALLSEL,ALL\n\n!模态分析 \n/SOL  \nANTYPE,2\nMODOPT,LANB,22  \nEQSLV,SPAR  \nMXPAND,0, , ,0  \nLUMPM,0 \nPSTRES,0\nMODOPT,LANB,22,0,80000, ,OFF\n\nCSYS,5\nASEL,S,LOC,X,-IAD/2,IAD/2   \nDA,ALL,ALL,\nALLSEL,ALL\n\n!OUTPR,BASIC,ALL,  \n!OUTRES,ALL,ALL,\n \n/STATUS,SOLU\nSOLVE   \nFINISH\nCSYS,0\nALLSEL,ALL\n\n/POST1  \nSET,FIRST   \n/EFACET,1   \nPLNSOL, U,SUM, 2,1.0 !无轮廓2变0\n/post1\n*do,i,8,22\nset,1,i\n/VIEW,1,1,2,3   \n/ANG,1  \n/REP,FAST  \n/show,jpeg,,\nplnsol,u,sum,0,1.0\n/show,close\n*enddo\nFINISH\n\n!振幅仿真\n/SOL\nANTYPE,3\nHROPT,FULL  \nHROUT,ON\nLUMPM,0 \nEQSLV, ,0,  \nPSTRES,0\n\n!阻尼特性\nALPHAD,0,   \nBETAD,0,\nDMPSTR,0.005,   \n\n!压电耦合\n*do,i,1,(BS-1)\nALLSEL,ALL\ncsys,5\nnsel,S,LOC,X,ITD/2,OTD/2\ncsys,0\nnsel,R,loc,y,-eh-eq-pt\ncsys,5\nangle=360/BS\nnsel,r,loc,y,(i-1)*angle/2,i*angle/2\nb=1/2*(1-(-1)**i)*1\nc=1/2*(1-(-1)**(i+1))*1\nD,All,VOLT,b,c\n*enddo\n\nALLSEL,ALL\ncsys,5\nnsel,S,LOC,X,ITD/2,OTD/2\ncsys,0\nnsel,R,loc,y,-eh-eq-pt\ncsys,5\nangle=360/BS\nnsel,r,loc,y,(BS-1)*angle/2,((BS-1)*angle/2+3*angle/8)\nD,All,VOLT,(1/2*(1-(-1)**BS)*1),(1/2*(1-(-1)**(BS+1))*1)\n\nALLSEL,ALL\ncsys,5\nnsel,S,LOC,X,ITD/2,OTD/2\ncsys,0\nnsel,R,loc,y,-eh-eq-pt\ncsys,5\nangle=360/BS\nnsel,r,loc,y,((BS-1)*angle/2+3*angle/8),((BS-1)*angle/2+3*angle/4)\nD,All,VOLT,(1/2*(1-(-1)**(BS+1))*1),(1/2*(1-(-1)**(BS+2))*1)\n\n*do,i,1,(BS-1)\nALLSEL,ALL\ncsys,5\nnsel,S,LOC,X,ITD/2,OTD/2\ncsys,0\nnsel,R,loc,y,-eh-eq-pt\ncsys,5\nangle=360/BS\nnsel,r,loc,y,((BS-1)*angle/2+3*angle/4+(i-1)*angle/2),((BS-1)*angle/2+3*angle/4+(i)*angle/2)\ne=1/2*(1-(-1)**(BS+1+i))*1\nf=1/2*(1-(-1)**(BS+2+i))*1\nD,All,VOLT,e,f\n*enddo\n\nALLSEL,ALL\ncsys,5\nnsel,S,LOC,X,ITD/2,OTD/2\ncsys,0\nnsel,r,loc,y,-eh-eq\nD,All,VOLT,0,0\nALLSEL,ALL \n\nHARFRQ,26000,76000, \nNSUBST,5,  \nKBC,1\n/STATUS,SOLU\nSOLVE\n\n!选最大位移点\n/POST1\nNSORT,U,SUM,0,1, ,SELECT  \nPRNSOL,U,Z\n*get,node,SORT,0,IMAX\n\n!结果显示,打开后处理器\n/POST26 \nFILE,'finaltest','rst','.'   \n/UI,COLL,1  \nNUMVAR,200  \nSOLU,191,NCMIT  \nSTORE,MERGE \nPLCPLX,0\nPRCPLX,1\nFILLDATA,191,,,,1,1 \nREALVAR,191,191 \n\n!z方向位移 \nNSOL,2,node,U,Z, UZ_2, \nSTORE,MERGE \n\n!保存为txt(excel也行)\n/post26\n! Save time history variables to file zmovement.prn\n*CREATE,scratch,gui \n*DEL,_P26_EXPORT\n*DIM,_P26_EXPORT,TABLE,5,2 \nVGET,_P26_EXPORT(1,0),1 \nVGET,_P26_EXPORT(1,1),2,,0  \nVGET,_P26_EXPORT(1,2),2,,1  \n/OUTPUT,'zmovement','prn','.'  \n*VWRITE,'FREQ','UZ_2',' '   \n%14C %14C %14C\n*VWRITE,' ','REAL','IMAGINARY'  \n%14C %14C %14C  \n*VWRITE,_P26_EXPORT(1,0),_P26_EXPORT(1,1),_P26_EXPORT(1,2)  \n%14.5G %14.5G %14.5G\n/OUTPUT,TERM\n*END\n/INPUT,scratch,gui  \n! End of time history save  \n\n!x方向位移 \nNSOL,3,node,U,X, UX_3, \nSTORE,MERGE \n\n!保存为txt(excel也行)\n/post26\n! Save time history variables to file xmovement.prn\n*CREATE,scratch,gui \n*DEL,_P26_EXPORT\n*DIM,_P26_EXPORT,TABLE,5,2 \nVGET,_P26_EXPORT(1,0),1 \nVGET,_P26_EXPORT(1,1),3,,0  \nVGET,_P26_EXPORT(1,2),3,,1  \n/OUTPUT,'xmovement','prn','.'  \n*VWRITE,'FREQ','UX_3',' '   \n%14C %14C %14C  \n*VWRITE,' ','REAL','IMAGINARY'  \n%14C %14C %14C  \n*VWRITE,_P26_EXPORT(1,0),_P26_EXPORT(1,1),_P26_EXPORT(1,2)  \n%14.5G %14.5G %14.5G\n/OUTPUT,TERM\n*END\n/INPUT,scratch,gui  \n! End of time history save\n\n!y方向位移 \nNSOL,4,node,U,Y, UY_4, \nSTORE,MERGE \n\n!保存为txt(excel也行)\n/post26\n! Save time history variables to file ymovement.prn\n*CREATE,scratch,gui \n*DEL,_P26_EXPORT\n*DIM,_P26_EXPORT,TABLE,5,2 \nVGET,_P26_EXPORT(1,0),1 \nVGET,_P26_EXPORT(1,1),4,,0  \nVGET,_P26_EXPORT(1,2),4,,1  \n/OUTPUT,'ymovement','prn','.'  \n*VWRITE,'FREQ','UY_4',' '   \n%14C %14C %14C  \n*VWRITE,' ','REAL','IMAGINARY'  \n%14C %14C %14C  \n*VWRITE,_P26_EXPORT(1,0),_P26_EXPORT(1,1),_P26_EXPORT(1,2)  \n%14.5G %14.5G %14.5G\n/OUTPUT,TERM\n*END\n/INPUT,scratch,gui  \n! End of time history save\n\n!选择电流点\nRFORCE,2,180,AMPS,, AMPS_2  \nSTORE,MERGE \nFILLDATA,192,,,,0,0 \nFILLDATA,193,,,,1,0 \nFILLDATA,194,,,,-1,0\nFILLDATA,195,,,,1,1 \nVARNAME,195,NSET\n! Name: Z   \n! ID:  3\n! Function: 1/{AMPS_2}  \nFILLDATA,199,,,,1,0 \nREALVAR,199,199 \nQUOT,3,199,2,,Z \nSTORE,MERGE \n\n!保存为txt(excel也行)\n/post26\n! Save time history variables to file current.prn   \n*CREATE,scratch,gui \n*DEL,_P26_EXPORT\n*DIM,_P26_EXPORT,TABLE,5,2 \nVGET,_P26_EXPORT(1,0),1 \nVGET,_P26_EXPORT(1,1),3,,0  \nVGET,_P26_EXPORT(1,2),3,,1  \n/OUTPUT,'current','prn','.' \n*VWRITE,'FREQ','Z',' '  \n%14C %14C %14C  \n*VWRITE,' ','REAL','IMAGINARY'  \n%14C %14C %14C  \n*VWRITE,_P26_EXPORT(1,0),_P26_EXPORT(1,1),_P26_EXPORT(1,2)  \n%14.5G %14.5G %14.5G\n/OUTPUT,TERM\n*END\n/INPUT,scratch,gui  \n! End of time history save " ("字符串")) -> (w891:string)
        n134 = Write to Text File(file (use dialog)=w892, text=w891) -> ()  [unwired: 2 in, 3 out]
      }
      event "9": Value Change {
        n135 = event-data() -> ()  [unwired: 1 in, 6 out]
        n136 = Number To Fractional String(number="轴内圈直径") -> (F-format string=w895:string)  [unwired: 3 in]
        n137 = Open/Create/Replace File(file path (use dialog)=path "H:/新/finaltest.dat" ("文件路径（使用对话框）"), operation (0:open)=T1."replace" ("操作(0:open)")) -> (refnum out=w900:refnum<file>)  [unwired: 4 in, 2 out]
        n138 = Concatenate Strings("/RGB,INDEX,100,100,100, 0   \n/RGB,INDEX, 80, 80, 80,13   \n/RGB,INDEX, 60, 60, 60,14   \n/RGB,INDEX, 0, 0, 0,15  \n\n/REPLOT,RESIZE  \n/CLEAR,NOSTART \nNZ=25 !齿数：\nTH=1.5 !平均齿高：\nWTH=1.5 !外侧斜齿高\nNTH=1.5 !内侧斜齿高\nWDTH=0.0 !齿外侧导角高度\nWDTL=0.0 !齿外侧导水平长度\nNDTH=0.0 !齿内侧导角高度\nNDTL=0.0 !齿内侧导水平长度\nTT=2 !齿厚：\nTW=0.1 !齿槽宽：\nITD=8 !定子齿内圈直径：\nOTD=13.3 !定子齿外圈直径：\nIAD=" ("字符串"), w895, " !轴内圈直径：\nOAD=6 !轴外圈直径：\nAT=1.6 !轴厚度\nPT=0.4 !压电片厚：\nIPD=8 !压电片内圈直径：\nOPD=13.3 !压电片外圈直径：\nEW= ITD-OAD !宽度：\nET=0.2 !厚度：\nEH=0.2 !台阶高：\nBS=4 !波数\nFK=5 !定子分块建模分块数与齿数成整数倍的关系 \n\nNZ=NZ !齿数：\nTH=TH/1000 !齿高：\nWTH=WTH/1000 !外侧斜齿高\nNTH=NTH/1000 !内侧斜齿高\nWDTH=WDTH/1000 !齿外侧导角高度\nWDTL=WDTL/1000 !齿外侧导水平长度\nNDTH=NDTH/1000 !齿内侧导角高度\nNDTL=NDTL/1000 !齿内侧导水平长度\nTT=TT/1000 !齿厚：\nTW=TW/1000 !齿槽宽：\nITD=ITD/1000 !定子齿内圈直径：\nOTD=OTD/1000 !定子齿外圈直径：\nIAD=IAD/1000 !轴内圈直径：\nOAD=OAD/1000 !轴外圈直径：\nAT=AT/1000 !轴厚度\nPT=PT/1000 !压电片厚：\nIPD=IPD/1000 !压电片内圈直径：\nOPD=OPD/1000 !压电片外圈直径：\nEW= EW/1000 !宽度：\nET=ET/1000 !厚度：\nEH=EH/1000 !台阶高：\n\n/PREP7 \n!定义单元和材料属性\nET,1,SOLID185   \nMPTEMP,,,,,,,,  \nMPTEMP,1,0  \nMPDATA,DENS,1,,8290\nMPTEMP,,,,,,,,  \nMPTEMP,1,0  \nMPDATA,EX,1,,1.06E+011   \nMPDATA,PRXY,1,,0.35 \n\nET,2,SOLID5 \nMPTEMP,,,,,,,,  \nMPTEMP,1,0     \nMPDATA,DENS,2,,7750   \nMPTEMP,,,,,,,,  \nMPTEMP,1,0  \nMPDATA,PERX,2,,919E-009\nMPDATA,PERY,2,,919E-009   \nMPDATA,PERZ,2,,826E-009\nTB,PIEZ,2,,,0   \nTBMODIF,1,1,0   \nTBMODIF,1,2,0   \nTBMODIF,1,3,-5.35   \nTBMODIF,2,1,0   \nTBMODIF,2,2,0   \nTBMODIF,2,3,-5.35   \nTBMODIF,3,1,0   \nTBMODIF,3,2,0   \nTBMODIF,3,3,15.78   \nTBMODIF,4,1,0   \nTBMODIF,4,2,0   \nTBMODIF,4,3,0   \nTBMODIF,5,1,0   \nTBMODIF,5,2,12.3\nTBMODIF,5,3,0   \nTBMODIF,6,1,12.3\nTBMODIF,6,2,0   \nTBMODIF,6,3,0   \nTB,ANEL,2,1,21,0\nTBTEMP,0\nTBDATA,,1.2035E+011,7.52E+010,7.51E+010,0,0,0   \nTBDATA,,1.204E+011,7.51E+010,0,0,0,1.109E+011   \nTBDATA,,0,0,0,2.26E+010,0,0 \nTBDATA,,2.12E+010,0,2.11E+010,,,\n\n!超声波电机模型建立\nK,1,OAD/2,,,\nK,2,ITD/2,,,\nK,3,ITD/2,-EH,,!最上面\nK,4,OTD/2,-EH,,\nK,5,OTD/2,-EH+TT-TH,,\nK,6,ITD/2,-EH+TT-TH,,\nK,7,ITD/2,ET,,\nK,8,OAD/2,ET,,\nK,11,ITD/2,-EH-PT,,!最下面\nK,12,OTD/2,-EH-PT,,\nK,13,OTD/2,-EH+TT,,\nK,14,ITD/2,-EH+TT,,\nK,15,IAD/2,ET,,\nK,16,IAD/2,0,,\nK,17,IAD/2,-AT+ET,,\nK,18,OAD/2,-AT+ET,,\n\nK,100,0,0,0,\nK,101,0,0.003,0,\n\nLSTR,1,2\nLSTR,2,3\nLSTR,3,4\nLSTR,4,5\nLSTR,5,6\nLSTR,6,7\nLSTR,7,8\nLSTR,8,1\nLSTR,3,11\nLSTR,11,12\nLSTR,12,4\nLSTR,5,13\nLSTR,13,14\nLSTR,14,6\nLSTR,2,7\nLSTR,8,15\nLSTR,15,16\nLSTR,1,16\nLSTR,16,17\nLSTR,17,18\nLSTR,1,18\n\nAL,1,15,7,8\nAL,15,2,3,4,5,6,\nAL,9,10,11,3\nAL,5,12,13,14\nAL,8,16,17,18\nAL,18,19,20,21\n\nVROTAT,1,2,3,4, , ,100,101 ,360/FK, , !!!!!\nVROTAT,5,6, , , , ,100,101 ,360/FK, , !!!!!\nBLC4,0,TT-EH,OTD,-TH,TW !建立长方体\nVGEN, ,7, , , , ,-TW/2, , ,1!复制创建体  \nVOVLAP,4,7 !布尔操作\nVDELE,10, , ,1!删除体\nVSYMM,Z,8, , , ,0,0 !体镜像 \n\n!建立齿槽\nCSYS,5  \nWPSTYLE,,,,,,,,0\nVGEN,NZ/FK+1,4, , , ,360/NZ, , ,0  \nVGEN,NZ/FK+1,8, , , ,360/NZ, , ,0  \nVOVLAP,ALL\n*DO,I,1,NZ/FK+1\nCSYS,0\nVSEL,S,LOC,Y,TT-EH-TH/1.5,1\nCSYS,5\nVSEL,R,LOC,Y,(I-1)*360/NZ-TW/2/3.1415/ITD*360,TW/2/3.1415/ITD*360+(I-1)*360/NZ!选择体\nVDELE,ALL, , ,1\nALLSEL,ALL \n*ENDDO\n\n!旋转成体\nEPLOT \nCSYS,5 \nVGEN,FK,ALL, , , ,360/FK, , ,0 \n\n!Glue体\nVGLUE,ALL\n\n!添加材料属性\nALLSEL,ALL\nCSYS,0\nVSEL,S,LOC,Y,0,TT-EH\nVATT,       1, ,   1,       0   \nCSYS,5\nVSEL,S,LOC,X,0,OAD/2\nVATT,       1, ,   1,       0 \n\nALLSEL,ALL\nCSYS,0\nVSEL,R,LOC,Y,-EH-PT,-EH\nVATT,       2, ,  2,       0  \nALLSEL,ALL\n\n!网格体\nCSYS,0\nVSEL,R,LOC,Y,-EH-PT,-EH\nVSWEEP,ALL\n\nCSYS,0\nALLSEL,ALL \nVSEL,S,MAT,,1\nSMRT,6  \nSMRT,5  \nSMRT,4  \nMSHAPE,1,3d\nMSHKEY,0\nVMESH,ALL\n\nALLSEL,ALL\n\n!模态分析 \n/SOL  \nANTYPE,2\nMODOPT,LANB,22  \nEQSLV,SPAR  \nMXPAND,0, , ,0  \nLUMPM,0 \nPSTRES,0\nMODOPT,LANB,22,0,80000, ,OFF\n\nCSYS,5\nASEL,S,LOC,X,-IAD/2,IAD/2   \nDA,ALL,ALL,\nALLSEL,ALL\n\n!OUTPR,BASIC,ALL,  \n!OUTRES,ALL,ALL,\n \n/STATUS,SOLU\nSOLVE   \nFINISH\nCSYS,0\nALLSEL,ALL\n\n/POST1  \nSET,FIRST   \n/EFACET,1   \nPLNSOL, U,SUM, 2,1.0 !无轮廓2变0\n/post1\n*do,i,8,22\nset,1,i\n/VIEW,1,1,2,3   \n/ANG,1  \n/REP,FAST  \n/show,jpeg,,\nplnsol,u,sum,0,1.0\n/show,close\n*enddo\nFINISH\n\n!振幅仿真\n/SOL\nANTYPE,3\nHROPT,FULL  \nHROUT,ON\nLUMPM,0 \nEQSLV, ,0,  \nPSTRES,0\n\n!阻尼特性\nALPHAD,0,   \nBETAD,0,\nDMPSTR,0.005,   \n\n!压电耦合\n*do,i,1,(BS-1)\nALLSEL,ALL\ncsys,5\nnsel,S,LOC,X,ITD/2,OTD/2\ncsys,0\nnsel,R,loc,y,-eh-eq-pt\ncsys,5\nangle=360/BS\nnsel,r,loc,y,(i-1)*angle/2,i*angle/2\nb=1/2*(1-(-1)**i)*1\nc=1/2*(1-(-1)**(i+1))*1\nD,All,VOLT,b,c\n*enddo\n\nALLSEL,ALL\ncsys,5\nnsel,S,LOC,X,ITD/2,OTD/2\ncsys,0\nnsel,R,loc,y,-eh-eq-pt\ncsys,5\nangle=360/BS\nnsel,r,loc,y,(BS-1)*angle/2,((BS-1)*angle/2+3*angle/8)\nD,All,VOLT,(1/2*(1-(-1)**BS)*1),(1/2*(1-(-1)**(BS+1))*1)\n\nALLSEL,ALL\ncsys,5\nnsel,S,LOC,X,ITD/2,OTD/2\ncsys,0\nnsel,R,loc,y,-eh-eq-pt\ncsys,5\nangle=360/BS\nnsel,r,loc,y,((BS-1)*angle/2+3*angle/8),((BS-1)*angle/2+3*angle/4)\nD,All,VOLT,(1/2*(1-(-1)**(BS+1))*1),(1/2*(1-(-1)**(BS+2))*1)\n\n*do,i,1,(BS-1)\nALLSEL,ALL\ncsys,5\nnsel,S,LOC,X,ITD/2,OTD/2\ncsys,0\nnsel,R,loc,y,-eh-eq-pt\ncsys,5\nangle=360/BS\nnsel,r,loc,y,((BS-1)*angle/2+3*angle/4+(i-1)*angle/2),((BS-1)*angle/2+3*angle/4+(i)*angle/2)\ne=1/2*(1-(-1)**(BS+1+i))*1\nf=1/2*(1-(-1)**(BS+2+i))*1\nD,All,VOLT,e,f\n*enddo\n\nALLSEL,ALL\ncsys,5\nnsel,S,LOC,X,ITD/2,OTD/2\ncsys,0\nnsel,r,loc,y,-eh-eq\nD,All,VOLT,0,0\nALLSEL,ALL \n\nHARFRQ,26000,76000, \nNSUBST,5,  \nKBC,1\n/STATUS,SOLU\nSOLVE\n\n!选最大位移点\n/POST1\nNSORT,U,SUM,0,1, ,SELECT  \nPRNSOL,U,Z\n*get,node,SORT,0,IMAX\n\n!结果显示,打开后处理器\n/POST26 \nFILE,'finaltest','rst','.'   \n/UI,COLL,1  \nNUMVAR,200  \nSOLU,191,NCMIT  \nSTORE,MERGE \nPLCPLX,0\nPRCPLX,1\nFILLDATA,191,,,,1,1 \nREALVAR,191,191 \n\n!z方向位移 \nNSOL,2,node,U,Z, UZ_2, \nSTORE,MERGE \n\n!保存为txt(excel也行)\n/post26\n! Save time history variables to file zmovement.prn\n*CREATE,scratch,gui \n*DEL,_P26_EXPORT\n*DIM,_P26_EXPORT,TABLE,5,2 \nVGET,_P26_EXPORT(1,0),1 \nVGET,_P26_EXPORT(1,1),2,,0  \nVGET,_P26_EXPORT(1,2),2,,1  \n/OUTPUT,'zmovement','prn','.'  \n*VWRITE,'FREQ','UZ_2',' '   \n%14C %14C %14C\n*VWRITE,' ','REAL','IMAGINARY'  \n%14C %14C %14C  \n*VWRITE,_P26_EXPORT(1,0),_P26_EXPORT(1,1),_P26_EXPORT(1,2)  \n%14.5G %14.5G %14.5G\n/OUTPUT,TERM\n*END\n/INPUT,scratch,gui  \n! End of time history save  \n\n!x方向位移 \nNSOL,3,node,U,X, UX_3, \nSTORE,MERGE \n\n!保存为txt(excel也行)\n/post26\n! Save time history variables to file xmovement.prn\n*CREATE,scratch,gui \n*DEL,_P26_EXPORT\n*DIM,_P26_EXPORT,TABLE,5,2 \nVGET,_P26_EXPORT(1,0),1 \nVGET,_P26_EXPORT(1,1),3,,0  \nVGET,_P26_EXPORT(1,2),3,,1  \n/OUTPUT,'xmovement','prn','.'  \n*VWRITE,'FREQ','UX_3',' '   \n%14C %14C %14C  \n*VWRITE,' ','REAL','IMAGINARY'  \n%14C %14C %14C  \n*VWRITE,_P26_EXPORT(1,0),_P26_EXPORT(1,1),_P26_EXPORT(1,2)  \n%14.5G %14.5G %14.5G\n/OUTPUT,TERM\n*END\n/INPUT,scratch,gui  \n! End of time history save\n\n!y方向位移 \nNSOL,4,node,U,Y, UY_4, \nSTORE,MERGE \n\n!保存为txt(excel也行)\n/post26\n! Save time history variables to file ymovement.prn\n*CREATE,scratch,gui \n*DEL,_P26_EXPORT\n*DIM,_P26_EXPORT,TABLE,5,2 \nVGET,_P26_EXPORT(1,0),1 \nVGET,_P26_EXPORT(1,1),4,,0  \nVGET,_P26_EXPORT(1,2),4,,1  \n/OUTPUT,'ymovement','prn','.'  \n*VWRITE,'FREQ','UY_4',' '   \n%14C %14C %14C  \n*VWRITE,' ','REAL','IMAGINARY'  \n%14C %14C %14C  \n*VWRITE,_P26_EXPORT(1,0),_P26_EXPORT(1,1),_P26_EXPORT(1,2)  \n%14.5G %14.5G %14.5G\n/OUTPUT,TERM\n*END\n/INPUT,scratch,gui  \n! End of time history save\n\n!选择电流点\nRFORCE,2,180,AMPS,, AMPS_2  \nSTORE,MERGE \nFILLDATA,192,,,,0,0 \nFILLDATA,193,,,,1,0 \nFILLDATA,194,,,,-1,0\nFILLDATA,195,,,,1,1 \nVARNAME,195,NSET\n! Name: Z   \n! ID:  3\n! Function: 1/{AMPS_2}  \nFILLDATA,199,,,,1,0 \nREALVAR,199,199 \nQUOT,3,199,2,,Z \nSTORE,MERGE \n\n!保存为txt(excel也行)\n/post26\n! Save time history variables to file current.prn   \n*CREATE,scratch,gui \n*DEL,_P26_EXPORT\n*DIM,_P26_EXPORT,TABLE,5,2 \nVGET,_P26_EXPORT(1,0),1 \nVGET,_P26_EXPORT(1,1),3,,0  \nVGET,_P26_EXPORT(1,2),3,,1  \n/OUTPUT,'current','prn','.' \n*VWRITE,'FREQ','Z',' '  \n%14C %14C %14C  \n*VWRITE,' ','REAL','IMAGINARY'  \n%14C %14C %14C  \n*VWRITE,_P26_EXPORT(1,0),_P26_EXPORT(1,1),_P26_EXPORT(1,2)  \n%14.5G %14.5G %14.5G\n/OUTPUT,TERM\n*END\n/INPUT,scratch,gui  \n! End of time history save " ("字符串")) -> (w899:string)
        n139 = Write to Text File(file (use dialog)=w900, text=w899) -> ()  [unwired: 2 in, 3 out]
      }
      event "10": Value Change {
        n140 = event-data() -> ()  [unwired: 1 in, 6 out]
        n141 = Number To Fractional String(number="轴外圈直径") -> (F-format string=w903:string)  [unwired: 3 in]
        n142 = Open/Create/Replace File(file path (use dialog)=path "H:/新/finaltest.dat" ("文件路径（使用对话框）"), operation (0:open)=T1."replace" ("操作(0:open)")) -> (refnum out=w908:refnum<file>)  [unwired: 4 in, 2 out]
        n143 = Concatenate Strings("/RGB,INDEX,100,100,100, 0   \n/RGB,INDEX, 80, 80, 80,13   \n/RGB,INDEX, 60, 60, 60,14   \n/RGB,INDEX, 0, 0, 0,15  \n\n/REPLOT,RESIZE  \n/CLEAR,NOSTART \nNZ=25 !齿数：\nTH=1.5 !平均齿高：\nWTH=1.5 !外侧斜齿高\nNTH=1.5 !内侧斜齿高\nWDTH=0.0 !齿外侧导角高度\nWDTL=0.0 !齿外侧导水平长度\nNDTH=0.0 !齿内侧导角高度\nNDTL=0.0 !齿内侧导水平长度\nTT=2 !齿厚：\nTW=0.1 !齿槽宽：\nITD=8 !定子齿内圈直径：\nOTD=13.3 !定子齿外圈直径：\nIAD=2.1 !轴内圈直径：\nOAD=" ("字符串"), w903, " !轴外圈直径：\nAT=1.6 !轴厚度\nPT=0.4 !压电片厚：\nIPD=8 !压电片内圈直径：\nOPD=13.3 !压电片外圈直径：\nEW= ITD-OAD !宽度：\nET=0.2 !厚度：\nEH=0.2 !台阶高：\nBS=4 !波数\nFK=5 !定子分块建模分块数与齿数成整数倍的关系 \n\nNZ=NZ !齿数：\nTH=TH/1000 !齿高：\nWTH=WTH/1000 !外侧斜齿高\nNTH=NTH/1000 !内侧斜齿高\nWDTH=WDTH/1000 !齿外侧导角高度\nWDTL=WDTL/1000 !齿外侧导水平长度\nNDTH=NDTH/1000 !齿内侧导角高度\nNDTL=NDTL/1000 !齿内侧导水平长度\nTT=TT/1000 !齿厚：\nTW=TW/1000 !齿槽宽：\nITD=ITD/1000 !定子齿内圈直径：\nOTD=OTD/1000 !定子齿外圈直径：\nIAD=IAD/1000 !轴内圈直径：\nOAD=OAD/1000 !轴外圈直径：\nAT=AT/1000 !轴厚度\nPT=PT/1000 !压电片厚：\nIPD=IPD/1000 !压电片内圈直径：\nOPD=OPD/1000 !压电片外圈直径：\nEW= EW/1000 !宽度：\nET=ET/1000 !厚度：\nEH=EH/1000 !台阶高：\n\n/PREP7 \n!定义单元和材料属性\nET,1,SOLID185   \nMPTEMP,,,,,,,,  \nMPTEMP,1,0  \nMPDATA,DENS,1,,8290\nMPTEMP,,,,,,,,  \nMPTEMP,1,0  \nMPDATA,EX,1,,1.06E+011   \nMPDATA,PRXY,1,,0.35 \n\nET,2,SOLID5 \nMPTEMP,,,,,,,,  \nMPTEMP,1,0     \nMPDATA,DENS,2,,7750   \nMPTEMP,,,,,,,,  \nMPTEMP,1,0  \nMPDATA,PERX,2,,919E-009\nMPDATA,PERY,2,,919E-009   \nMPDATA,PERZ,2,,826E-009\nTB,PIEZ,2,,,0   \nTBMODIF,1,1,0   \nTBMODIF,1,2,0   \nTBMODIF,1,3,-5.35   \nTBMODIF,2,1,0   \nTBMODIF,2,2,0   \nTBMODIF,2,3,-5.35   \nTBMODIF,3,1,0   \nTBMODIF,3,2,0   \nTBMODIF,3,3,15.78   \nTBMODIF,4,1,0   \nTBMODIF,4,2,0   \nTBMODIF,4,3,0   \nTBMODIF,5,1,0   \nTBMODIF,5,2,12.3\nTBMODIF,5,3,0   \nTBMODIF,6,1,12.3\nTBMODIF,6,2,0   \nTBMODIF,6,3,0   \nTB,ANEL,2,1,21,0\nTBTEMP,0\nTBDATA,,1.2035E+011,7.52E+010,7.51E+010,0,0,0   \nTBDATA,,1.204E+011,7.51E+010,0,0,0,1.109E+011   \nTBDATA,,0,0,0,2.26E+010,0,0 \nTBDATA,,2.12E+010,0,2.11E+010,,,\n\n!超声波电机模型建立\nK,1,OAD/2,,,\nK,2,ITD/2,,,\nK,3,ITD/2,-EH,,!最上面\nK,4,OTD/2,-EH,,\nK,5,OTD/2,-EH+TT-TH,,\nK,6,ITD/2,-EH+TT-TH,,\nK,7,ITD/2,ET,,\nK,8,OAD/2,ET,,\nK,11,ITD/2,-EH-PT,,!最下面\nK,12,OTD/2,-EH-PT,,\nK,13,OTD/2,-EH+TT,,\nK,14,ITD/2,-EH+TT,,\nK,15,IAD/2,ET,,\nK,16,IAD/2,0,,\nK,17,IAD/2,-AT+ET,,\nK,18,OAD/2,-AT+ET,,\n\nK,100,0,0,0,\nK,101,0,0.003,0,\n\nLSTR,1,2\nLSTR,2,3\nLSTR,3,4\nLSTR,4,5\nLSTR,5,6\nLSTR,6,7\nLSTR,7,8\nLSTR,8,1\nLSTR,3,11\nLSTR,11,12\nLSTR,12,4\nLSTR,5,13\nLSTR,13,14\nLSTR,14,6\nLSTR,2,7\nLSTR,8,15\nLSTR,15,16\nLSTR,1,16\nLSTR,16,17\nLSTR,17,18\nLSTR,1,18\n\nAL,1,15,7,8\nAL,15,2,3,4,5,6,\nAL,9,10,11,3\nAL,5,12,13,14\nAL,8,16,17,18\nAL,18,19,20,21\n\nVROTAT,1,2,3,4, , ,100,101 ,360/FK, , !!!!!\nVROTAT,5,6, , , , ,100,101 ,360/FK, , !!!!!\nBLC4,0,TT-EH,OTD,-TH,TW !建立长方体\nVGEN, ,7, , , , ,-TW/2, , ,1!复制创建体  \nVOVLAP,4,7 !布尔操作\nVDELE,10, , ,1!删除体\nVSYMM,Z,8, , , ,0,0 !体镜像 \n\n!建立齿槽\nCSYS,5  \nWPSTYLE,,,,,,,,0\nVGEN,NZ/FK+1,4, , , ,360/NZ, , ,0  \nVGEN,NZ/FK+1,8, , , ,360/NZ, , ,0  \nVOVLAP,ALL\n*DO,I,1,NZ/FK+1\nCSYS,0\nVSEL,S,LOC,Y,TT-EH-TH/1.5,1\nCSYS,5\nVSEL,R,LOC,Y,(I-1)*360/NZ-TW/2/3.1415/ITD*360,TW/2/3.1415/ITD*360+(I-1)*360/NZ!选择体\nVDELE,ALL, , ,1\nALLSEL,ALL \n*ENDDO\n\n!旋转成体\nEPLOT \nCSYS,5 \nVGEN,FK,ALL, , , ,360/FK, , ,0 \n\n!Glue体\nVGLUE,ALL\n\n!添加材料属性\nALLSEL,ALL\nCSYS,0\nVSEL,S,LOC,Y,0,TT-EH\nVATT,       1, ,   1,       0   \nCSYS,5\nVSEL,S,LOC,X,0,OAD/2\nVATT,       1, ,   1,       0 \n\nALLSEL,ALL\nCSYS,0\nVSEL,R,LOC,Y,-EH-PT,-EH\nVATT,       2, ,  2,       0  \nALLSEL,ALL\n\n!网格体\nCSYS,0\nVSEL,R,LOC,Y,-EH-PT,-EH\nVSWEEP,ALL\n\nCSYS,0\nALLSEL,ALL \nVSEL,S,MAT,,1\nSMRT,6  \nSMRT,5  \nSMRT,4  \nMSHAPE,1,3d\nMSHKEY,0\nVMESH,ALL\n\nALLSEL,ALL\n\n!模态分析 \n/SOL  \nANTYPE,2\nMODOPT,LANB,22  \nEQSLV,SPAR  \nMXPAND,0, , ,0  \nLUMPM,0 \nPSTRES,0\nMODOPT,LANB,22,0,80000, ,OFF\n\nCSYS,5\nASEL,S,LOC,X,-IAD/2,IAD/2   \nDA,ALL,ALL,\nALLSEL,ALL\n\n!OUTPR,BASIC,ALL,  \n!OUTRES,ALL,ALL,\n \n/STATUS,SOLU\nSOLVE   \nFINISH\nCSYS,0\nALLSEL,ALL\n\n/POST1  \nSET,FIRST   \n/EFACET,1   \nPLNSOL, U,SUM, 2,1.0 !无轮廓2变0\n/post1\n*do,i,8,22\nset,1,i\n/VIEW,1,1,2,3   \n/ANG,1  \n/REP,FAST  \n/show,jpeg,,\nplnsol,u,sum,0,1.0\n/show,close\n*enddo\nFINISH\n\n!振幅仿真\n/SOL\nANTYPE,3\nHROPT,FULL  \nHROUT,ON\nLUMPM,0 \nEQSLV, ,0,  \nPSTRES,0\n\n!阻尼特性\nALPHAD,0,   \nBETAD,0,\nDMPSTR,0.005,   \n\n!压电耦合\n*do,i,1,(BS-1)\nALLSEL,ALL\ncsys,5\nnsel,S,LOC,X,ITD/2,OTD/2\ncsys,0\nnsel,R,loc,y,-eh-eq-pt\ncsys,5\nangle=360/BS\nnsel,r,loc,y,(i-1)*angle/2,i*angle/2\nb=1/2*(1-(-1)**i)*1\nc=1/2*(1-(-1)**(i+1))*1\nD,All,VOLT,b,c\n*enddo\n\nALLSEL,ALL\ncsys,5\nnsel,S,LOC,X,ITD/2,OTD/2\ncsys,0\nnsel,R,loc,y,-eh-eq-pt\ncsys,5\nangle=360/BS\nnsel,r,loc,y,(BS-1)*angle/2,((BS-1)*angle/2+3*angle/8)\nD,All,VOLT,(1/2*(1-(-1)**BS)*1),(1/2*(1-(-1)**(BS+1))*1)\n\nALLSEL,ALL\ncsys,5\nnsel,S,LOC,X,ITD/2,OTD/2\ncsys,0\nnsel,R,loc,y,-eh-eq-pt\ncsys,5\nangle=360/BS\nnsel,r,loc,y,((BS-1)*angle/2+3*angle/8),((BS-1)*angle/2+3*angle/4)\nD,All,VOLT,(1/2*(1-(-1)**(BS+1))*1),(1/2*(1-(-1)**(BS+2))*1)\n\n*do,i,1,(BS-1)\nALLSEL,ALL\ncsys,5\nnsel,S,LOC,X,ITD/2,OTD/2\ncsys,0\nnsel,R,loc,y,-eh-eq-pt\ncsys,5\nangle=360/BS\nnsel,r,loc,y,((BS-1)*angle/2+3*angle/4+(i-1)*angle/2),((BS-1)*angle/2+3*angle/4+(i)*angle/2)\ne=1/2*(1-(-1)**(BS+1+i))*1\nf=1/2*(1-(-1)**(BS+2+i))*1\nD,All,VOLT,e,f\n*enddo\n\nALLSEL,ALL\ncsys,5\nnsel,S,LOC,X,ITD/2,OTD/2\ncsys,0\nnsel,r,loc,y,-eh-eq\nD,All,VOLT,0,0\nALLSEL,ALL \n\nHARFRQ,26000,76000, \nNSUBST,5,  \nKBC,1\n/STATUS,SOLU\nSOLVE\n\n!选最大位移点\n/POST1\nNSORT,U,SUM,0,1, ,SELECT  \nPRNSOL,U,Z\n*get,node,SORT,0,IMAX\n\n!结果显示,打开后处理器\n/POST26 \nFILE,'finaltest','rst','.'   \n/UI,COLL,1  \nNUMVAR,200  \nSOLU,191,NCMIT  \nSTORE,MERGE \nPLCPLX,0\nPRCPLX,1\nFILLDATA,191,,,,1,1 \nREALVAR,191,191 \n\n!z方向位移 \nNSOL,2,node,U,Z, UZ_2, \nSTORE,MERGE \n\n!保存为txt(excel也行)\n/post26\n! Save time history variables to file zmovement.prn\n*CREATE,scratch,gui \n*DEL,_P26_EXPORT\n*DIM,_P26_EXPORT,TABLE,5,2 \nVGET,_P26_EXPORT(1,0),1 \nVGET,_P26_EXPORT(1,1),2,,0  \nVGET,_P26_EXPORT(1,2),2,,1  \n/OUTPUT,'zmovement','prn','.'  \n*VWRITE,'FREQ','UZ_2',' '   \n%14C %14C %14C\n*VWRITE,' ','REAL','IMAGINARY'  \n%14C %14C %14C  \n*VWRITE,_P26_EXPORT(1,0),_P26_EXPORT(1,1),_P26_EXPORT(1,2)  \n%14.5G %14.5G %14.5G\n/OUTPUT,TERM\n*END\n/INPUT,scratch,gui  \n! End of time history save  \n\n!x方向位移 \nNSOL,3,node,U,X, UX_3, \nSTORE,MERGE \n\n!保存为txt(excel也行)\n/post26\n! Save time history variables to file xmovement.prn\n*CREATE,scratch,gui \n*DEL,_P26_EXPORT\n*DIM,_P26_EXPORT,TABLE,5,2 \nVGET,_P26_EXPORT(1,0),1 \nVGET,_P26_EXPORT(1,1),3,,0  \nVGET,_P26_EXPORT(1,2),3,,1  \n/OUTPUT,'xmovement','prn','.'  \n*VWRITE,'FREQ','UX_3',' '   \n%14C %14C %14C  \n*VWRITE,' ','REAL','IMAGINARY'  \n%14C %14C %14C  \n*VWRITE,_P26_EXPORT(1,0),_P26_EXPORT(1,1),_P26_EXPORT(1,2)  \n%14.5G %14.5G %14.5G\n/OUTPUT,TERM\n*END\n/INPUT,scratch,gui  \n! End of time history save\n\n!y方向位移 \nNSOL,4,node,U,Y, UY_4, \nSTORE,MERGE \n\n!保存为txt(excel也行)\n/post26\n! Save time history variables to file ymovement.prn\n*CREATE,scratch,gui \n*DEL,_P26_EXPORT\n*DIM,_P26_EXPORT,TABLE,5,2 \nVGET,_P26_EXPORT(1,0),1 \nVGET,_P26_EXPORT(1,1),4,,0  \nVGET,_P26_EXPORT(1,2),4,,1  \n/OUTPUT,'ymovement','prn','.'  \n*VWRITE,'FREQ','UY_4',' '   \n%14C %14C %14C  \n*VWRITE,' ','REAL','IMAGINARY'  \n%14C %14C %14C  \n*VWRITE,_P26_EXPORT(1,0),_P26_EXPORT(1,1),_P26_EXPORT(1,2)  \n%14.5G %14.5G %14.5G\n/OUTPUT,TERM\n*END\n/INPUT,scratch,gui  \n! End of time history save\n\n!选择电流点\nRFORCE,2,180,AMPS,, AMPS_2  \nSTORE,MERGE \nFILLDATA,192,,,,0,0 \nFILLDATA,193,,,,1,0 \nFILLDATA,194,,,,-1,0\nFILLDATA,195,,,,1,1 \nVARNAME,195,NSET\n! Name: Z   \n! ID:  3\n! Function: 1/{AMPS_2}  \nFILLDATA,199,,,,1,0 \nREALVAR,199,199 \nQUOT,3,199,2,,Z \nSTORE,MERGE \n\n!保存为txt(excel也行)\n/post26\n! Save time history variables to file current.prn   \n*CREATE,scratch,gui \n*DEL,_P26_EXPORT\n*DIM,_P26_EXPORT,TABLE,5,2 \nVGET,_P26_EXPORT(1,0),1 \nVGET,_P26_EXPORT(1,1),3,,0  \nVGET,_P26_EXPORT(1,2),3,,1  \n/OUTPUT,'current','prn','.' \n*VWRITE,'FREQ','Z',' '  \n%14C %14C %14C  \n*VWRITE,' ','REAL','IMAGINARY'  \n%14C %14C %14C  \n*VWRITE,_P26_EXPORT(1,0),_P26_EXPORT(1,1),_P26_EXPORT(1,2)  \n%14.5G %14.5G %14.5G\n/OUTPUT,TERM\n*END\n/INPUT,scratch,gui  \n! End of time history save " ("字符串")) -> (w907:string)
        n144 = Write to Text File(file (use dialog)=w908, text=w907) -> ()  [unwired: 2 in, 3 out]
      }
      event "11": Value Change {
        n145 = event-data() -> ()  [unwired: 1 in, 6 out]
        n146 = Number To Fractional String(number="轴厚度") -> (F-format string=w911:string)  [unwired: 3 in]
        n147 = Open/Create/Replace File(file path (use dialog)=path "H:/新/finaltest.dat" ("文件路径（使用对话框）"), operation (0:open)=T1."replace" ("操作(0:open)")) -> (refnum out=w916:refnum<file>)  [unwired: 4 in, 2 out]
        n148 = Concatenate Strings("/RGB,INDEX,100,100,100, 0   \n/RGB,INDEX, 80, 80, 80,13   \n/RGB,INDEX, 60, 60, 60,14   \n/RGB,INDEX, 0, 0, 0,15  \n\n/REPLOT,RESIZE  \n/CLEAR,NOSTART \nNZ=25 !齿数：\nTH=1.5 !平均齿高：\nWTH=1.5 !外侧斜齿高\nNTH=1.5 !内侧斜齿高\nWDTH=0.0 !齿外侧导角高度\nWDTL=0.0 !齿外侧导水平长度\nNDTH=0.0 !齿内侧导角高度\nNDTL=0.0 !齿内侧导水平长度\nTT=2 !齿厚：\nTW=0.1 !齿槽宽：\nITD=8 !定子齿内圈直径：\nOTD=13.3 !定子齿外圈直径：\nIAD=2.1 !轴内圈直径：\nOAD=6 !轴外圈直径：\nAT=" ("字符串"), w911, " !轴厚度\nPT=0.4 !压电片厚：\nIPD=8 !压电片内圈直径：\nOPD=13.3 !压电片外圈直径：\nEW= ITD-OAD !宽度：\nET=0.2 !厚度：\nEH=0.2 !台阶高：\nBS=4 !波数\nFK=5 !定子分块建模分块数与齿数成整数倍的关系 \n\nNZ=NZ !齿数：\nTH=TH/1000 !齿高：\nWTH=WTH/1000 !外侧斜齿高\nNTH=NTH/1000 !内侧斜齿高\nWDTH=WDTH/1000 !齿外侧导角高度\nWDTL=WDTL/1000 !齿外侧导水平长度\nNDTH=NDTH/1000 !齿内侧导角高度\nNDTL=NDTL/1000 !齿内侧导水平长度\nTT=TT/1000 !齿厚：\nTW=TW/1000 !齿槽宽：\nITD=ITD/1000 !定子齿内圈直径：\nOTD=OTD/1000 !定子齿外圈直径：\nIAD=IAD/1000 !轴内圈直径：\nOAD=OAD/1000 !轴外圈直径：\nAT=AT/1000 !轴厚度\nPT=PT/1000 !压电片厚：\nIPD=IPD/1000 !压电片内圈直径：\nOPD=OPD/1000 !压电片外圈直径：\nEW= EW/1000 !宽度：\nET=ET/1000 !厚度：\nEH=EH/1000 !台阶高：\n\n/PREP7 \n!定义单元和材料属性\nET,1,SOLID185   \nMPTEMP,,,,,,,,  \nMPTEMP,1,0  \nMPDATA,DENS,1,,8290\nMPTEMP,,,,,,,,  \nMPTEMP,1,0  \nMPDATA,EX,1,,1.06E+011   \nMPDATA,PRXY,1,,0.35 \n\nET,2,SOLID5 \nMPTEMP,,,,,,,,  \nMPTEMP,1,0     \nMPDATA,DENS,2,,7750   \nMPTEMP,,,,,,,,  \nMPTEMP,1,0  \nMPDATA,PERX,2,,919E-009\nMPDATA,PERY,2,,919E-009   \nMPDATA,PERZ,2,,826E-009\nTB,PIEZ,2,,,0   \nTBMODIF,1,1,0   \nTBMODIF,1,2,0   \nTBMODIF,1,3,-5.35   \nTBMODIF,2,1,0   \nTBMODIF,2,2,0   \nTBMODIF,2,3,-5.35   \nTBMODIF,3,1,0   \nTBMODIF,3,2,0   \nTBMODIF,3,3,15.78   \nTBMODIF,4,1,0   \nTBMODIF,4,2,0   \nTBMODIF,4,3,0   \nTBMODIF,5,1,0   \nTBMODIF,5,2,12.3\nTBMODIF,5,3,0   \nTBMODIF,6,1,12.3\nTBMODIF,6,2,0   \nTBMODIF,6,3,0   \nTB,ANEL,2,1,21,0\nTBTEMP,0\nTBDATA,,1.2035E+011,7.52E+010,7.51E+010,0,0,0   \nTBDATA,,1.204E+011,7.51E+010,0,0,0,1.109E+011   \nTBDATA,,0,0,0,2.26E+010,0,0 \nTBDATA,,2.12E+010,0,2.11E+010,,,\n\n!超声波电机模型建立\nK,1,OAD/2,,,\nK,2,ITD/2,,,\nK,3,ITD/2,-EH,,!最上面\nK,4,OTD/2,-EH,,\nK,5,OTD/2,-EH+TT-TH,,\nK,6,ITD/2,-EH+TT-TH,,\nK,7,ITD/2,ET,,\nK,8,OAD/2,ET,,\nK,11,ITD/2,-EH-PT,,!最下面\nK,12,OTD/2,-EH-PT,,\nK,13,OTD/2,-EH+TT,,\nK,14,ITD/2,-EH+TT,,\nK,15,IAD/2,ET,,\nK,16,IAD/2,0,,\nK,17,IAD/2,-AT+ET,,\nK,18,OAD/2,-AT+ET,,\n\nK,100,0,0,0,\nK,101,0,0.003,0,\n\nLSTR,1,2\nLSTR,2,3\nLSTR,3,4\nLSTR,4,5\nLSTR,5,6\nLSTR,6,7\nLSTR,7,8\nLSTR,8,1\nLSTR,3,11\nLSTR,11,12\nLSTR,12,4\nLSTR,5,13\nLSTR,13,14\nLSTR,14,6\nLSTR,2,7\nLSTR,8,15\nLSTR,15,16\nLSTR,1,16\nLSTR,16,17\nLSTR,17,18\nLSTR,1,18\n\nAL,1,15,7,8\nAL,15,2,3,4,5,6,\nAL,9,10,11,3\nAL,5,12,13,14\nAL,8,16,17,18\nAL,18,19,20,21\n\nVROTAT,1,2,3,4, , ,100,101 ,360/FK, , !!!!!\nVROTAT,5,6, , , , ,100,101 ,360/FK, , !!!!!\nBLC4,0,TT-EH,OTD,-TH,TW !建立长方体\nVGEN, ,7, , , , ,-TW/2, , ,1!复制创建体  \nVOVLAP,4,7 !布尔操作\nVDELE,10, , ,1!删除体\nVSYMM,Z,8, , , ,0,0 !体镜像 \n\n!建立齿槽\nCSYS,5  \nWPSTYLE,,,,,,,,0\nVGEN,NZ/FK+1,4, , , ,360/NZ, , ,0  \nVGEN,NZ/FK+1,8, , , ,360/NZ, , ,0  \nVOVLAP,ALL\n*DO,I,1,NZ/FK+1\nCSYS,0\nVSEL,S,LOC,Y,TT-EH-TH/1.5,1\nCSYS,5\nVSEL,R,LOC,Y,(I-1)*360/NZ-TW/2/3.1415/ITD*360,TW/2/3.1415/ITD*360+(I-1)*360/NZ!选择体\nVDELE,ALL, , ,1\nALLSEL,ALL \n*ENDDO\n\n!旋转成体\nEPLOT \nCSYS,5 \nVGEN,FK,ALL, , , ,360/FK, , ,0 \n\n!Glue体\nVGLUE,ALL\n\n!添加材料属性\nALLSEL,ALL\nCSYS,0\nVSEL,S,LOC,Y,0,TT-EH\nVATT,       1, ,   1,       0   \nCSYS,5\nVSEL,S,LOC,X,0,OAD/2\nVATT,       1, ,   1,       0 \n\nALLSEL,ALL\nCSYS,0\nVSEL,R,LOC,Y,-EH-PT,-EH\nVATT,       2, ,  2,       0  \nALLSEL,ALL\n\n!网格体\nCSYS,0\nVSEL,R,LOC,Y,-EH-PT,-EH\nVSWEEP,ALL\n\nCSYS,0\nALLSEL,ALL \nVSEL,S,MAT,,1\nSMRT,6  \nSMRT,5  \nSMRT,4  \nMSHAPE,1,3d\nMSHKEY,0\nVMESH,ALL\n\nALLSEL,ALL\n\n!模态分析 \n/SOL  \nANTYPE,2\nMODOPT,LANB,22  \nEQSLV,SPAR  \nMXPAND,0, , ,0  \nLUMPM,0 \nPSTRES,0\nMODOPT,LANB,22,0,80000, ,OFF\n\nCSYS,5\nASEL,S,LOC,X,-IAD/2,IAD/2   \nDA,ALL,ALL,\nALLSEL,ALL\n\n!OUTPR,BASIC,ALL,  \n!OUTRES,ALL,ALL,\n \n/STATUS,SOLU\nSOLVE   \nFINISH\nCSYS,0\nALLSEL,ALL\n\n/POST1  \nSET,FIRST   \n/EFACET,1   \nPLNSOL, U,SUM, 2,1.0 !无轮廓2变0\n/post1\n*do,i,8,22\nset,1,i\n/VIEW,1,1,2,3   \n/ANG,1  \n/REP,FAST  \n/show,jpeg,,\nplnsol,u,sum,0,1.0\n/show,close\n*enddo\nFINISH\n\n!振幅仿真\n/SOL\nANTYPE,3\nHROPT,FULL  \nHROUT,ON\nLUMPM,0 \nEQSLV, ,0,  \nPSTRES,0\n\n!阻尼特性\nALPHAD,0,   \nBETAD,0,\nDMPSTR,0.005,   \n\n!压电耦合\n*do,i,1,(BS-1)\nALLSEL,ALL\ncsys,5\nnsel,S,LOC,X,ITD/2,OTD/2\ncsys,0\nnsel,R,loc,y,-eh-eq-pt\ncsys,5\nangle=360/BS\nnsel,r,loc,y,(i-1)*angle/2,i*angle/2\nb=1/2*(1-(-1)**i)*1\nc=1/2*(1-(-1)**(i+1))*1\nD,All,VOLT,b,c\n*enddo\n\nALLSEL,ALL\ncsys,5\nnsel,S,LOC,X,ITD/2,OTD/2\ncsys,0\nnsel,R,loc,y,-eh-eq-pt\ncsys,5\nangle=360/BS\nnsel,r,loc,y,(BS-1)*angle/2,((BS-1)*angle/2+3*angle/8)\nD,All,VOLT,(1/2*(1-(-1)**BS)*1),(1/2*(1-(-1)**(BS+1))*1)\n\nALLSEL,ALL\ncsys,5\nnsel,S,LOC,X,ITD/2,OTD/2\ncsys,0\nnsel,R,loc,y,-eh-eq-pt\ncsys,5\nangle=360/BS\nnsel,r,loc,y,((BS-1)*angle/2+3*angle/8),((BS-1)*angle/2+3*angle/4)\nD,All,VOLT,(1/2*(1-(-1)**(BS+1))*1),(1/2*(1-(-1)**(BS+2))*1)\n\n*do,i,1,(BS-1)\nALLSEL,ALL\ncsys,5\nnsel,S,LOC,X,ITD/2,OTD/2\ncsys,0\nnsel,R,loc,y,-eh-eq-pt\ncsys,5\nangle=360/BS\nnsel,r,loc,y,((BS-1)*angle/2+3*angle/4+(i-1)*angle/2),((BS-1)*angle/2+3*angle/4+(i)*angle/2)\ne=1/2*(1-(-1)**(BS+1+i))*1\nf=1/2*(1-(-1)**(BS+2+i))*1\nD,All,VOLT,e,f\n*enddo\n\nALLSEL,ALL\ncsys,5\nnsel,S,LOC,X,ITD/2,OTD/2\ncsys,0\nnsel,r,loc,y,-eh-eq\nD,All,VOLT,0,0\nALLSEL,ALL \n\nHARFRQ,26000,76000, \nNSUBST,5,  \nKBC,1\n/STATUS,SOLU\nSOLVE\n\n!选最大位移点\n/POST1\nNSORT,U,SUM,0,1, ,SELECT  \nPRNSOL,U,Z\n*get,node,SORT,0,IMAX\n\n!结果显示,打开后处理器\n/POST26 \nFILE,'finaltest','rst','.'   \n/UI,COLL,1  \nNUMVAR,200  \nSOLU,191,NCMIT  \nSTORE,MERGE \nPLCPLX,0\nPRCPLX,1\nFILLDATA,191,,,,1,1 \nREALVAR,191,191 \n\n!z方向位移 \nNSOL,2,node,U,Z, UZ_2, \nSTORE,MERGE \n\n!保存为txt(excel也行)\n/post26\n! Save time history variables to file zmovement.prn\n*CREATE,scratch,gui \n*DEL,_P26_EXPORT\n*DIM,_P26_EXPORT,TABLE,5,2 \nVGET,_P26_EXPORT(1,0),1 \nVGET,_P26_EXPORT(1,1),2,,0  \nVGET,_P26_EXPORT(1,2),2,,1  \n/OUTPUT,'zmovement','prn','.'  \n*VWRITE,'FREQ','UZ_2',' '   \n%14C %14C %14C\n*VWRITE,' ','REAL','IMAGINARY'  \n%14C %14C %14C  \n*VWRITE,_P26_EXPORT(1,0),_P26_EXPORT(1,1),_P26_EXPORT(1,2)  \n%14.5G %14.5G %14.5G\n/OUTPUT,TERM\n*END\n/INPUT,scratch,gui  \n! End of time history save  \n\n!x方向位移 \nNSOL,3,node,U,X, UX_3, \nSTORE,MERGE \n\n!保存为txt(excel也行)\n/post26\n! Save time history variables to file xmovement.prn\n*CREATE,scratch,gui \n*DEL,_P26_EXPORT\n*DIM,_P26_EXPORT,TABLE,5,2 \nVGET,_P26_EXPORT(1,0),1 \nVGET,_P26_EXPORT(1,1),3,,0  \nVGET,_P26_EXPORT(1,2),3,,1  \n/OUTPUT,'xmovement','prn','.'  \n*VWRITE,'FREQ','UX_3',' '   \n%14C %14C %14C  \n*VWRITE,' ','REAL','IMAGINARY'  \n%14C %14C %14C  \n*VWRITE,_P26_EXPORT(1,0),_P26_EXPORT(1,1),_P26_EXPORT(1,2)  \n%14.5G %14.5G %14.5G\n/OUTPUT,TERM\n*END\n/INPUT,scratch,gui  \n! End of time history save\n\n!y方向位移 \nNSOL,4,node,U,Y, UY_4, \nSTORE,MERGE \n\n!保存为txt(excel也行)\n/post26\n! Save time history variables to file ymovement.prn\n*CREATE,scratch,gui \n*DEL,_P26_EXPORT\n*DIM,_P26_EXPORT,TABLE,5,2 \nVGET,_P26_EXPORT(1,0),1 \nVGET,_P26_EXPORT(1,1),4,,0  \nVGET,_P26_EXPORT(1,2),4,,1  \n/OUTPUT,'ymovement','prn','.'  \n*VWRITE,'FREQ','UY_4',' '   \n%14C %14C %14C  \n*VWRITE,' ','REAL','IMAGINARY'  \n%14C %14C %14C  \n*VWRITE,_P26_EXPORT(1,0),_P26_EXPORT(1,1),_P26_EXPORT(1,2)  \n%14.5G %14.5G %14.5G\n/OUTPUT,TERM\n*END\n/INPUT,scratch,gui  \n! End of time history save\n\n!选择电流点\nRFORCE,2,180,AMPS,, AMPS_2  \nSTORE,MERGE \nFILLDATA,192,,,,0,0 \nFILLDATA,193,,,,1,0 \nFILLDATA,194,,,,-1,0\nFILLDATA,195,,,,1,1 \nVARNAME,195,NSET\n! Name: Z   \n! ID:  3\n! Function: 1/{AMPS_2}  \nFILLDATA,199,,,,1,0 \nREALVAR,199,199 \nQUOT,3,199,2,,Z \nSTORE,MERGE \n\n!保存为txt(excel也行)\n/post26\n! Save time history variables to file current.prn   \n*CREATE,scratch,gui \n*DEL,_P26_EXPORT\n*DIM,_P26_EXPORT,TABLE,5,2 \nVGET,_P26_EXPORT(1,0),1 \nVGET,_P26_EXPORT(1,1),3,,0  \nVGET,_P26_EXPORT(1,2),3,,1  \n/OUTPUT,'current','prn','.' \n*VWRITE,'FREQ','Z',' '  \n%14C %14C %14C  \n*VWRITE,' ','REAL','IMAGINARY'  \n%14C %14C %14C  \n*VWRITE,_P26_EXPORT(1,0),_P26_EXPORT(1,1),_P26_EXPORT(1,2)  \n%14.5G %14.5G %14.5G\n/OUTPUT,TERM\n*END\n/INPUT,scratch,gui  \n! End of time history save " ("字符串")) -> (w915:string)
        n149 = Write to Text File(file (use dialog)=w916, text=w915) -> ()  [unwired: 2 in, 3 out]
      }
      event "12": Value Change {
        n150 = event-data() -> ()  [unwired: 1 in, 6 out]
        n151 = Number To Fractional String(number="压电片厚") -> (F-format string=w919:string)  [unwired: 3 in]
        n152 = Open/Create/Replace File(file path (use dialog)=path "H:/新/finaltest.dat" ("文件路径（使用对话框）"), operation (0:open)=T1."replace" ("操作(0:open)")) -> (refnum out=w924:refnum<file>)  [unwired: 4 in, 2 out]
        n153 = Concatenate Strings("/RGB,INDEX,100,100,100, 0   \n/RGB,INDEX, 80, 80, 80,13   \n/RGB,INDEX, 60, 60, 60,14   \n/RGB,INDEX, 0, 0, 0,15  \n\n/REPLOT,RESIZE  \n/CLEAR,NOSTART \nNZ=25 !齿数：\nTH=1.5 !平均齿高：\nWTH=1.5 !外侧斜齿高\nNTH=1.5 !内侧斜齿高\nWDTH=0.0 !齿外侧导角高度\nWDTL=0.0 !齿外侧导水平长度\nNDTH=0.0 !齿内侧导角高度\nNDTL=0.0 !齿内侧导水平长度\nTT=2 !齿厚：\nTW=0.1 !齿槽宽：\nITD=8 !定子齿内圈直径：\nOTD=13.3 !定子齿外圈直径：\nIAD=2.1 !轴内圈直径：\nOAD=6 !轴外圈直径：\nAT=1.6 !轴厚度\nPT=" ("字符串"), w919, " !压电片厚：\nIPD=8 !压电片内圈直径：\nOPD=13.3 !压电片外圈直径：\nEW= ITD-OAD !宽度：\nET=0.2 !厚度：\nEH=0.2 !台阶高：\nBS=4 !波数\nFK=5 !定子分块建模分块数与齿数成整数倍的关系 \n\nNZ=NZ !齿数：\nTH=TH/1000 !齿高：\nWTH=WTH/1000 !外侧斜齿高\nNTH=NTH/1000 !内侧斜齿高\nWDTH=WDTH/1000 !齿外侧导角高度\nWDTL=WDTL/1000 !齿外侧导水平长度\nNDTH=NDTH/1000 !齿内侧导角高度\nNDTL=NDTL/1000 !齿内侧导水平长度\nTT=TT/1000 !齿厚：\nTW=TW/1000 !齿槽宽：\nITD=ITD/1000 !定子齿内圈直径：\nOTD=OTD/1000 !定子齿外圈直径：\nIAD=IAD/1000 !轴内圈直径：\nOAD=OAD/1000 !轴外圈直径：\nAT=AT/1000 !轴厚度\nPT=PT/1000 !压电片厚：\nIPD=IPD/1000 !压电片内圈直径：\nOPD=OPD/1000 !压电片外圈直径：\nEW= EW/1000 !宽度：\nET=ET/1000 !厚度：\nEH=EH/1000 !台阶高：\n\n/PREP7 \n!定义单元和材料属性\nET,1,SOLID185   \nMPTEMP,,,,,,,,  \nMPTEMP,1,0  \nMPDATA,DENS,1,,8290\nMPTEMP,,,,,,,,  \nMPTEMP,1,0  \nMPDATA,EX,1,,1.06E+011   \nMPDATA,PRXY,1,,0.35 \n\nET,2,SOLID5 \nMPTEMP,,,,,,,,  \nMPTEMP,1,0     \nMPDATA,DENS,2,,7750   \nMPTEMP,,,,,,,,  \nMPTEMP,1,0  \nMPDATA,PERX,2,,919E-009\nMPDATA,PERY,2,,919E-009   \nMPDATA,PERZ,2,,826E-009\nTB,PIEZ,2,,,0   \nTBMODIF,1,1,0   \nTBMODIF,1,2,0   \nTBMODIF,1,3,-5.35   \nTBMODIF,2,1,0   \nTBMODIF,2,2,0   \nTBMODIF,2,3,-5.35   \nTBMODIF,3,1,0   \nTBMODIF,3,2,0   \nTBMODIF,3,3,15.78   \nTBMODIF,4,1,0   \nTBMODIF,4,2,0   \nTBMODIF,4,3,0   \nTBMODIF,5,1,0   \nTBMODIF,5,2,12.3\nTBMODIF,5,3,0   \nTBMODIF,6,1,12.3\nTBMODIF,6,2,0   \nTBMODIF,6,3,0   \nTB,ANEL,2,1,21,0\nTBTEMP,0\nTBDATA,,1.2035E+011,7.52E+010,7.51E+010,0,0,0   \nTBDATA,,1.204E+011,7.51E+010,0,0,0,1.109E+011   \nTBDATA,,0,0,0,2.26E+010,0,0 \nTBDATA,,2.12E+010,0,2.11E+010,,,\n\n!超声波电机模型建立\nK,1,OAD/2,,,\nK,2,ITD/2,,,\nK,3,ITD/2,-EH,,!最上面\nK,4,OTD/2,-EH,,\nK,5,OTD/2,-EH+TT-TH,,\nK,6,ITD/2,-EH+TT-TH,,\nK,7,ITD/2,ET,,\nK,8,OAD/2,ET,,\nK,11,ITD/2,-EH-PT,,!最下面\nK,12,OTD/2,-EH-PT,,\nK,13,OTD/2,-EH+TT,,\nK,14,ITD/2,-EH+TT,,\nK,15,IAD/2,ET,,\nK,16,IAD/2,0,,\nK,17,IAD/2,-AT+ET,,\nK,18,OAD/2,-AT+ET,,\n\nK,100,0,0,0,\nK,101,0,0.003,0,\n\nLSTR,1,2\nLSTR,2,3\nLSTR,3,4\nLSTR,4,5\nLSTR,5,6\nLSTR,6,7\nLSTR,7,8\nLSTR,8,1\nLSTR,3,11\nLSTR,11,12\nLSTR,12,4\nLSTR,5,13\nLSTR,13,14\nLSTR,14,6\nLSTR,2,7\nLSTR,8,15\nLSTR,15,16\nLSTR,1,16\nLSTR,16,17\nLSTR,17,18\nLSTR,1,18\n\nAL,1,15,7,8\nAL,15,2,3,4,5,6,\nAL,9,10,11,3\nAL,5,12,13,14\nAL,8,16,17,18\nAL,18,19,20,21\n\nVROTAT,1,2,3,4, , ,100,101 ,360/FK, , !!!!!\nVROTAT,5,6, , , , ,100,101 ,360/FK, , !!!!!\nBLC4,0,TT-EH,OTD,-TH,TW !建立长方体\nVGEN, ,7, , , , ,-TW/2, , ,1!复制创建体  \nVOVLAP,4,7 !布尔操作\nVDELE,10, , ,1!删除体\nVSYMM,Z,8, , , ,0,0 !体镜像 \n\n!建立齿槽\nCSYS,5  \nWPSTYLE,,,,,,,,0\nVGEN,NZ/FK+1,4, , , ,360/NZ, , ,0  \nVGEN,NZ/FK+1,8, , , ,360/NZ, , ,0  \nVOVLAP,ALL\n*DO,I,1,NZ/FK+1\nCSYS,0\nVSEL,S,LOC,Y,TT-EH-TH/1.5,1\nCSYS,5\nVSEL,R,LOC,Y,(I-1)*360/NZ-TW/2/3.1415/ITD*360,TW/2/3.1415/ITD*360+(I-1)*360/NZ!选择体\nVDELE,ALL, , ,1\nALLSEL,ALL \n*ENDDO\n\n!旋转成体\nEPLOT \nCSYS,5 \nVGEN,FK,ALL, , , ,360/FK, , ,0 \n\n!Glue体\nVGLUE,ALL\n\n!添加材料属性\nALLSEL,ALL\nCSYS,0\nVSEL,S,LOC,Y,0,TT-EH\nVATT,       1, ,   1,       0   \nCSYS,5\nVSEL,S,LOC,X,0,OAD/2\nVATT,       1, ,   1,       0 \n\nALLSEL,ALL\nCSYS,0\nVSEL,R,LOC,Y,-EH-PT,-EH\nVATT,       2, ,  2,       0  \nALLSEL,ALL\n\n!网格体\nCSYS,0\nVSEL,R,LOC,Y,-EH-PT,-EH\nVSWEEP,ALL\n\nCSYS,0\nALLSEL,ALL \nVSEL,S,MAT,,1\nSMRT,6  \nSMRT,5  \nSMRT,4  \nMSHAPE,1,3d\nMSHKEY,0\nVMESH,ALL\n\nALLSEL,ALL\n\n!模态分析 \n/SOL  \nANTYPE,2\nMODOPT,LANB,22  \nEQSLV,SPAR  \nMXPAND,0, , ,0  \nLUMPM,0 \nPSTRES,0\nMODOPT,LANB,22,0,80000, ,OFF\n\nCSYS,5\nASEL,S,LOC,X,-IAD/2,IAD/2   \nDA,ALL,ALL,\nALLSEL,ALL\n\n!OUTPR,BASIC,ALL,  \n!OUTRES,ALL,ALL,\n \n/STATUS,SOLU\nSOLVE   \nFINISH\nCSYS,0\nALLSEL,ALL\n\n/POST1  \nSET,FIRST   \n/EFACET,1   \nPLNSOL, U,SUM, 2,1.0 !无轮廓2变0\n/post1\n*do,i,8,22\nset,1,i\n/VIEW,1,1,2,3   \n/ANG,1  \n/REP,FAST  \n/show,jpeg,,\nplnsol,u,sum,0,1.0\n/show,close\n*enddo\nFINISH\n\n!振幅仿真\n/SOL\nANTYPE,3\nHROPT,FULL  \nHROUT,ON\nLUMPM,0 \nEQSLV, ,0,  \nPSTRES,0\n\n!阻尼特性\nALPHAD,0,   \nBETAD,0,\nDMPSTR,0.005,   \n\n!压电耦合\n*do,i,1,(BS-1)\nALLSEL,ALL\ncsys,5\nnsel,S,LOC,X,ITD/2,OTD/2\ncsys,0\nnsel,R,loc,y,-eh-eq-pt\ncsys,5\nangle=360/BS\nnsel,r,loc,y,(i-1)*angle/2,i*angle/2\nb=1/2*(1-(-1)**i)*1\nc=1/2*(1-(-1)**(i+1))*1\nD,All,VOLT,b,c\n*enddo\n\nALLSEL,ALL\ncsys,5\nnsel,S,LOC,X,ITD/2,OTD/2\ncsys,0\nnsel,R,loc,y,-eh-eq-pt\ncsys,5\nangle=360/BS\nnsel,r,loc,y,(BS-1)*angle/2,((BS-1)*angle/2+3*angle/8)\nD,All,VOLT,(1/2*(1-(-1)**BS)*1),(1/2*(1-(-1)**(BS+1))*1)\n\nALLSEL,ALL\ncsys,5\nnsel,S,LOC,X,ITD/2,OTD/2\ncsys,0\nnsel,R,loc,y,-eh-eq-pt\ncsys,5\nangle=360/BS\nnsel,r,loc,y,((BS-1)*angle/2+3*angle/8),((BS-1)*angle/2+3*angle/4)\nD,All,VOLT,(1/2*(1-(-1)**(BS+1))*1),(1/2*(1-(-1)**(BS+2))*1)\n\n*do,i,1,(BS-1)\nALLSEL,ALL\ncsys,5\nnsel,S,LOC,X,ITD/2,OTD/2\ncsys,0\nnsel,R,loc,y,-eh-eq-pt\ncsys,5\nangle=360/BS\nnsel,r,loc,y,((BS-1)*angle/2+3*angle/4+(i-1)*angle/2),((BS-1)*angle/2+3*angle/4+(i)*angle/2)\ne=1/2*(1-(-1)**(BS+1+i))*1\nf=1/2*(1-(-1)**(BS+2+i))*1\nD,All,VOLT,e,f\n*enddo\n\nALLSEL,ALL\ncsys,5\nnsel,S,LOC,X,ITD/2,OTD/2\ncsys,0\nnsel,r,loc,y,-eh-eq\nD,All,VOLT,0,0\nALLSEL,ALL \n\nHARFRQ,26000,76000, \nNSUBST,5,  \nKBC,1\n/STATUS,SOLU\nSOLVE\n\n!选最大位移点\n/POST1\nNSORT,U,SUM,0,1, ,SELECT  \nPRNSOL,U,Z\n*get,node,SORT,0,IMAX\n\n!结果显示,打开后处理器\n/POST26 \nFILE,'finaltest','rst','.'   \n/UI,COLL,1  \nNUMVAR,200  \nSOLU,191,NCMIT  \nSTORE,MERGE \nPLCPLX,0\nPRCPLX,1\nFILLDATA,191,,,,1,1 \nREALVAR,191,191 \n\n!z方向位移 \nNSOL,2,node,U,Z, UZ_2, \nSTORE,MERGE \n\n!保存为txt(excel也行)\n/post26\n! Save time history variables to file zmovement.prn\n*CREATE,scratch,gui \n*DEL,_P26_EXPORT\n*DIM,_P26_EXPORT,TABLE,5,2 \nVGET,_P26_EXPORT(1,0),1 \nVGET,_P26_EXPORT(1,1),2,,0  \nVGET,_P26_EXPORT(1,2),2,,1  \n/OUTPUT,'zmovement','prn','.'  \n*VWRITE,'FREQ','UZ_2',' '   \n%14C %14C %14C\n*VWRITE,' ','REAL','IMAGINARY'  \n%14C %14C %14C  \n*VWRITE,_P26_EXPORT(1,0),_P26_EXPORT(1,1),_P26_EXPORT(1,2)  \n%14.5G %14.5G %14.5G\n/OUTPUT,TERM\n*END\n/INPUT,scratch,gui  \n! End of time history save  \n\n!x方向位移 \nNSOL,3,node,U,X, UX_3, \nSTORE,MERGE \n\n!保存为txt(excel也行)\n/post26\n! Save time history variables to file xmovement.prn\n*CREATE,scratch,gui \n*DEL,_P26_EXPORT\n*DIM,_P26_EXPORT,TABLE,5,2 \nVGET,_P26_EXPORT(1,0),1 \nVGET,_P26_EXPORT(1,1),3,,0  \nVGET,_P26_EXPORT(1,2),3,,1  \n/OUTPUT,'xmovement','prn','.'  \n*VWRITE,'FREQ','UX_3',' '   \n%14C %14C %14C  \n*VWRITE,' ','REAL','IMAGINARY'  \n%14C %14C %14C  \n*VWRITE,_P26_EXPORT(1,0),_P26_EXPORT(1,1),_P26_EXPORT(1,2)  \n%14.5G %14.5G %14.5G\n/OUTPUT,TERM\n*END\n/INPUT,scratch,gui  \n! End of time history save\n\n!y方向位移 \nNSOL,4,node,U,Y, UY_4, \nSTORE,MERGE \n\n!保存为txt(excel也行)\n/post26\n! Save time history variables to file ymovement.prn\n*CREATE,scratch,gui \n*DEL,_P26_EXPORT\n*DIM,_P26_EXPORT,TABLE,5,2 \nVGET,_P26_EXPORT(1,0),1 \nVGET,_P26_EXPORT(1,1),4,,0  \nVGET,_P26_EXPORT(1,2),4,,1  \n/OUTPUT,'ymovement','prn','.'  \n*VWRITE,'FREQ','UY_4',' '   \n%14C %14C %14C  \n*VWRITE,' ','REAL','IMAGINARY'  \n%14C %14C %14C  \n*VWRITE,_P26_EXPORT(1,0),_P26_EXPORT(1,1),_P26_EXPORT(1,2)  \n%14.5G %14.5G %14.5G\n/OUTPUT,TERM\n*END\n/INPUT,scratch,gui  \n! End of time history save\n\n!选择电流点\nRFORCE,2,180,AMPS,, AMPS_2  \nSTORE,MERGE \nFILLDATA,192,,,,0,0 \nFILLDATA,193,,,,1,0 \nFILLDATA,194,,,,-1,0\nFILLDATA,195,,,,1,1 \nVARNAME,195,NSET\n! Name: Z   \n! ID:  3\n! Function: 1/{AMPS_2}  \nFILLDATA,199,,,,1,0 \nREALVAR,199,199 \nQUOT,3,199,2,,Z \nSTORE,MERGE \n\n!保存为txt(excel也行)\n/post26\n! Save time history variables to file current.prn   \n*CREATE,scratch,gui \n*DEL,_P26_EXPORT\n*DIM,_P26_EXPORT,TABLE,5,2 \nVGET,_P26_EXPORT(1,0),1 \nVGET,_P26_EXPORT(1,1),3,,0  \nVGET,_P26_EXPORT(1,2),3,,1  \n/OUTPUT,'current','prn','.' \n*VWRITE,'FREQ','Z',' '  \n%14C %14C %14C  \n*VWRITE,' ','REAL','IMAGINARY'  \n%14C %14C %14C  \n*VWRITE,_P26_EXPORT(1,0),_P26_EXPORT(1,1),_P26_EXPORT(1,2)  \n%14.5G %14.5G %14.5G\n/OUTPUT,TERM\n*END\n/INPUT,scratch,gui  \n! End of time history save " ("字符串")) -> (w923:string)
        n154 = Write to Text File(file (use dialog)=w924, text=w923) -> ()  [unwired: 2 in, 3 out]
      }
      event "13": Value Change {
        n155 = event-data() -> ()  [unwired: 1 in, 6 out]
        n156 = Number To Fractional String(number="压电片内圈直径") -> (F-format string=w927:string)  [unwired: 3 in]
        n157 = Open/Create/Replace File(file path (use dialog)=path "H:/新/finaltest.dat" ("文件路径（使用对话框）"), operation (0:open)=T1."replace" ("操作(0:open)")) -> (refnum out=w932:refnum<file>)  [unwired: 4 in, 2 out]
        n158 = Concatenate Strings("/RGB,INDEX,100,100,100, 0   \n/RGB,INDEX, 80, 80, 80,13   \n/RGB,INDEX, 60, 60, 60,14   \n/RGB,INDEX, 0, 0, 0,15  \n\n/REPLOT,RESIZE  \n/CLEAR,NOSTART \nNZ=25 !齿数：\nTH=1.5 !平均齿高：\nWTH=1.5 !外侧斜齿高\nNTH=1.5 !内侧斜齿高\nWDTH=0.0 !齿外侧导角高度\nWDTL=0.0 !齿外侧导水平长度\nNDTH=0.0 !齿内侧导角高度\nNDTL=0.0 !齿内侧导水平长度\nTT=2 !齿厚：\nTW=0.1 !齿槽宽：\nITD=8 !定子齿内圈直径：\nOTD=13.3 !定子齿外圈直径：\nIAD=2.1 !轴内圈直径：\nOAD=6 !轴外圈直径：\nAT=1.6 !轴厚度\nPT=0.4 !压电片厚：\nIPD=" ("字符串"), w927, " !压电片内圈直径：\nOPD=13.3 !压电片外圈直径：\nEW= ITD-OAD !宽度：\nET=0.2 !厚度：\nEH=0.2 !台阶高：\nBS=4 !波数\nFK=5 !定子分块建模分块数与齿数成整数倍的关系 \n\nNZ=NZ !齿数：\nTH=TH/1000 !齿高：\nWTH=WTH/1000 !外侧斜齿高\nNTH=NTH/1000 !内侧斜齿高\nWDTH=WDTH/1000 !齿外侧导角高度\nWDTL=WDTL/1000 !齿外侧导水平长度\nNDTH=NDTH/1000 !齿内侧导角高度\nNDTL=NDTL/1000 !齿内侧导水平长度\nTT=TT/1000 !齿厚：\nTW=TW/1000 !齿槽宽：\nITD=ITD/1000 !定子齿内圈直径：\nOTD=OTD/1000 !定子齿外圈直径：\nIAD=IAD/1000 !轴内圈直径：\nOAD=OAD/1000 !轴外圈直径：\nAT=AT/1000 !轴厚度\nPT=PT/1000 !压电片厚：\nIPD=IPD/1000 !压电片内圈直径：\nOPD=OPD/1000 !压电片外圈直径：\nEW= EW/1000 !宽度：\nET=ET/1000 !厚度：\nEH=EH/1000 !台阶高：\n\n/PREP7 \n!定义单元和材料属性\nET,1,SOLID185   \nMPTEMP,,,,,,,,  \nMPTEMP,1,0  \nMPDATA,DENS,1,,8290\nMPTEMP,,,,,,,,  \nMPTEMP,1,0  \nMPDATA,EX,1,,1.06E+011   \nMPDATA,PRXY,1,,0.35 \n\nET,2,SOLID5 \nMPTEMP,,,,,,,,  \nMPTEMP,1,0     \nMPDATA,DENS,2,,7750   \nMPTEMP,,,,,,,,  \nMPTEMP,1,0  \nMPDATA,PERX,2,,919E-009\nMPDATA,PERY,2,,919E-009   \nMPDATA,PERZ,2,,826E-009\nTB,PIEZ,2,,,0   \nTBMODIF,1,1,0   \nTBMODIF,1,2,0   \nTBMODIF,1,3,-5.35   \nTBMODIF,2,1,0   \nTBMODIF,2,2,0   \nTBMODIF,2,3,-5.35   \nTBMODIF,3,1,0   \nTBMODIF,3,2,0   \nTBMODIF,3,3,15.78   \nTBMODIF,4,1,0   \nTBMODIF,4,2,0   \nTBMODIF,4,3,0   \nTBMODIF,5,1,0   \nTBMODIF,5,2,12.3\nTBMODIF,5,3,0   \nTBMODIF,6,1,12.3\nTBMODIF,6,2,0   \nTBMODIF,6,3,0   \nTB,ANEL,2,1,21,0\nTBTEMP,0\nTBDATA,,1.2035E+011,7.52E+010,7.51E+010,0,0,0   \nTBDATA,,1.204E+011,7.51E+010,0,0,0,1.109E+011   \nTBDATA,,0,0,0,2.26E+010,0,0 \nTBDATA,,2.12E+010,0,2.11E+010,,,\n\n!超声波电机模型建立\nK,1,OAD/2,,,\nK,2,ITD/2,,,\nK,3,ITD/2,-EH,,!最上面\nK,4,OTD/2,-EH,,\nK,5,OTD/2,-EH+TT-TH,,\nK,6,ITD/2,-EH+TT-TH,,\nK,7,ITD/2,ET,,\nK,8,OAD/2,ET,,\nK,11,ITD/2,-EH-PT,,!最下面\nK,12,OTD/2,-EH-PT,,\nK,13,OTD/2,-EH+TT,,\nK,14,ITD/2,-EH+TT,,\nK,15,IAD/2,ET,,\nK,16,IAD/2,0,,\nK,17,IAD/2,-AT+ET,,\nK,18,OAD/2,-AT+ET,,\n\nK,100,0,0,0,\nK,101,0,0.003,0,\n\nLSTR,1,2\nLSTR,2,3\nLSTR,3,4\nLSTR,4,5\nLSTR,5,6\nLSTR,6,7\nLSTR,7,8\nLSTR,8,1\nLSTR,3,11\nLSTR,11,12\nLSTR,12,4\nLSTR,5,13\nLSTR,13,14\nLSTR,14,6\nLSTR,2,7\nLSTR,8,15\nLSTR,15,16\nLSTR,1,16\nLSTR,16,17\nLSTR,17,18\nLSTR,1,18\n\nAL,1,15,7,8\nAL,15,2,3,4,5,6,\nAL,9,10,11,3\nAL,5,12,13,14\nAL,8,16,17,18\nAL,18,19,20,21\n\nVROTAT,1,2,3,4, , ,100,101 ,360/FK, , !!!!!\nVROTAT,5,6, , , , ,100,101 ,360/FK, , !!!!!\nBLC4,0,TT-EH,OTD,-TH,TW !建立长方体\nVGEN, ,7, , , , ,-TW/2, , ,1!复制创建体  \nVOVLAP,4,7 !布尔操作\nVDELE,10, , ,1!删除体\nVSYMM,Z,8, , , ,0,0 !体镜像 \n\n!建立齿槽\nCSYS,5  \nWPSTYLE,,,,,,,,0\nVGEN,NZ/FK+1,4, , , ,360/NZ, , ,0  \nVGEN,NZ/FK+1,8, , , ,360/NZ, , ,0  \nVOVLAP,ALL\n*DO,I,1,NZ/FK+1\nCSYS,0\nVSEL,S,LOC,Y,TT-EH-TH/1.5,1\nCSYS,5\nVSEL,R,LOC,Y,(I-1)*360/NZ-TW/2/3.1415/ITD*360,TW/2/3.1415/ITD*360+(I-1)*360/NZ!选择体\nVDELE,ALL, , ,1\nALLSEL,ALL \n*ENDDO\n\n!旋转成体\nEPLOT \nCSYS,5 \nVGEN,FK,ALL, , , ,360/FK, , ,0 \n\n!Glue体\nVGLUE,ALL\n\n!添加材料属性\nALLSEL,ALL\nCSYS,0\nVSEL,S,LOC,Y,0,TT-EH\nVATT,       1, ,   1,       0   \nCSYS,5\nVSEL,S,LOC,X,0,OAD/2\nVATT,       1, ,   1,       0 \n\nALLSEL,ALL\nCSYS,0\nVSEL,R,LOC,Y,-EH-PT,-EH\nVATT,       2, ,  2,       0  \nALLSEL,ALL\n\n!网格体\nCSYS,0\nVSEL,R,LOC,Y,-EH-PT,-EH\nVSWEEP,ALL\n\nCSYS,0\nALLSEL,ALL \nVSEL,S,MAT,,1\nSMRT,6  \nSMRT,5  \nSMRT,4  \nMSHAPE,1,3d\nMSHKEY,0\nVMESH,ALL\n\nALLSEL,ALL\n\n!模态分析 \n/SOL  \nANTYPE,2\nMODOPT,LANB,22  \nEQSLV,SPAR  \nMXPAND,0, , ,0  \nLUMPM,0 \nPSTRES,0\nMODOPT,LANB,22,0,80000, ,OFF\n\nCSYS,5\nASEL,S,LOC,X,-IAD/2,IAD/2   \nDA,ALL,ALL,\nALLSEL,ALL\n\n!OUTPR,BASIC,ALL,  \n!OUTRES,ALL,ALL,\n \n/STATUS,SOLU\nSOLVE   \nFINISH\nCSYS,0\nALLSEL,ALL\n\n/POST1  \nSET,FIRST   \n/EFACET,1   \nPLNSOL, U,SUM, 2,1.0 !无轮廓2变0\n/post1\n*do,i,8,22\nset,1,i\n/VIEW,1,1,2,3   \n/ANG,1  \n/REP,FAST  \n/show,jpeg,,\nplnsol,u,sum,0,1.0\n/show,close\n*enddo\nFINISH\n\n!振幅仿真\n/SOL\nANTYPE,3\nHROPT,FULL  \nHROUT,ON\nLUMPM,0 \nEQSLV, ,0,  \nPSTRES,0\n\n!阻尼特性\nALPHAD,0,   \nBETAD,0,\nDMPSTR,0.005,   \n\n!压电耦合\n*do,i,1,(BS-1)\nALLSEL,ALL\ncsys,5\nnsel,S,LOC,X,ITD/2,OTD/2\ncsys,0\nnsel,R,loc,y,-eh-eq-pt\ncsys,5\nangle=360/BS\nnsel,r,loc,y,(i-1)*angle/2,i*angle/2\nb=1/2*(1-(-1)**i)*1\nc=1/2*(1-(-1)**(i+1))*1\nD,All,VOLT,b,c\n*enddo\n\nALLSEL,ALL\ncsys,5\nnsel,S,LOC,X,ITD/2,OTD/2\ncsys,0\nnsel,R,loc,y,-eh-eq-pt\ncsys,5\nangle=360/BS\nnsel,r,loc,y,(BS-1)*angle/2,((BS-1)*angle/2+3*angle/8)\nD,All,VOLT,(1/2*(1-(-1)**BS)*1),(1/2*(1-(-1)**(BS+1))*1)\n\nALLSEL,ALL\ncsys,5\nnsel,S,LOC,X,ITD/2,OTD/2\ncsys,0\nnsel,R,loc,y,-eh-eq-pt\ncsys,5\nangle=360/BS\nnsel,r,loc,y,((BS-1)*angle/2+3*angle/8),((BS-1)*angle/2+3*angle/4)\nD,All,VOLT,(1/2*(1-(-1)**(BS+1))*1),(1/2*(1-(-1)**(BS+2))*1)\n\n*do,i,1,(BS-1)\nALLSEL,ALL\ncsys,5\nnsel,S,LOC,X,ITD/2,OTD/2\ncsys,0\nnsel,R,loc,y,-eh-eq-pt\ncsys,5\nangle=360/BS\nnsel,r,loc,y,((BS-1)*angle/2+3*angle/4+(i-1)*angle/2),((BS-1)*angle/2+3*angle/4+(i)*angle/2)\ne=1/2*(1-(-1)**(BS+1+i))*1\nf=1/2*(1-(-1)**(BS+2+i))*1\nD,All,VOLT,e,f\n*enddo\n\nALLSEL,ALL\ncsys,5\nnsel,S,LOC,X,ITD/2,OTD/2\ncsys,0\nnsel,r,loc,y,-eh-eq\nD,All,VOLT,0,0\nALLSEL,ALL \n\nHARFRQ,26000,76000, \nNSUBST,5,  \nKBC,1\n/STATUS,SOLU\nSOLVE\n\n!选最大位移点\n/POST1\nNSORT,U,SUM,0,1, ,SELECT  \nPRNSOL,U,Z\n*get,node,SORT,0,IMAX\n\n!结果显示,打开后处理器\n/POST26 \nFILE,'finaltest','rst','.'   \n/UI,COLL,1  \nNUMVAR,200  \nSOLU,191,NCMIT  \nSTORE,MERGE \nPLCPLX,0\nPRCPLX,1\nFILLDATA,191,,,,1,1 \nREALVAR,191,191 \n\n!z方向位移 \nNSOL,2,node,U,Z, UZ_2, \nSTORE,MERGE \n\n!保存为txt(excel也行)\n/post26\n! Save time history variables to file zmovement.prn\n*CREATE,scratch,gui \n*DEL,_P26_EXPORT\n*DIM,_P26_EXPORT,TABLE,5,2 \nVGET,_P26_EXPORT(1,0),1 \nVGET,_P26_EXPORT(1,1),2,,0  \nVGET,_P26_EXPORT(1,2),2,,1  \n/OUTPUT,'zmovement','prn','.'  \n*VWRITE,'FREQ','UZ_2',' '   \n%14C %14C %14C\n*VWRITE,' ','REAL','IMAGINARY'  \n%14C %14C %14C  \n*VWRITE,_P26_EXPORT(1,0),_P26_EXPORT(1,1),_P26_EXPORT(1,2)  \n%14.5G %14.5G %14.5G\n/OUTPUT,TERM\n*END\n/INPUT,scratch,gui  \n! End of time history save  \n\n!x方向位移 \nNSOL,3,node,U,X, UX_3, \nSTORE,MERGE \n\n!保存为txt(excel也行)\n/post26\n! Save time history variables to file xmovement.prn\n*CREATE,scratch,gui \n*DEL,_P26_EXPORT\n*DIM,_P26_EXPORT,TABLE,5,2 \nVGET,_P26_EXPORT(1,0),1 \nVGET,_P26_EXPORT(1,1),3,,0  \nVGET,_P26_EXPORT(1,2),3,,1  \n/OUTPUT,'xmovement','prn','.'  \n*VWRITE,'FREQ','UX_3',' '   \n%14C %14C %14C  \n*VWRITE,' ','REAL','IMAGINARY'  \n%14C %14C %14C  \n*VWRITE,_P26_EXPORT(1,0),_P26_EXPORT(1,1),_P26_EXPORT(1,2)  \n%14.5G %14.5G %14.5G\n/OUTPUT,TERM\n*END\n/INPUT,scratch,gui  \n! End of time history save\n\n!y方向位移 \nNSOL,4,node,U,Y, UY_4, \nSTORE,MERGE \n\n!保存为txt(excel也行)\n/post26\n! Save time history variables to file ymovement.prn\n*CREATE,scratch,gui \n*DEL,_P26_EXPORT\n*DIM,_P26_EXPORT,TABLE,5,2 \nVGET,_P26_EXPORT(1,0),1 \nVGET,_P26_EXPORT(1,1),4,,0  \nVGET,_P26_EXPORT(1,2),4,,1  \n/OUTPUT,'ymovement','prn','.'  \n*VWRITE,'FREQ','UY_4',' '   \n%14C %14C %14C  \n*VWRITE,' ','REAL','IMAGINARY'  \n%14C %14C %14C  \n*VWRITE,_P26_EXPORT(1,0),_P26_EXPORT(1,1),_P26_EXPORT(1,2)  \n%14.5G %14.5G %14.5G\n/OUTPUT,TERM\n*END\n/INPUT,scratch,gui  \n! End of time history save\n\n!选择电流点\nRFORCE,2,180,AMPS,, AMPS_2  \nSTORE,MERGE \nFILLDATA,192,,,,0,0 \nFILLDATA,193,,,,1,0 \nFILLDATA,194,,,,-1,0\nFILLDATA,195,,,,1,1 \nVARNAME,195,NSET\n! Name: Z   \n! ID:  3\n! Function: 1/{AMPS_2}  \nFILLDATA,199,,,,1,0 \nREALVAR,199,199 \nQUOT,3,199,2,,Z \nSTORE,MERGE \n\n!保存为txt(excel也行)\n/post26\n! Save time history variables to file current.prn   \n*CREATE,scratch,gui \n*DEL,_P26_EXPORT\n*DIM,_P26_EXPORT,TABLE,5,2 \nVGET,_P26_EXPORT(1,0),1 \nVGET,_P26_EXPORT(1,1),3,,0  \nVGET,_P26_EXPORT(1,2),3,,1  \n/OUTPUT,'current','prn','.' \n*VWRITE,'FREQ','Z',' '  \n%14C %14C %14C  \n*VWRITE,' ','REAL','IMAGINARY'  \n%14C %14C %14C  \n*VWRITE,_P26_EXPORT(1,0),_P26_EXPORT(1,1),_P26_EXPORT(1,2)  \n%14.5G %14.5G %14.5G\n/OUTPUT,TERM\n*END\n/INPUT,scratch,gui  \n! End of time history save " ("字符串")) -> (w931:string)
        n159 = Write to Text File(file (use dialog)=w932, text=w931) -> ()  [unwired: 2 in, 3 out]
      }
      event "14": Value Change {
        n160 = event-data() -> ()  [unwired: 1 in, 6 out]
        n161 = Number To Fractional String(number="压电片外圈直径") -> (F-format string=w935:string)  [unwired: 3 in]
        n162 = Open/Create/Replace File(file path (use dialog)=path "H:/新/finaltest.dat" ("文件路径（使用对话框）"), operation (0:open)=T1."replace" ("操作(0:open)")) -> (refnum out=w940:refnum<file>)  [unwired: 4 in, 2 out]
        n163 = Concatenate Strings("/RGB,INDEX,100,100,100, 0   \n/RGB,INDEX, 80, 80, 80,13   \n/RGB,INDEX, 60, 60, 60,14   \n/RGB,INDEX, 0, 0, 0,15  \n\n/REPLOT,RESIZE  \n/CLEAR,NOSTART \nNZ=25 !齿数：\nTH=1.5 !平均齿高：\nWTH=1.5 !外侧斜齿高\nNTH=1.5 !内侧斜齿高\nWDTH=0.0 !齿外侧导角高度\nWDTL=0.0 !齿外侧导水平长度\nNDTH=0.0 !齿内侧导角高度\nNDTL=0.0 !齿内侧导水平长度\nTT=2 !齿厚：\nTW=0.1 !齿槽宽：\nITD=8 !定子齿内圈直径：\nOTD=13.3 !定子齿外圈直径：\nIAD=2.1 !轴内圈直径：\nOAD=6 !轴外圈直径：\nAT=1.6 !轴厚度\nPT=0.4 !压电片厚：\nIPD=8 !压电片内圈直径：\nOPD=" ("字符串"), w935, " !压电片外圈直径：\nEW= ITD-OAD !宽度：\nET=0.2 !厚度：\nEH=0.2 !台阶高：\nBS=4 !波数\nFK=5 !定子分块建模分块数与齿数成整数倍的关系 \n\nNZ=NZ !齿数：\nTH=TH/1000 !齿高：\nWTH=WTH/1000 !外侧斜齿高\nNTH=NTH/1000 !内侧斜齿高\nWDTH=WDTH/1000 !齿外侧导角高度\nWDTL=WDTL/1000 !齿外侧导水平长度\nNDTH=NDTH/1000 !齿内侧导角高度\nNDTL=NDTL/1000 !齿内侧导水平长度\nTT=TT/1000 !齿厚：\nTW=TW/1000 !齿槽宽：\nITD=ITD/1000 !定子齿内圈直径：\nOTD=OTD/1000 !定子齿外圈直径：\nIAD=IAD/1000 !轴内圈直径：\nOAD=OAD/1000 !轴外圈直径：\nAT=AT/1000 !轴厚度\nPT=PT/1000 !压电片厚：\nIPD=IPD/1000 !压电片内圈直径：\nOPD=OPD/1000 !压电片外圈直径：\nEW= EW/1000 !宽度：\nET=ET/1000 !厚度：\nEH=EH/1000 !台阶高：\n\n/PREP7 \n!定义单元和材料属性\nET,1,SOLID185   \nMPTEMP,,,,,,,,  \nMPTEMP,1,0  \nMPDATA,DENS,1,,8290\nMPTEMP,,,,,,,,  \nMPTEMP,1,0  \nMPDATA,EX,1,,1.06E+011   \nMPDATA,PRXY,1,,0.35 \n\nET,2,SOLID5 \nMPTEMP,,,,,,,,  \nMPTEMP,1,0     \nMPDATA,DENS,2,,7750   \nMPTEMP,,,,,,,,  \nMPTEMP,1,0  \nMPDATA,PERX,2,,919E-009\nMPDATA,PERY,2,,919E-009   \nMPDATA,PERZ,2,,826E-009\nTB,PIEZ,2,,,0   \nTBMODIF,1,1,0   \nTBMODIF,1,2,0   \nTBMODIF,1,3,-5.35   \nTBMODIF,2,1,0   \nTBMODIF,2,2,0   \nTBMODIF,2,3,-5.35   \nTBMODIF,3,1,0   \nTBMODIF,3,2,0   \nTBMODIF,3,3,15.78   \nTBMODIF,4,1,0   \nTBMODIF,4,2,0   \nTBMODIF,4,3,0   \nTBMODIF,5,1,0   \nTBMODIF,5,2,12.3\nTBMODIF,5,3,0   \nTBMODIF,6,1,12.3\nTBMODIF,6,2,0   \nTBMODIF,6,3,0   \nTB,ANEL,2,1,21,0\nTBTEMP,0\nTBDATA,,1.2035E+011,7.52E+010,7.51E+010,0,0,0   \nTBDATA,,1.204E+011,7.51E+010,0,0,0,1.109E+011   \nTBDATA,,0,0,0,2.26E+010,0,0 \nTBDATA,,2.12E+010,0,2.11E+010,,,\n\n!超声波电机模型建立\nK,1,OAD/2,,,\nK,2,ITD/2,,,\nK,3,ITD/2,-EH,,!最上面\nK,4,OTD/2,-EH,,\nK,5,OTD/2,-EH+TT-TH,,\nK,6,ITD/2,-EH+TT-TH,,\nK,7,ITD/2,ET,,\nK,8,OAD/2,ET,,\nK,11,ITD/2,-EH-PT,,!最下面\nK,12,OTD/2,-EH-PT,,\nK,13,OTD/2,-EH+TT,,\nK,14,ITD/2,-EH+TT,,\nK,15,IAD/2,ET,,\nK,16,IAD/2,0,,\nK,17,IAD/2,-AT+ET,,\nK,18,OAD/2,-AT+ET,,\n\nK,100,0,0,0,\nK,101,0,0.003,0,\n\nLSTR,1,2\nLSTR,2,3\nLSTR,3,4\nLSTR,4,5\nLSTR,5,6\nLSTR,6,7\nLSTR,7,8\nLSTR,8,1\nLSTR,3,11\nLSTR,11,12\nLSTR,12,4\nLSTR,5,13\nLSTR,13,14\nLSTR,14,6\nLSTR,2,7\nLSTR,8,15\nLSTR,15,16\nLSTR,1,16\nLSTR,16,17\nLSTR,17,18\nLSTR,1,18\n\nAL,1,15,7,8\nAL,15,2,3,4,5,6,\nAL,9,10,11,3\nAL,5,12,13,14\nAL,8,16,17,18\nAL,18,19,20,21\n\nVROTAT,1,2,3,4, , ,100,101 ,360/FK, , !!!!!\nVROTAT,5,6, , , , ,100,101 ,360/FK, , !!!!!\nBLC4,0,TT-EH,OTD,-TH,TW !建立长方体\nVGEN, ,7, , , , ,-TW/2, , ,1!复制创建体  \nVOVLAP,4,7 !布尔操作\nVDELE,10, , ,1!删除体\nVSYMM,Z,8, , , ,0,0 !体镜像 \n\n!建立齿槽\nCSYS,5  \nWPSTYLE,,,,,,,,0\nVGEN,NZ/FK+1,4, , , ,360/NZ, , ,0  \nVGEN,NZ/FK+1,8, , , ,360/NZ, , ,0  \nVOVLAP,ALL\n*DO,I,1,NZ/FK+1\nCSYS,0\nVSEL,S,LOC,Y,TT-EH-TH/1.5,1\nCSYS,5\nVSEL,R,LOC,Y,(I-1)*360/NZ-TW/2/3.1415/ITD*360,TW/2/3.1415/ITD*360+(I-1)*360/NZ!选择体\nVDELE,ALL, , ,1\nALLSEL,ALL \n*ENDDO\n\n!旋转成体\nEPLOT \nCSYS,5 \nVGEN,FK,ALL, , , ,360/FK, , ,0 \n\n!Glue体\nVGLUE,ALL\n\n!添加材料属性\nALLSEL,ALL\nCSYS,0\nVSEL,S,LOC,Y,0,TT-EH\nVATT,       1, ,   1,       0   \nCSYS,5\nVSEL,S,LOC,X,0,OAD/2\nVATT,       1, ,   1,       0 \n\nALLSEL,ALL\nCSYS,0\nVSEL,R,LOC,Y,-EH-PT,-EH\nVATT,       2, ,  2,       0  \nALLSEL,ALL\n\n!网格体\nCSYS,0\nVSEL,R,LOC,Y,-EH-PT,-EH\nVSWEEP,ALL\n\nCSYS,0\nALLSEL,ALL \nVSEL,S,MAT,,1\nSMRT,6  \nSMRT,5  \nSMRT,4  \nMSHAPE,1,3d\nMSHKEY,0\nVMESH,ALL\n\nALLSEL,ALL\n\n!模态分析 \n/SOL  \nANTYPE,2\nMODOPT,LANB,22  \nEQSLV,SPAR  \nMXPAND,0, , ,0  \nLUMPM,0 \nPSTRES,0\nMODOPT,LANB,22,0,80000, ,OFF\n\nCSYS,5\nASEL,S,LOC,X,-IAD/2,IAD/2   \nDA,ALL,ALL,\nALLSEL,ALL\n\n!OUTPR,BASIC,ALL,  \n!OUTRES,ALL,ALL,\n \n/STATUS,SOLU\nSOLVE   \nFINISH\nCSYS,0\nALLSEL,ALL\n\n/POST1  \nSET,FIRST   \n/EFACET,1   \nPLNSOL, U,SUM, 2,1.0 !无轮廓2变0\n/post1\n*do,i,8,22\nset,1,i\n/VIEW,1,1,2,3   \n/ANG,1  \n/REP,FAST  \n/show,jpeg,,\nplnsol,u,sum,0,1.0\n/show,close\n*enddo\nFINISH\n\n!振幅仿真\n/SOL\nANTYPE,3\nHROPT,FULL  \nHROUT,ON\nLUMPM,0 \nEQSLV, ,0,  \nPSTRES,0\n\n!阻尼特性\nALPHAD,0,   \nBETAD,0,\nDMPSTR,0.005,   \n\n!压电耦合\n*do,i,1,(BS-1)\nALLSEL,ALL\ncsys,5\nnsel,S,LOC,X,ITD/2,OTD/2\ncsys,0\nnsel,R,loc,y,-eh-eq-pt\ncsys,5\nangle=360/BS\nnsel,r,loc,y,(i-1)*angle/2,i*angle/2\nb=1/2*(1-(-1)**i)*1\nc=1/2*(1-(-1)**(i+1))*1\nD,All,VOLT,b,c\n*enddo\n\nALLSEL,ALL\ncsys,5\nnsel,S,LOC,X,ITD/2,OTD/2\ncsys,0\nnsel,R,loc,y,-eh-eq-pt\ncsys,5\nangle=360/BS\nnsel,r,loc,y,(BS-1)*angle/2,((BS-1)*angle/2+3*angle/8)\nD,All,VOLT,(1/2*(1-(-1)**BS)*1),(1/2*(1-(-1)**(BS+1))*1)\n\nALLSEL,ALL\ncsys,5\nnsel,S,LOC,X,ITD/2,OTD/2\ncsys,0\nnsel,R,loc,y,-eh-eq-pt\ncsys,5\nangle=360/BS\nnsel,r,loc,y,((BS-1)*angle/2+3*angle/8),((BS-1)*angle/2+3*angle/4)\nD,All,VOLT,(1/2*(1-(-1)**(BS+1))*1),(1/2*(1-(-1)**(BS+2))*1)\n\n*do,i,1,(BS-1)\nALLSEL,ALL\ncsys,5\nnsel,S,LOC,X,ITD/2,OTD/2\ncsys,0\nnsel,R,loc,y,-eh-eq-pt\ncsys,5\nangle=360/BS\nnsel,r,loc,y,((BS-1)*angle/2+3*angle/4+(i-1)*angle/2),((BS-1)*angle/2+3*angle/4+(i)*angle/2)\ne=1/2*(1-(-1)**(BS+1+i))*1\nf=1/2*(1-(-1)**(BS+2+i))*1\nD,All,VOLT,e,f\n*enddo\n\nALLSEL,ALL\ncsys,5\nnsel,S,LOC,X,ITD/2,OTD/2\ncsys,0\nnsel,r,loc,y,-eh-eq\nD,All,VOLT,0,0\nALLSEL,ALL \n\nHARFRQ,26000,76000, \nNSUBST,5,  \nKBC,1\n/STATUS,SOLU\nSOLVE\n\n!选最大位移点\n/POST1\nNSORT,U,SUM,0,1, ,SELECT  \nPRNSOL,U,Z\n*get,node,SORT,0,IMAX\n\n!结果显示,打开后处理器\n/POST26 \nFILE,'finaltest','rst','.'   \n/UI,COLL,1  \nNUMVAR,200  \nSOLU,191,NCMIT  \nSTORE,MERGE \nPLCPLX,0\nPRCPLX,1\nFILLDATA,191,,,,1,1 \nREALVAR,191,191 \n\n!z方向位移 \nNSOL,2,node,U,Z, UZ_2, \nSTORE,MERGE \n\n!保存为txt(excel也行)\n/post26\n! Save time history variables to file zmovement.prn\n*CREATE,scratch,gui \n*DEL,_P26_EXPORT\n*DIM,_P26_EXPORT,TABLE,5,2 \nVGET,_P26_EXPORT(1,0),1 \nVGET,_P26_EXPORT(1,1),2,,0  \nVGET,_P26_EXPORT(1,2),2,,1  \n/OUTPUT,'zmovement','prn','.'  \n*VWRITE,'FREQ','UZ_2',' '   \n%14C %14C %14C\n*VWRITE,' ','REAL','IMAGINARY'  \n%14C %14C %14C  \n*VWRITE,_P26_EXPORT(1,0),_P26_EXPORT(1,1),_P26_EXPORT(1,2)  \n%14.5G %14.5G %14.5G\n/OUTPUT,TERM\n*END\n/INPUT,scratch,gui  \n! End of time history save  \n\n!x方向位移 \nNSOL,3,node,U,X, UX_3, \nSTORE,MERGE \n\n!保存为txt(excel也行)\n/post26\n! Save time history variables to file xmovement.prn\n*CREATE,scratch,gui \n*DEL,_P26_EXPORT\n*DIM,_P26_EXPORT,TABLE,5,2 \nVGET,_P26_EXPORT(1,0),1 \nVGET,_P26_EXPORT(1,1),3,,0  \nVGET,_P26_EXPORT(1,2),3,,1  \n/OUTPUT,'xmovement','prn','.'  \n*VWRITE,'FREQ','UX_3',' '   \n%14C %14C %14C  \n*VWRITE,' ','REAL','IMAGINARY'  \n%14C %14C %14C  \n*VWRITE,_P26_EXPORT(1,0),_P26_EXPORT(1,1),_P26_EXPORT(1,2)  \n%14.5G %14.5G %14.5G\n/OUTPUT,TERM\n*END\n/INPUT,scratch,gui  \n! End of time history save\n\n!y方向位移 \nNSOL,4,node,U,Y, UY_4, \nSTORE,MERGE \n\n!保存为txt(excel也行)\n/post26\n! Save time history variables to file ymovement.prn\n*CREATE,scratch,gui \n*DEL,_P26_EXPORT\n*DIM,_P26_EXPORT,TABLE,5,2 \nVGET,_P26_EXPORT(1,0),1 \nVGET,_P26_EXPORT(1,1),4,,0  \nVGET,_P26_EXPORT(1,2),4,,1  \n/OUTPUT,'ymovement','prn','.'  \n*VWRITE,'FREQ','UY_4',' '   \n%14C %14C %14C  \n*VWRITE,' ','REAL','IMAGINARY'  \n%14C %14C %14C  \n*VWRITE,_P26_EXPORT(1,0),_P26_EXPORT(1,1),_P26_EXPORT(1,2)  \n%14.5G %14.5G %14.5G\n/OUTPUT,TERM\n*END\n/INPUT,scratch,gui  \n! End of time history save\n\n!选择电流点\nRFORCE,2,180,AMPS,, AMPS_2  \nSTORE,MERGE \nFILLDATA,192,,,,0,0 \nFILLDATA,193,,,,1,0 \nFILLDATA,194,,,,-1,0\nFILLDATA,195,,,,1,1 \nVARNAME,195,NSET\n! Name: Z   \n! ID:  3\n! Function: 1/{AMPS_2}  \nFILLDATA,199,,,,1,0 \nREALVAR,199,199 \nQUOT,3,199,2,,Z \nSTORE,MERGE \n\n!保存为txt(excel也行)\n/post26\n! Save time history variables to file current.prn   \n*CREATE,scratch,gui \n*DEL,_P26_EXPORT\n*DIM,_P26_EXPORT,TABLE,5,2 \nVGET,_P26_EXPORT(1,0),1 \nVGET,_P26_EXPORT(1,1),3,,0  \nVGET,_P26_EXPORT(1,2),3,,1  \n/OUTPUT,'current','prn','.' \n*VWRITE,'FREQ','Z',' '  \n%14C %14C %14C  \n*VWRITE,' ','REAL','IMAGINARY'  \n%14C %14C %14C  \n*VWRITE,_P26_EXPORT(1,0),_P26_EXPORT(1,1),_P26_EXPORT(1,2)  \n%14.5G %14.5G %14.5G\n/OUTPUT,TERM\n*END\n/INPUT,scratch,gui  \n! End of time history save " ("字符串")) -> (w939:string)
        n164 = Write to Text File(file (use dialog)=w940, text=w939) -> ()  [unwired: 2 in, 3 out]
      }
      event "15": Value Change {
        n165 = event-data() -> ()  [unwired: 1 in, 6 out]
        n166 = Number To Fractional String(number="台阶高") -> (F-format string=w943:string)  [unwired: 3 in]
        n167 = Open/Create/Replace File(file path (use dialog)=path "H:/新/finaltest.dat" ("文件路径（使用对话框）"), operation (0:open)=T1."replace" ("操作(0:open)")) -> (refnum out=w948:refnum<file>)  [unwired: 4 in, 2 out]
        n168 = Concatenate Strings("/RGB,INDEX,100,100,100, 0   \n/RGB,INDEX, 80, 80, 80,13   \n/RGB,INDEX, 60, 60, 60,14   \n/RGB,INDEX, 0, 0, 0,15  \n\n/REPLOT,RESIZE  \n/CLEAR,NOSTART \nNZ=25 !齿数：\nTH=1.5 !平均齿高：\nWTH=1.5 !外侧斜齿高\nNTH=1.5 !内侧斜齿高\nWDTH=0.0 !齿外侧导角高度\nWDTL=0.0 !齿外侧导水平长度\nNDTH=0.0 !齿内侧导角高度\nNDTL=0.0 !齿内侧导水平长度\nTT=2 !齿厚：\nTW=0.1 !齿槽宽：\nITD=8 !定子齿内圈直径：\nOTD=13.3 !定子齿外圈直径：\nIAD=2.1 !轴内圈直径：\nOAD=6 !轴外圈直径：\nAT=1.6 !轴厚度\nPT=0.4 !压电片厚：\nIPD=8 !压电片内圈直径：\nOPD=13.3 !压电片外圈直径：\nEW= ITD-OAD !宽度：\nET=0.2 !厚度：\nEH=" ("字符串"), w943, " !台阶高：\nBS=4 !波数\nFK=5 !定子分块建模分块数与齿数成整数倍的关系 \n\nNZ=NZ !齿数：\nTH=TH/1000 !齿高：\nWTH=WTH/1000 !外侧斜齿高\nNTH=NTH/1000 !内侧斜齿高\nWDTH=WDTH/1000 !齿外侧导角高度\nWDTL=WDTL/1000 !齿外侧导水平长度\nNDTH=NDTH/1000 !齿内侧导角高度\nNDTL=NDTL/1000 !齿内侧导水平长度\nTT=TT/1000 !齿厚：\nTW=TW/1000 !齿槽宽：\nITD=ITD/1000 !定子齿内圈直径：\nOTD=OTD/1000 !定子齿外圈直径：\nIAD=IAD/1000 !轴内圈直径：\nOAD=OAD/1000 !轴外圈直径：\nAT=AT/1000 !轴厚度\nPT=PT/1000 !压电片厚：\nIPD=IPD/1000 !压电片内圈直径：\nOPD=OPD/1000 !压电片外圈直径：\nEW= EW/1000 !宽度：\nET=ET/1000 !厚度：\nEH=EH/1000 !台阶高：\n\n/PREP7 \n!定义单元和材料属性\nET,1,SOLID185   \nMPTEMP,,,,,,,,  \nMPTEMP,1,0  \nMPDATA,DENS,1,,8290\nMPTEMP,,,,,,,,  \nMPTEMP,1,0  \nMPDATA,EX,1,,1.06E+011   \nMPDATA,PRXY,1,,0.35 \n\nET,2,SOLID5 \nMPTEMP,,,,,,,,  \nMPTEMP,1,0     \nMPDATA,DENS,2,,7750   \nMPTEMP,,,,,,,,  \nMPTEMP,1,0  \nMPDATA,PERX,2,,919E-009\nMPDATA,PERY,2,,919E-009   \nMPDATA,PERZ,2,,826E-009\nTB,PIEZ,2,,,0   \nTBMODIF,1,1,0   \nTBMODIF,1,2,0   \nTBMODIF,1,3,-5.35   \nTBMODIF,2,1,0   \nTBMODIF,2,2,0   \nTBMODIF,2,3,-5.35   \nTBMODIF,3,1,0   \nTBMODIF,3,2,0   \nTBMODIF,3,3,15.78   \nTBMODIF,4,1,0   \nTBMODIF,4,2,0   \nTBMODIF,4,3,0   \nTBMODIF,5,1,0   \nTBMODIF,5,2,12.3\nTBMODIF,5,3,0   \nTBMODIF,6,1,12.3\nTBMODIF,6,2,0   \nTBMODIF,6,3,0   \nTB,ANEL,2,1,21,0\nTBTEMP,0\nTBDATA,,1.2035E+011,7.52E+010,7.51E+010,0,0,0   \nTBDATA,,1.204E+011,7.51E+010,0,0,0,1.109E+011   \nTBDATA,,0,0,0,2.26E+010,0,0 \nTBDATA,,2.12E+010,0,2.11E+010,,,\n\n!超声波电机模型建立\nK,1,OAD/2,,,\nK,2,ITD/2,,,\nK,3,ITD/2,-EH,,!最上面\nK,4,OTD/2,-EH,,\nK,5,OTD/2,-EH+TT-TH,,\nK,6,ITD/2,-EH+TT-TH,,\nK,7,ITD/2,ET,,\nK,8,OAD/2,ET,,\nK,11,ITD/2,-EH-PT,,!最下面\nK,12,OTD/2,-EH-PT,,\nK,13,OTD/2,-EH+TT,,\nK,14,ITD/2,-EH+TT,,\nK,15,IAD/2,ET,,\nK,16,IAD/2,0,,\nK,17,IAD/2,-AT+ET,,\nK,18,OAD/2,-AT+ET,,\n\nK,100,0,0,0,\nK,101,0,0.003,0,\n\nLSTR,1,2\nLSTR,2,3\nLSTR,3,4\nLSTR,4,5\nLSTR,5,6\nLSTR,6,7\nLSTR,7,8\nLSTR,8,1\nLSTR,3,11\nLSTR,11,12\nLSTR,12,4\nLSTR,5,13\nLSTR,13,14\nLSTR,14,6\nLSTR,2,7\nLSTR,8,15\nLSTR,15,16\nLSTR,1,16\nLSTR,16,17\nLSTR,17,18\nLSTR,1,18\n\nAL,1,15,7,8\nAL,15,2,3,4,5,6,\nAL,9,10,11,3\nAL,5,12,13,14\nAL,8,16,17,18\nAL,18,19,20,21\n\nVROTAT,1,2,3,4, , ,100,101 ,360/FK, , !!!!!\nVROTAT,5,6, , , , ,100,101 ,360/FK, , !!!!!\nBLC4,0,TT-EH,OTD,-TH,TW !建立长方体\nVGEN, ,7, , , , ,-TW/2, , ,1!复制创建体  \nVOVLAP,4,7 !布尔操作\nVDELE,10, , ,1!删除体\nVSYMM,Z,8, , , ,0,0 !体镜像 \n\n!建立齿槽\nCSYS,5  \nWPSTYLE,,,,,,,,0\nVGEN,NZ/FK+1,4, , , ,360/NZ, , ,0  \nVGEN,NZ/FK+1,8, , , ,360/NZ, , ,0  \nVOVLAP,ALL\n*DO,I,1,NZ/FK+1\nCSYS,0\nVSEL,S,LOC,Y,TT-EH-TH/1.5,1\nCSYS,5\nVSEL,R,LOC,Y,(I-1)*360/NZ-TW/2/3.1415/ITD*360,TW/2/3.1415/ITD*360+(I-1)*360/NZ!选择体\nVDELE,ALL, , ,1\nALLSEL,ALL \n*ENDDO\n\n!旋转成体\nEPLOT \nCSYS,5 \nVGEN,FK,ALL, , , ,360/FK, , ,0 \n\n!Glue体\nVGLUE,ALL\n\n!添加材料属性\nALLSEL,ALL\nCSYS,0\nVSEL,S,LOC,Y,0,TT-EH\nVATT,       1, ,   1,       0   \nCSYS,5\nVSEL,S,LOC,X,0,OAD/2\nVATT,       1, ,   1,       0 \n\nALLSEL,ALL\nCSYS,0\nVSEL,R,LOC,Y,-EH-PT,-EH\nVATT,       2, ,  2,       0  \nALLSEL,ALL\n\n!网格体\nCSYS,0\nVSEL,R,LOC,Y,-EH-PT,-EH\nVSWEEP,ALL\n\nCSYS,0\nALLSEL,ALL \nVSEL,S,MAT,,1\nSMRT,6  \nSMRT,5  \nSMRT,4  \nMSHAPE,1,3d\nMSHKEY,0\nVMESH,ALL\n\nALLSEL,ALL\n\n!模态分析 \n/SOL  \nANTYPE,2\nMODOPT,LANB,22  \nEQSLV,SPAR  \nMXPAND,0, , ,0  \nLUMPM,0 \nPSTRES,0\nMODOPT,LANB,22,0,80000, ,OFF\n\nCSYS,5\nASEL,S,LOC,X,-IAD/2,IAD/2   \nDA,ALL,ALL,\nALLSEL,ALL\n\n!OUTPR,BASIC,ALL,  \n!OUTRES,ALL,ALL,\n \n/STATUS,SOLU\nSOLVE   \nFINISH\nCSYS,0\nALLSEL,ALL\n\n/POST1  \nSET,FIRST   \n/EFACET,1   \nPLNSOL, U,SUM, 2,1.0 !无轮廓2变0\n/post1\n*do,i,8,22\nset,1,i\n/VIEW,1,1,2,3   \n/ANG,1  \n/REP,FAST  \n/show,jpeg,,\nplnsol,u,sum,0,1.0\n/show,close\n*enddo\nFINISH\n\n!振幅仿真\n/SOL\nANTYPE,3\nHROPT,FULL  \nHROUT,ON\nLUMPM,0 \nEQSLV, ,0,  \nPSTRES,0\n\n!阻尼特性\nALPHAD,0,   \nBETAD,0,\nDMPSTR,0.005,   \n\n!压电耦合\n*do,i,1,(BS-1)\nALLSEL,ALL\ncsys,5\nnsel,S,LOC,X,ITD/2,OTD/2\ncsys,0\nnsel,R,loc,y,-eh-eq-pt\ncsys,5\nangle=360/BS\nnsel,r,loc,y,(i-1)*angle/2,i*angle/2\nb=1/2*(1-(-1)**i)*1\nc=1/2*(1-(-1)**(i+1))*1\nD,All,VOLT,b,c\n*enddo\n\nALLSEL,ALL\ncsys,5\nnsel,S,LOC,X,ITD/2,OTD/2\ncsys,0\nnsel,R,loc,y,-eh-eq-pt\ncsys,5\nangle=360/BS\nnsel,r,loc,y,(BS-1)*angle/2,((BS-1)*angle/2+3*angle/8)\nD,All,VOLT,(1/2*(1-(-1)**BS)*1),(1/2*(1-(-1)**(BS+1))*1)\n\nALLSEL,ALL\ncsys,5\nnsel,S,LOC,X,ITD/2,OTD/2\ncsys,0\nnsel,R,loc,y,-eh-eq-pt\ncsys,5\nangle=360/BS\nnsel,r,loc,y,((BS-1)*angle/2+3*angle/8),((BS-1)*angle/2+3*angle/4)\nD,All,VOLT,(1/2*(1-(-1)**(BS+1))*1),(1/2*(1-(-1)**(BS+2))*1)\n\n*do,i,1,(BS-1)\nALLSEL,ALL\ncsys,5\nnsel,S,LOC,X,ITD/2,OTD/2\ncsys,0\nnsel,R,loc,y,-eh-eq-pt\ncsys,5\nangle=360/BS\nnsel,r,loc,y,((BS-1)*angle/2+3*angle/4+(i-1)*angle/2),((BS-1)*angle/2+3*angle/4+(i)*angle/2)\ne=1/2*(1-(-1)**(BS+1+i))*1\nf=1/2*(1-(-1)**(BS+2+i))*1\nD,All,VOLT,e,f\n*enddo\n\nALLSEL,ALL\ncsys,5\nnsel,S,LOC,X,ITD/2,OTD/2\ncsys,0\nnsel,r,loc,y,-eh-eq\nD,All,VOLT,0,0\nALLSEL,ALL \n\nHARFRQ,26000,76000, \nNSUBST,5,  \nKBC,1\n/STATUS,SOLU\nSOLVE\n\n!选最大位移点\n/POST1\nNSORT,U,SUM,0,1, ,SELECT  \nPRNSOL,U,Z\n*get,node,SORT,0,IMAX\n\n!结果显示,打开后处理器\n/POST26 \nFILE,'finaltest','rst','.'   \n/UI,COLL,1  \nNUMVAR,200  \nSOLU,191,NCMIT  \nSTORE,MERGE \nPLCPLX,0\nPRCPLX,1\nFILLDATA,191,,,,1,1 \nREALVAR,191,191 \n\n!z方向位移 \nNSOL,2,node,U,Z, UZ_2, \nSTORE,MERGE \n\n!保存为txt(excel也行)\n/post26\n! Save time history variables to file zmovement.prn\n*CREATE,scratch,gui \n*DEL,_P26_EXPORT\n*DIM,_P26_EXPORT,TABLE,5,2 \nVGET,_P26_EXPORT(1,0),1 \nVGET,_P26_EXPORT(1,1),2,,0  \nVGET,_P26_EXPORT(1,2),2,,1  \n/OUTPUT,'zmovement','prn','.'  \n*VWRITE,'FREQ','UZ_2',' '   \n%14C %14C %14C\n*VWRITE,' ','REAL','IMAGINARY'  \n%14C %14C %14C  \n*VWRITE,_P26_EXPORT(1,0),_P26_EXPORT(1,1),_P26_EXPORT(1,2)  \n%14.5G %14.5G %14.5G\n/OUTPUT,TERM\n*END\n/INPUT,scratch,gui  \n! End of time history save  \n\n!x方向位移 \nNSOL,3,node,U,X, UX_3, \nSTORE,MERGE \n\n!保存为txt(excel也行)\n/post26\n! Save time history variables to file xmovement.prn\n*CREATE,scratch,gui \n*DEL,_P26_EXPORT\n*DIM,_P26_EXPORT,TABLE,5,2 \nVGET,_P26_EXPORT(1,0),1 \nVGET,_P26_EXPORT(1,1),3,,0  \nVGET,_P26_EXPORT(1,2),3,,1  \n/OUTPUT,'xmovement','prn','.'  \n*VWRITE,'FREQ','UX_3',' '   \n%14C %14C %14C  \n*VWRITE,' ','REAL','IMAGINARY'  \n%14C %14C %14C  \n*VWRITE,_P26_EXPORT(1,0),_P26_EXPORT(1,1),_P26_EXPORT(1,2)  \n%14.5G %14.5G %14.5G\n/OUTPUT,TERM\n*END\n/INPUT,scratch,gui  \n! End of time history save\n\n!y方向位移 \nNSOL,4,node,U,Y, UY_4, \nSTORE,MERGE \n\n!保存为txt(excel也行)\n/post26\n! Save time history variables to file ymovement.prn\n*CREATE,scratch,gui \n*DEL,_P26_EXPORT\n*DIM,_P26_EXPORT,TABLE,5,2 \nVGET,_P26_EXPORT(1,0),1 \nVGET,_P26_EXPORT(1,1),4,,0  \nVGET,_P26_EXPORT(1,2),4,,1  \n/OUTPUT,'ymovement','prn','.'  \n*VWRITE,'FREQ','UY_4',' '   \n%14C %14C %14C  \n*VWRITE,' ','REAL','IMAGINARY'  \n%14C %14C %14C  \n*VWRITE,_P26_EXPORT(1,0),_P26_EXPORT(1,1),_P26_EXPORT(1,2)  \n%14.5G %14.5G %14.5G\n/OUTPUT,TERM\n*END\n/INPUT,scratch,gui  \n! End of time history save\n\n!选择电流点\nRFORCE,2,180,AMPS,, AMPS_2  \nSTORE,MERGE \nFILLDATA,192,,,,0,0 \nFILLDATA,193,,,,1,0 \nFILLDATA,194,,,,-1,0\nFILLDATA,195,,,,1,1 \nVARNAME,195,NSET\n! Name: Z   \n! ID:  3\n! Function: 1/{AMPS_2}  \nFILLDATA,199,,,,1,0 \nREALVAR,199,199 \nQUOT,3,199,2,,Z \nSTORE,MERGE \n\n!保存为txt(excel也行)\n/post26\n! Save time history variables to file current.prn   \n*CREATE,scratch,gui \n*DEL,_P26_EXPORT\n*DIM,_P26_EXPORT,TABLE,5,2 \nVGET,_P26_EXPORT(1,0),1 \nVGET,_P26_EXPORT(1,1),3,,0  \nVGET,_P26_EXPORT(1,2),3,,1  \n/OUTPUT,'current','prn','.' \n*VWRITE,'FREQ','Z',' '  \n%14C %14C %14C  \n*VWRITE,' ','REAL','IMAGINARY'  \n%14C %14C %14C  \n*VWRITE,_P26_EXPORT(1,0),_P26_EXPORT(1,1),_P26_EXPORT(1,2)  \n%14.5G %14.5G %14.5G\n/OUTPUT,TERM\n*END\n/INPUT,scratch,gui  \n! End of time history save " ("字符串")) -> (w947:string)
        n169 = Write to Text File(file (use dialog)=w948, text=w947) -> ()  [unwired: 2 in, 3 out]
      }
      event "16": Value Change {
        n170 = event-data() -> ()  [unwired: 1 in, 6 out]
        n171 = Number To Fractional String(number="波数") -> (F-format string=w951:string)  [unwired: 3 in]
        n172 = Open/Create/Replace File(file path (use dialog)=path "H:/新/finaltest.dat" ("文件路径（使用对话框）"), operation (0:open)=T1."replace" ("操作(0:open)")) -> (refnum out=w956:refnum<file>)  [unwired: 4 in, 2 out]
        n173 = Concatenate Strings("/RGB,INDEX,100,100,100, 0   \n/RGB,INDEX, 80, 80, 80,13   \n/RGB,INDEX, 60, 60, 60,14   \n/RGB,INDEX, 0, 0, 0,15  \n\n/REPLOT,RESIZE  \n/CLEAR,NOSTART \nNZ=25 !齿数：\nTH=1.5 !平均齿高：\nWTH=1.5 !外侧斜齿高\nNTH=1.5 !内侧斜齿高\nWDTH=0.0 !齿外侧导角高度\nWDTL=0.0 !齿外侧导水平长度\nNDTH=0.0 !齿内侧导角高度\nNDTL=0.0 !齿内侧导水平长度\nTT=2 !齿厚：\nTW=0.1 !齿槽宽：\nITD=8 !定子齿内圈直径：\nOTD=13.3 !定子齿外圈直径：\nIAD=2.1 !轴内圈直径：\nOAD=6 !轴外圈直径：\nAT=1.6 !轴厚度\nPT=0.4 !压电片厚：\nIPD=8 !压电片内圈直径：\nOPD=13.3 !压电片外圈直径：\nEW= ITD-OAD !宽度：\nET=0.2 !厚度：\nEH=0.2 !台阶高：\nBS=" ("字符串"), w951, " !波数\nFK=5 !定子分块建模分块数与齿数成整数倍的关系 \n\nNZ=NZ !齿数：\nTH=TH/1000 !齿高：\nWTH=WTH/1000 !外侧斜齿高\nNTH=NTH/1000 !内侧斜齿高\nWDTH=WDTH/1000 !齿外侧导角高度\nWDTL=WDTL/1000 !齿外侧导水平长度\nNDTH=NDTH/1000 !齿内侧导角高度\nNDTL=NDTL/1000 !齿内侧导水平长度\nTT=TT/1000 !齿厚：\nTW=TW/1000 !齿槽宽：\nITD=ITD/1000 !定子齿内圈直径：\nOTD=OTD/1000 !定子齿外圈直径：\nIAD=IAD/1000 !轴内圈直径：\nOAD=OAD/1000 !轴外圈直径：\nAT=AT/1000 !轴厚度\nPT=PT/1000 !压电片厚：\nIPD=IPD/1000 !压电片内圈直径：\nOPD=OPD/1000 !压电片外圈直径：\nEW= EW/1000 !宽度：\nET=ET/1000 !厚度：\nEH=EH/1000 !台阶高：\n\n/PREP7 \n!定义单元和材料属性\nET,1,SOLID185   \nMPTEMP,,,,,,,,  \nMPTEMP,1,0  \nMPDATA,DENS,1,,8290\nMPTEMP,,,,,,,,  \nMPTEMP,1,0  \nMPDATA,EX,1,,1.06E+011   \nMPDATA,PRXY,1,,0.35 \n\nET,2,SOLID5 \nMPTEMP,,,,,,,,  \nMPTEMP,1,0     \nMPDATA,DENS,2,,7750   \nMPTEMP,,,,,,,,  \nMPTEMP,1,0  \nMPDATA,PERX,2,,919E-009\nMPDATA,PERY,2,,919E-009   \nMPDATA,PERZ,2,,826E-009\nTB,PIEZ,2,,,0   \nTBMODIF,1,1,0   \nTBMODIF,1,2,0   \nTBMODIF,1,3,-5.35   \nTBMODIF,2,1,0   \nTBMODIF,2,2,0   \nTBMODIF,2,3,-5.35   \nTBMODIF,3,1,0   \nTBMODIF,3,2,0   \nTBMODIF,3,3,15.78   \nTBMODIF,4,1,0   \nTBMODIF,4,2,0   \nTBMODIF,4,3,0   \nTBMODIF,5,1,0   \nTBMODIF,5,2,12.3\nTBMODIF,5,3,0   \nTBMODIF,6,1,12.3\nTBMODIF,6,2,0   \nTBMODIF,6,3,0   \nTB,ANEL,2,1,21,0\nTBTEMP,0\nTBDATA,,1.2035E+011,7.52E+010,7.51E+010,0,0,0   \nTBDATA,,1.204E+011,7.51E+010,0,0,0,1.109E+011   \nTBDATA,,0,0,0,2.26E+010,0,0 \nTBDATA,,2.12E+010,0,2.11E+010,,,\n\n!超声波电机模型建立\nK,1,OAD/2,,,\nK,2,ITD/2,,,\nK,3,ITD/2,-EH,,!最上面\nK,4,OTD/2,-EH,,\nK,5,OTD/2,-EH+TT-TH,,\nK,6,ITD/2,-EH+TT-TH,,\nK,7,ITD/2,ET,,\nK,8,OAD/2,ET,,\nK,11,ITD/2,-EH-PT,,!最下面\nK,12,OTD/2,-EH-PT,,\nK,13,OTD/2,-EH+TT,,\nK,14,ITD/2,-EH+TT,,\nK,15,IAD/2,ET,,\nK,16,IAD/2,0,,\nK,17,IAD/2,-AT+ET,,\nK,18,OAD/2,-AT+ET,,\n\nK,100,0,0,0,\nK,101,0,0.003,0,\n\nLSTR,1,2\nLSTR,2,3\nLSTR,3,4\nLSTR,4,5\nLSTR,5,6\nLSTR,6,7\nLSTR,7,8\nLSTR,8,1\nLSTR,3,11\nLSTR,11,12\nLSTR,12,4\nLSTR,5,13\nLSTR,13,14\nLSTR,14,6\nLSTR,2,7\nLSTR,8,15\nLSTR,15,16\nLSTR,1,16\nLSTR,16,17\nLSTR,17,18\nLSTR,1,18\n\nAL,1,15,7,8\nAL,15,2,3,4,5,6,\nAL,9,10,11,3\nAL,5,12,13,14\nAL,8,16,17,18\nAL,18,19,20,21\n\nVROTAT,1,2,3,4, , ,100,101 ,360/FK, , !!!!!\nVROTAT,5,6, , , , ,100,101 ,360/FK, , !!!!!\nBLC4,0,TT-EH,OTD,-TH,TW !建立长方体\nVGEN, ,7, , , , ,-TW/2, , ,1!复制创建体  \nVOVLAP,4,7 !布尔操作\nVDELE,10, , ,1!删除体\nVSYMM,Z,8, , , ,0,0 !体镜像 \n\n!建立齿槽\nCSYS,5  \nWPSTYLE,,,,,,,,0\nVGEN,NZ/FK+1,4, , , ,360/NZ, , ,0  \nVGEN,NZ/FK+1,8, , , ,360/NZ, , ,0  \nVOVLAP,ALL\n*DO,I,1,NZ/FK+1\nCSYS,0\nVSEL,S,LOC,Y,TT-EH-TH/1.5,1\nCSYS,5\nVSEL,R,LOC,Y,(I-1)*360/NZ-TW/2/3.1415/ITD*360,TW/2/3.1415/ITD*360+(I-1)*360/NZ!选择体\nVDELE,ALL, , ,1\nALLSEL,ALL \n*ENDDO\n\n!旋转成体\nEPLOT \nCSYS,5 \nVGEN,FK,ALL, , , ,360/FK, , ,0 \n\n!Glue体\nVGLUE,ALL\n\n!添加材料属性\nALLSEL,ALL\nCSYS,0\nVSEL,S,LOC,Y,0,TT-EH\nVATT,       1, ,   1,       0   \nCSYS,5\nVSEL,S,LOC,X,0,OAD/2\nVATT,       1, ,   1,       0 \n\nALLSEL,ALL\nCSYS,0\nVSEL,R,LOC,Y,-EH-PT,-EH\nVATT,       2, ,  2,       0  \nALLSEL,ALL\n\n!网格体\nCSYS,0\nVSEL,R,LOC,Y,-EH-PT,-EH\nVSWEEP,ALL\n\nCSYS,0\nALLSEL,ALL \nVSEL,S,MAT,,1\nSMRT,6  \nSMRT,5  \nSMRT,4  \nMSHAPE,1,3d\nMSHKEY,0\nVMESH,ALL\n\nALLSEL,ALL\n\n!模态分析 \n/SOL  \nANTYPE,2\nMODOPT,LANB,22  \nEQSLV,SPAR  \nMXPAND,0, , ,0  \nLUMPM,0 \nPSTRES,0\nMODOPT,LANB,22,0,80000, ,OFF\n\nCSYS,5\nASEL,S,LOC,X,-IAD/2,IAD/2   \nDA,ALL,ALL,\nALLSEL,ALL\n\n!OUTPR,BASIC,ALL,  \n!OUTRES,ALL,ALL,\n \n/STATUS,SOLU\nSOLVE   \nFINISH\nCSYS,0\nALLSEL,ALL\n\n/POST1  \nSET,FIRST   \n/EFACET,1   \nPLNSOL, U,SUM, 2,1.0 !无轮廓2变0\n/post1\n*do,i,8,22\nset,1,i\n/VIEW,1,1,2,3   \n/ANG,1  \n/REP,FAST  \n/show,jpeg,,\nplnsol,u,sum,0,1.0\n/show,close\n*enddo\nFINISH\n\n!振幅仿真\n/SOL\nANTYPE,3\nHROPT,FULL  \nHROUT,ON\nLUMPM,0 \nEQSLV, ,0,  \nPSTRES,0\n\n!阻尼特性\nALPHAD,0,   \nBETAD,0,\nDMPSTR,0.005,   \n\n!压电耦合\n*do,i,1,(BS-1)\nALLSEL,ALL\ncsys,5\nnsel,S,LOC,X,ITD/2,OTD/2\ncsys,0\nnsel,R,loc,y,-eh-eq-pt\ncsys,5\nangle=360/BS\nnsel,r,loc,y,(i-1)*angle/2,i*angle/2\nb=1/2*(1-(-1)**i)*1\nc=1/2*(1-(-1)**(i+1))*1\nD,All,VOLT,b,c\n*enddo\n\nALLSEL,ALL\ncsys,5\nnsel,S,LOC,X,ITD/2,OTD/2\ncsys,0\nnsel,R,loc,y,-eh-eq-pt\ncsys,5\nangle=360/BS\nnsel,r,loc,y,(BS-1)*angle/2,((BS-1)*angle/2+3*angle/8)\nD,All,VOLT,(1/2*(1-(-1)**BS)*1),(1/2*(1-(-1)**(BS+1))*1)\n\nALLSEL,ALL\ncsys,5\nnsel,S,LOC,X,ITD/2,OTD/2\ncsys,0\nnsel,R,loc,y,-eh-eq-pt\ncsys,5\nangle=360/BS\nnsel,r,loc,y,((BS-1)*angle/2+3*angle/8),((BS-1)*angle/2+3*angle/4)\nD,All,VOLT,(1/2*(1-(-1)**(BS+1))*1),(1/2*(1-(-1)**(BS+2))*1)\n\n*do,i,1,(BS-1)\nALLSEL,ALL\ncsys,5\nnsel,S,LOC,X,ITD/2,OTD/2\ncsys,0\nnsel,R,loc,y,-eh-eq-pt\ncsys,5\nangle=360/BS\nnsel,r,loc,y,((BS-1)*angle/2+3*angle/4+(i-1)*angle/2),((BS-1)*angle/2+3*angle/4+(i)*angle/2)\ne=1/2*(1-(-1)**(BS+1+i))*1\nf=1/2*(1-(-1)**(BS+2+i))*1\nD,All,VOLT,e,f\n*enddo\n\nALLSEL,ALL\ncsys,5\nnsel,S,LOC,X,ITD/2,OTD/2\ncsys,0\nnsel,r,loc,y,-eh-eq\nD,All,VOLT,0,0\nALLSEL,ALL \n\nHARFRQ,26000,76000, \nNSUBST,5,  \nKBC,1\n/STATUS,SOLU\nSOLVE\n\n!选最大位移点\n/POST1\nNSORT,U,SUM,0,1, ,SELECT  \nPRNSOL,U,Z\n*get,node,SORT,0,IMAX\n\n!结果显示,打开后处理器\n/POST26 \nFILE,'finaltest','rst','.'   \n/UI,COLL,1  \nNUMVAR,200  \nSOLU,191,NCMIT  \nSTORE,MERGE \nPLCPLX,0\nPRCPLX,1\nFILLDATA,191,,,,1,1 \nREALVAR,191,191 \n\n!z方向位移 \nNSOL,2,node,U,Z, UZ_2, \nSTORE,MERGE \n\n!保存为txt(excel也行)\n/post26\n! Save time history variables to file zmovement.prn\n*CREATE,scratch,gui \n*DEL,_P26_EXPORT\n*DIM,_P26_EXPORT,TABLE,5,2 \nVGET,_P26_EXPORT(1,0),1 \nVGET,_P26_EXPORT(1,1),2,,0  \nVGET,_P26_EXPORT(1,2),2,,1  \n/OUTPUT,'zmovement','prn','.'  \n*VWRITE,'FREQ','UZ_2',' '   \n%14C %14C %14C\n*VWRITE,' ','REAL','IMAGINARY'  \n%14C %14C %14C  \n*VWRITE,_P26_EXPORT(1,0),_P26_EXPORT(1,1),_P26_EXPORT(1,2)  \n%14.5G %14.5G %14.5G\n/OUTPUT,TERM\n*END\n/INPUT,scratch,gui  \n! End of time history save  \n\n!x方向位移 \nNSOL,3,node,U,X, UX_3, \nSTORE,MERGE \n\n!保存为txt(excel也行)\n/post26\n! Save time history variables to file xmovement.prn\n*CREATE,scratch,gui \n*DEL,_P26_EXPORT\n*DIM,_P26_EXPORT,TABLE,5,2 \nVGET,_P26_EXPORT(1,0),1 \nVGET,_P26_EXPORT(1,1),3,,0  \nVGET,_P26_EXPORT(1,2),3,,1  \n/OUTPUT,'xmovement','prn','.'  \n*VWRITE,'FREQ','UX_3',' '   \n%14C %14C %14C  \n*VWRITE,' ','REAL','IMAGINARY'  \n%14C %14C %14C  \n*VWRITE,_P26_EXPORT(1,0),_P26_EXPORT(1,1),_P26_EXPORT(1,2)  \n%14.5G %14.5G %14.5G\n/OUTPUT,TERM\n*END\n/INPUT,scratch,gui  \n! End of time history save\n\n!y方向位移 \nNSOL,4,node,U,Y, UY_4, \nSTORE,MERGE \n\n!保存为txt(excel也行)\n/post26\n! Save time history variables to file ymovement.prn\n*CREATE,scratch,gui \n*DEL,_P26_EXPORT\n*DIM,_P26_EXPORT,TABLE,5,2 \nVGET,_P26_EXPORT(1,0),1 \nVGET,_P26_EXPORT(1,1),4,,0  \nVGET,_P26_EXPORT(1,2),4,,1  \n/OUTPUT,'ymovement','prn','.'  \n*VWRITE,'FREQ','UY_4',' '   \n%14C %14C %14C  \n*VWRITE,' ','REAL','IMAGINARY'  \n%14C %14C %14C  \n*VWRITE,_P26_EXPORT(1,0),_P26_EXPORT(1,1),_P26_EXPORT(1,2)  \n%14.5G %14.5G %14.5G\n/OUTPUT,TERM\n*END\n/INPUT,scratch,gui  \n! End of time history save\n\n!选择电流点\nRFORCE,2,180,AMPS,, AMPS_2  \nSTORE,MERGE \nFILLDATA,192,,,,0,0 \nFILLDATA,193,,,,1,0 \nFILLDATA,194,,,,-1,0\nFILLDATA,195,,,,1,1 \nVARNAME,195,NSET\n! Name: Z   \n! ID:  3\n! Function: 1/{AMPS_2}  \nFILLDATA,199,,,,1,0 \nREALVAR,199,199 \nQUOT,3,199,2,,Z \nSTORE,MERGE \n\n!保存为txt(excel也行)\n/post26\n! Save time history variables to file current.prn   \n*CREATE,scratch,gui \n*DEL,_P26_EXPORT\n*DIM,_P26_EXPORT,TABLE,5,2 \nVGET,_P26_EXPORT(1,0),1 \nVGET,_P26_EXPORT(1,1),3,,0  \nVGET,_P26_EXPORT(1,2),3,,1  \n/OUTPUT,'current','prn','.' \n*VWRITE,'FREQ','Z',' '  \n%14C %14C %14C  \n*VWRITE,' ','REAL','IMAGINARY'  \n%14C %14C %14C  \n*VWRITE,_P26_EXPORT(1,0),_P26_EXPORT(1,1),_P26_EXPORT(1,2)  \n%14.5G %14.5G %14.5G\n/OUTPUT,TERM\n*END\n/INPUT,scratch,gui  \n! End of time history save " ("字符串")) -> (w955:string)
        n174 = Write to Text File(file (use dialog)=w956, text=w955) -> ()  [unwired: 2 in, 3 out]
      }
      event "前一张": Value Change {
        n175 = event-data() -> ()  [unwired: 1 in, 6 out]
        n176 = flat-sequence {
          frame #0 {
            n177 = local read "数值"() -> (w958:dbl)
            n178 = case shown="0" w958 {
              selector: w958 -> [w960 w963]
              tunnel: [w959 w961] -> w957
              frame 1..14, Default {
                n179 = Decrement(x=w960) -> (x-1=w959:i32)
              }
              frame 0 {
                n180 = Add(x=w963, y=14) -> (x+y=w961:i32)
              }
            }
            n181 = local write "数值"(w957) -> ()
          }
          frame #1 {
            n182 = local read "数值"() -> (w964:dbl)
            n183 = case shown="0..9" w964 {
              selector: w964 -> [w973 w977]
              tunnel: [w974 w976] -> w971
              frame 0..9 {
                n184 = Number To Decimal String(number=w973) -> (decimal integer string=w972:string)  [unwired: 1 in]
                n185 = Concatenate Strings("0" ("字符串"), w972) -> (w974:string)
              }
              frame 10..14, Default {
                n186 = Number To Decimal String(number=w977) -> (decimal integer string=w976:string)  [unwired: 1 in]
              }
            }
            n187 = Concatenate Strings("E:\\6546\\finaltest0", w971, ".jpg" ("字符串")) -> (w968:string)
            n188 = String To Path(string=w968) -> (path=w967:path)
            n189 = call <vilib>:"Read JPEG File.vi"("path to JPEG file"=w967) -> ("image data"=w969:T3)  [unwired: 8 in, 2 out]
            n190 = call <vilib>:"Draw Flattened Pixmap.vi"("image data"=w969) -> ("new picture"=w965:picture)  [unwired: 8 in]
            n191 = local write "new picture"(w965) -> ()
          }
        }
      }
    }
  }
